vi "CF _new.vi"() -> ()   [LabVIEW 2013]
uses:
  PEM/Labview Driver, PEM100, Rev 1.2/PEM100_Visa_rev1.2.llb/HindsPEM100_Setup.ctl
  PEM/Labview Driver, PEM100, Rev 1.2/PEM100_Visa_rev1.2.llb/Com Address.ctl
  <vilib>/DAQmx/read.llb/DAQmx Read (Analog 1D DBL NChan 1Samp).vi
  <vilib>/DAQmx/write.llb/DAQmx Write (Analog 1D DBL NChan 1Samp).vi
  <vilib>/DAQmx/write.llb/DAQmx Write (Analog 2D DBL NChan NSamp).vi
  <vilib>/DAQmx/read.llb/DAQmx Read (Analog 2D DBL NChan NSamp).vi
  <vilib>/Analysis/baseanly.llb/Mean (DBL).vi
  <vilib>/DAQmx/write.llb/DAQmx Write (Analog DBL 1Chan 1Samp).vi
  <vilib>/DAQmx/read.llb/DAQmx Read (Analog 1D DBL 1Chan NSamp).vi
  <vilib>/Utility/file.llb/Read From Spreadsheet File (DBL).vi
  <vilib>/DAQmx/create/channels.llb/DAQmx Create Channel (AI-Voltage-Basic).vi
  <vilib>/DAQmx/create/channels.llb/DAQmx Create Channel (AO-Voltage-Basic).vi
  <vilib>/DAQmx/configure/timing.llb/DAQmx Timing (Sample Clock).vi
  <vilib>/DAQmx/miscellaneous.llb/DAQmx Fill In Error Info.vi
  <vilib>/DAQmx/configure/trigger.llb/DAQmx Start Trigger (Digital Edge).vi
  <vilib>/Utility/file.llb/Write To Spreadsheet File (DBL).vi
  <vilib>/measure/NI_MABase.lvlib
  <resource>/objmgr/daqmx.rc
  <vilib>/Analysis/NI_AALBase.lvlib
panel:
  in  "Static Channels":cluster{dbl, string, "Output Channels":tag}[](array[cluster])=[{1.0, "", "Output Channels"="Dev1/ao2"}, {1.0, "", "Output Channels"="Dev1/ao3"}, {1.0, "", "Output Channels"="Dev2/ao2"}, {1.0, "", "Output Channels"="Dev2/ao3"}, {0.0, "", "Output Channels"=""}, {1.0, "", "Output Channels"=""}]
  out "IR Power":dbl[][](array[numeric])=[[0.3898, 5.617e-05, 1000.0], [2.02, 0.0002739, 1010.0], [2.025, 0.0002537, 1020.0], [1.748, 0.0002412, 1030.0], [1.884, 0.0003115, 1040.0], [1.752, 0.000412, 1050.0], [2.034, 0.0004784, 1060.0], [2.031, 0.0003652, 1070.0], [2.155, 0.000355, 1080.0], [1.988, 0.0003222, 1090.0], [1.864, 0.0003151, 1100.0], [1.733, 0.000293, 1110.0], [1.546, 0.0002614, 1120.0], [1.43, 0.0002417, 1130.0], [1.423, 0.0002405, 1140.0], [1.513, 0.0002557, 1150.0], [1.694, 0.0002862, 1160.0], [1.907, 0.0003223, 1170.0], [2.124, 0.0003589, 1180.0], [2.278, 0.000385, 1190.0], [2.277, 0.0003847, 1200.0], [2.144, 0.0003621, 1210.0], [1.986, 0.0003355, 1220.0], [1.898, 0.0003205, 1230.0], [1.925, 0.0003252, 1240.0], [2.034, 0.0003435, 1250.0], [2.127, 0.0003592, 1260.0], [2.211, 0.0003733, 1270.0], [2.244, 0.0003788, 1280.0], [2.232, 0.0003768, 1290.0], [2.217, 0.0003743, 1300.0], [2.274, 0.0003838, 1310.0], [2.371, 0.0004002, 1320.0], [2.499, 0.0004217, 1330.0], [2.694, 0.0004546, 1340.0], [2.607, 0.0004399, 1350.0], [2.198, 0.0003709, 1360.0], [1.699, 0.0002866, 1370.0], [1.275, 0.0002151, 1380.0], [1.552, 0.0002617, 1390.0], [1.766, 0.0002977, 1400.0], [2.054, 0.0003464, 1410.0], [2.374, 0.0004003, 1420.0], [2.643, 0.0004456, 1430.0], [2.718, 0.0004583, 1440.0], [2.547, 0.0004293, 1450.0], [2.195, 0.00037, 1460.0], [1.875, 0.000316, 1470.0], [1.72, 0.0002899, 1480.0], [1.676, 0.0002824, 1490.0], [1.736, 0.0002925, 1500.0], [1.805, 0.0003041, 1510.0], [1.929, 0.0003249, 1520.0], [2.082, 0.0003507, 1530.0], [2.283, 0.0003845, 1540.0], [2.517, 0.0004239, 1550.0], [2.698, 0.0004544, 1560.0], [2.772, 0.0004668, 1570.0], [2.674, 0.0004501, 1580.0], [2.529, 0.0004257, 1590.0], [2.338, 0.0003936, 1600.0], [2.127, 0.000358, 1610.0], [1.947, 0.0003277, 1620.0], [1.752, 0.0002948, 1630.0], [1.552, 0.0002612, 1640.0], [1.388, 0.0002335, 1650.0], [1.207, 0.0002031, 1660.0], [1.019, 0.0001714, 1670.0], [0.9422, 0.0001585, 1680.0], [0.8635, 0.0001452, 1690.0], [0.8028, 0.000135, 1700.0], [0.7895, 0.0001328, 1710.0], [0.7496, 0.000126, 1720.0], [0.7109, 0.0001195, 1730.0], [0.6709, 0.0001128, 1740.0], [0.6361, 0.0001069, 1750.0], [0.586, 9.849e-05, 1760.0], [0.5324, 8.947e-05, 1770.0], [0.472, 7.932e-05, 1780.0], [0.4092, 6.875e-05, 1790.0], [0.3409, 5.728e-05, 1800.0]]
  out "Vis Power":dbl[][](array[numeric])=[[1.246, 2.318e-05, 400.0], [1.183, 0.0001042, 405.0], [0.7058, 0.0001228, 410.0], [0.957, 3.031e-05, 415.0], [0.9707, 5.607e-05, 420.0], [0.9509, 9.291e-05, 425.0], [0.9652, 0.0001411, 430.0], [0.9779, 0.000182, 435.0], [1.003, 0.0001974, 440.0], [1.041, 0.0002096, 445.0], [1.028, 0.0002025, 450.0], [1.052, 0.0001774, 455.0], [1.04, 0.0001549, 460.0], [1.031, 0.0001442, 465.0], [1.076, 0.0001512, 470.0], [1.072, 0.0001558, 475.0], [1.077, 0.0001726, 480.0], [1.077, 0.000155, 485.0], [1.051, 0.0001677, 490.0], [1.085, 0.0001761, 495.0], [1.075, 0.0002017, 500.0], [1.039, 0.0002081, 505.0], [1.025, 0.0002273, 510.0], [1.01, 0.0002913, 515.0], [1.017, 0.0002703, 520.0], [1.009, 0.0002942, 525.0], [0.9843, 0.0002796, 530.0], [1.004, 0.0002957, 535.0], [0.9771, 0.0003261, 540.0], [0.9818, 0.0003368, 545.0], [0.9802, 0.0003446, 550.0], [0.9463, 0.0003474, 555.0], [0.9541, 0.0003665, 560.0], [0.9389, 0.0003327, 565.0], [0.9278, 0.0003475, 570.0], [0.9343, 0.0003765, 575.0], [0.9392, 0.000404, 580.0], [0.9248, 0.0004213, 585.0], [0.9276, 0.0004463, 590.0], [0.9301, 0.0004129, 595.0], [0.938, 0.0003926, 600.0], [0.9261, 0.0004247, 605.0], [0.9214, 0.0004545, 610.0], [0.9264, 0.0004519, 615.0], [0.9205, 0.0004481, 620.0], [0.9071, 0.0004037, 625.0], [0.9085, 0.0004188, 630.0], [0.9135, 0.0004314, 635.0], [0.919, 0.0004155, 640.0], [0.9358, 0.0004483, 645.0], [0.9164, 0.0004434, 650.0], [0.9342, 0.0004245, 655.0], [0.9412, 0.0004252, 660.0], [0.9544, 0.0004259, 665.0], [0.9549, 0.0004423, 670.0], [0.9525, 0.0004703, 675.0], [0.9531, 0.0005061, 680.0], [0.9534, 0.0005373, 685.0], [0.9538, 0.0005706, 690.0], [0.9623, 0.0005955, 695.0], [0.9587, 0.0006049, 700.0], [0.9643, 0.0005917, 705.0], [0.9702, 0.0005094, 710.0], [0.9857, 0.0004327, 715.0], [0.9781, 0.0004413, 720.0], [0.9567, 0.0004771, 725.0], [0.9459, 0.0004635, 730.0], [0.9418, 0.0004453, 735.0], [0.9456, 0.0004497, 740.0], [0.9608, 0.0004574, 745.0], [0.953, 0.0004442, 750.0], [0.9723, 0.000451, 755.0], [0.9896, 0.0004518, 760.0], [0.996, 0.0004485, 765.0], [1.001, 0.0004247, 770.0], [1.007, 0.0003865, 775.0], [1.016, 0.0003508, 780.0], [1.035, 0.0003404, 785.0], [1.031, 0.0003623, 790.0], [1.027, 0.0003991, 795.0], [1.018, 0.0004293, 800.0], [1.02, 0.0004557, 805.0], [1.028, 0.0004573, 810.0], [1.023, 0.0004482, 815.0], [1.018, 0.0004471, 820.0], [1.006, 0.0004426, 825.0], [1.005, 0.0004233, 830.0], [1.01, 0.0003991, 835.0], [1.009, 0.000391, 840.0], [1.001, 0.0004016, 845.0], [0.9936, 0.0004036, 850.0], [0.9817, 0.0003871, 855.0], [0.98, 0.0003447, 860.0], [0.989, 0.0003386, 865.0], [0.9676, 0.0003372, 870.0], [0.9529, 0.0003146, 875.0], [0.96, 0.0003173, 880.0], [0.9574, 0.0002994, 885.0], [0.9534, 0.000297, 890.0], [0.9416, 0.0002885, 895.0], [0.9526, 0.0002831, 900.0], [0.9407, 0.0002601, 905.0], [0.9437, 0.000248, 910.0], [0.9327, 0.0002356, 915.0], [0.9274, 0.0002234, 920.0], [0.93, 0.0002134, 925.0], [0.9262, 0.0002018, 930.0], [0.9292, 0.0001934, 935.0], [0.937, 0.0001986, 940.0], [0.9274, 0.0002188, 945.0], [0.9187, 0.0002472, 950.0], [0.919, 0.0002798, 955.0], [0.9199, 0.0002845, 960.0], [0.9228, 0.0002559, 965.0], [0.9247, 0.0002169, 970.0], [0.9264, 0.0001847, 975.0], [0.9249, 0.0001615, 980.0], [0.9245, 0.0001469, 985.0], [0.9239, 0.0001402, 990.0], [0.9154, 0.0001357, 995.0], [0.9124, 0.0001315, 1000.0]]
  in  "Normalizing power IR":path=path "T:/Physics/Minot Group/Lee/SPCM/Power waves/2015-02-05/PowIRnewconfig"
  in  "Normalizing power visible":path=path "T:/Physics/Minot Group/Lee/SPCM/Power waves/2015-02-05/Powvis"
  out "Record Start":timestamp=timestamp(3554067343.4700146 s since 1904-01-01)
  in  "Sm Voltage offset x":dbl=0.0056
  in  "Sm voltage offset y":dbl=0.0064
  out "VNTy":dbl=-0.002731286355015208
  out "VNTx":dbl=0.0019385044089532365
  in  "Use PEM?":bool
  out "PEM delay":dbl=2.0442256927490234
  in  "PEM100Setup":T1={"Address:"=0, "Retardation:"=0.25, "RTD Units"=0, "Wavelength:"=1010.0, "Wave Units"=0} {"Address:" items=["Com 1", "Com 2", "Com 3", "Com 4", "Com 5", "Com 6", "Com 7", "Com 8", "Com 9", "Com 10"]; "Wave Units" items=["nm", "um", "cm-1"]; "RTD Units" items=["waves", "Radians", "Degrees"]; "Wavelength:" min=0.0 max=19999.9 step=0.1 format="%.1f"; "Retardation:" min=0.0 max=10.0 step=0.001 format="%.3f"}
  in  "Scan base":path=path "T:/Physics/Minot Group/Lee/SPCM"
  in  "Prepend date folder?":bool=TRUE
  in  "Subfolder(no outside slashes)":string
  in  "Volts/pixel y":dbl=-0.041
  in  "Volts/pixel  x":dbl=0.041
  out "String":string="IR Grating"
  in  "IR Grating Correction":dbl[][](array[numeric])=[[1000.0, 0.0, 0.0], [1100.0, 0.0, -0.06], [1200.0, -0.01, 0.06], [1300.0, 0.06, 0.02], [1400.0, -0.05, 0.05], [1500.0, 0.0, 0.0], [1600.0, 0.0, 0.0], [1700.0, 0.0, 0.0], [1800.0, 0.0, 0.0]]
  in  "Reset Positioned wavelength?":bool
  out "Done?":string="  ok\r\n"
  out "Busy?":bool
  out "Reply":string=" 619.990 nm  ok\r\n" caption="Mono Response"
  in  "Speed (nm/min)":dbl=100.0 min=1.0 max=500.0 step=0.1 format="%.1f"
  in  "Wavelength:":dbl=620.0 caption="nm" min=0.0 max=2000.0 step=0.1 format="%.1f"
  in  "Positioned Wavelength":dbl=1600.0
  in  "Sm Correction?":bool=TRUE
  out "Delta Pix y":dbl=-0.006
  out "delta pix x":dbl
  in  "Power Meter Initalized?":bool
  out "Multiplication Factor":dbl=1e-09
  in  "Preamp Sensitivity":T3(ring)=enum."1nA/V"
  in  "Configuration":T4(ring)=enum."Preamp"
  in  "Multiply Data?":bool=TRUE
  out "Waveform Chart  Y":dbl[](graph)=[-0.006278594561464471, -0.0062748012532580204, -0.006271007945051572, -0.006267214636845122, -0.0062634213286386735, -0.006259628020432223, -0.006255834712225775, -0.006252041404019325, -0.006248248095812876, -0.006244454787606426, -0.006240661479399978, -0.006236868171193528, -0.006233074862987079, -0.006229281554780629, -0.006225488246574181, -0.006221694938367731, -0.006217901630161282, -0.006214108321954833, -0.006210315013748384, -0.006206521705541934, -0.006202728397335485, -0.006198935089129036, -0.0061951417809225865, -0.006191348472716137, -0.006187555164509688, -0.006183761856303239, -0.006179968548096789, -0.00617617523989034, -0.006172381931683891, -0.006168588623477442, -0.006164795315270992, -0.006161002007064543, -0.006157208698858094, -0.0061534153906516445, -0.006149622082445195, -0.006145828774238746, -0.006142035466032297, -0.006138242157825847, -0.006134448849619398, -0.006130655541412949, -0.0061268622332064995, -0.00612306892500005, -0.006119275616793601, -0.006115482308587152, -0.006111689000380702, -0.006107895692174253, -0.006104102383967804, -0.006100309075761355, -0.006096515767554905, -0.006092722459348457, -0.006088929151142007, -0.0060851358429355575, -0.006081342534729108, -0.006077549226522659, -0.00607375591831621, -0.00606996261010976, -0.006066169301903311, -0.006062375993696862, -0.0060585826854904126, -0.006054789377283963, -0.006050996069077514, -0.006047202760871065, -0.0060434094526646154, -0.006039616144458167, -0.006035822836251717, -0.0060320295280452685, -0.006028236219838819, -0.00602444291163237, -0.006020649603425921, -0.006016856295219471, -0.006013062987013022, -0.006009269678806573, -0.0060054763706001235, -0.006001683062393674, -0.005997889754187225, -0.005994096445980776, -0.005990303137774326, -0.005986509829567877, -0.005982716521361427, -0.005978923213154979, -0.005975129904948529, -0.00597133659674208, -0.005967543288535631, -0.0059637499803291815, -0.005959956672122732, -0.005956163363916283, -0.005952370055709834, -0.005948576747503384, -0.005944783439296935, -0.005940990131090486, -0.005937196822884037, -0.005933403514677587, -0.005929610206471138, -0.005925816898264689, -0.0059220235900582395, -0.00591823028185179, -0.005914436973645341, -0.005910643665438892, -0.005906850357232442, -0.005903057049025993, -0.005899263740819544, -0.0058954704326130945, -0.005891677124406645, -0.005887883816200196, -0.005884090507993747, -0.005880297199787297, -0.005876503891580848, -0.005872710583374399, -0.00586891727516795, -0.0058651239669615, -0.005861330658755051, -0.005857537350548602, -0.005853744042342153, -0.005849950734135703, -0.005846157425929255, -0.005842364117722805, -0.005838570809516356, -0.005834777501309906, -0.005830984193103458, -0.0058271908848970076, -0.005823397576690559, -0.005819604268484109, -0.005815810960277661, -0.0058120176520712104, -0.005808224343864761, -0.005804431035658312, -0.005800637727451863, -0.005796844419245413, -0.005793051111038965, -0.005789257802832515, -0.005785464494626066, -0.005781671186419617, -0.005777877878213168, -0.0057740845700067185, -0.005770291261800269, -0.00576649795359382, -0.005762704645387371, -0.0057589113371809214, -0.005755118028974472, -0.005751324720768023, -0.005747531412561574, -0.005743738104355124, -0.005739944796148675, -0.005736151487942226, -0.0057323581797357765, -0.005728564871529327, -0.005724771563322878, -0.005720978255116429, -0.005717184946909979, -0.00571339163870353, -0.005709598330497081, -0.005705805022290632, -0.005702011714084182, -0.005698218405877733, -0.005694425097671284, -0.0056906317894648345, -0.005686838481258385, -0.005683045173051936, -0.005679251864845487, -0.005675458556639037, -0.005671665248432588, -0.005667871940226139, -0.0056640786320196895, -0.00566028532381324, -0.005656492015606791, -0.005652698707400342, -0.005648905399193892, -0.005645112090987443, -0.005641318782780994, -0.005637525474574545, -0.005633732166368095, -0.005629938858161646, -0.005626145549955197, -0.0056223522417487475, -0.005618558933542298, -0.005614765625335849, -0.0056109723171294, -0.005607179008922951, -0.005603385700716501, -0.005599592392510053, -0.0055957990843036026, -0.005592005776097154, -0.005588212467890704, -0.005584419159684256, -0.0055806258514778054, -0.005576832543271357, -0.005573039235064907, -0.0055692459268584585, -0.005565452618652008, -0.00556165931044556, -0.00555786600223911, -0.005554072694032661, -0.005550279385826211, -0.005546486077619763, -0.0055426927694133135, -0.005538899461206864, -0.005535106153000415, -0.005531312844793966, -0.0055275195365875164, -0.005523726228381067, -0.005519932920174618, -0.005516139611968169, -0.005512346303761719, -0.00550855299555527, -0.005504759687348821, -0.0055009663791423715, -0.005497173070935922, -0.005493379762729473, -0.005489586454523024, -0.005485793146316574, -0.005481999838110125, -0.005478206529903676, -0.005474413221697227, -0.005470619913490777, -0.005466826605284328, -0.005463033297077879, -0.0054592399888714295, -0.00545544668066498, -0.005451653372458531, -0.005447860064252082, -0.005444066756045632, -0.005440273447839183, -0.005436480139632734, -0.0054326868314262845, -0.005428893523219835, -0.005425100215013386, -0.005421306906806937, -0.005417513598600487, -0.005413720290394039, -0.005409926982187589, -0.00540613367398114, -0.00540234036577469, -0.005398547057568242, -0.005394753749361792, -0.0053909604411553425, -0.005387167132948893, -0.005383373824742445, -0.005379580516535995, -0.005375787208329545, -0.005371993900123096, -0.005368200591916648, -0.0053644072837101976, -0.005360613975503749, -0.005356820667297299, -0.005353027359090851, -0.005349234050884401, -0.005345440742677952, -0.005341647434471502, -0.005337854126265053, -0.005334060818058604, -0.005330267509852155, -0.005326474201645705, -0.0053226808934392555, -0.005318887585232807, -0.005315094277026358, -0.0053113009688199085, -0.005307507660613458, -0.00530371435240701, -0.005299921044200561, -0.0052961277359941114, -0.005292334427787662, -0.005288541119581213, -0.005284747811374764, -0.005280954503168314, -0.005277161194961865, -0.005273367886755416, -0.0052695745785489665, -0.005265781270342517, -0.005261987962136068, -0.005258194653929619, -0.005254401345723169, -0.00525060803751672, -0.005246814729310271, -0.005243021421103822, -0.005239228112897372, -0.005235434804690923, -0.005231641496484474, -0.0052278481882780245, -0.005224054880071575, -0.005220261571865126, -0.005216468263658677, -0.005212674955452227, -0.005208881647245778, -0.005205088339039329, -0.0052012950308328795, -0.00519750172262643, -0.005193708414419981, -0.005189915106213532, -0.005186121798007082, -0.005182328489800633, -0.005178535181594185, -0.005174741873387735, -0.005170948565181285, -0.005167155256974836, -0.005163361948768388, -0.005159568640561938, -0.005155775332355488, -0.005151982024149039, -0.00514818871594259, -0.005144395407736141, -0.005140602099529691, -0.005136808791323242, -0.0051330154831167926, -0.005129222174910344, -0.005125428866703894, -0.005121635558497445, -0.0051178422502909954, -0.005114048942084547, -0.005110255633878098, -0.0051064623256716485, -0.005102669017465198, -0.00509887570925875, -0.005095082401052301, -0.005091289092845851, -0.005087495784639401, -0.005083702476432953, -0.0050799091682265035, -0.005076115860020054, -0.005072322551813604, -0.005068529243607156, -0.0050647359354007064, -0.005060942627194257, -0.005057149318987808, -0.005053356010781359, -0.005049562702574909, -0.00504576939436846, -0.005041976086162011, -0.0050381827779555615, -0.005034389469749112, -0.005030596161542663, -0.005026802853336214, -0.005023009545129764, -0.005019216236923315, -0.005015422928716866, -0.005011629620510417, -0.005007836312303967, -0.005004043004097518, -0.005000249695891069, -0.0049964563876846195, -0.00499266307947817, -0.004988869771271721, -0.004985076463065272, -0.004981283154858822, -0.004977489846652373, -0.004973696538445925, -0.0049699032302394745, -0.004966109922033025, -0.004962316613826576, -0.004958523305620127, -0.004954729997413677, -0.004950936689207228, -0.004947143381000779, -0.00494335007279433, -0.00493955676458788, -0.004935763456381431, -0.004931970148174982, -0.0049281768399685325, -0.004924383531762084, -0.004920590223555635, -0.004916796915349185, -0.004913003607142735, -0.004909210298936287, -0.004905416990729838, -0.0049016236825233876, -0.004897830374316938, -0.00489403706611049, -0.004890243757904041, -0.0048864504496975904, -0.004882657141491141, -0.004878863833284693, -0.0048750705250782435, -0.004871277216871794, -0.004867483908665345, -0.004863690600458895, -0.004859897292252446, -0.004856103984045997, -0.004852310675839548, -0.004848517367633098, -0.004844724059426649, -0.0048409307512202, -0.004837137443013751, -0.004833344134807301, -0.004829550826600852, -0.004825757518394403, -0.004821964210187954, -0.004818170901981504, -0.004814377593775055, -0.004810584285568606, -0.0048067909773621565, -0.004802997669155707, -0.004799204360949258, -0.004795411052742809, -0.004791617744536359, -0.00478782443632991, -0.004784031128123461, -0.004780237819917012, -0.004776444511710562, -0.004772651203504113, -0.004768857895297664, -0.0047650645870912145, -0.004761271278884765, -0.004757477970678316, -0.004753684662471867, -0.004749891354265417, -0.004746098046058968, -0.004742304737852519, -0.0047385114296460695, -0.004734718121439621, -0.004730924813233171, -0.004727131505026722, -0.004723338196820272, -0.004719544888613824, -0.004715751580407374, -0.004711958272200925, -0.004708164963994475, -0.004704371655788027, -0.004700578347581577, -0.0046967850393751275, -0.004692991731168678, -0.00468919842296223, -0.0046854051147557805, -0.004681611806549331, -0.004677818498342881, -0.004674025190136432, -0.004670231881929983, -0.004666438573723534, -0.004662645265517084, -0.004658851957310635, -0.004655058649104186, -0.004651265340897737, -0.004647472032691287, -0.004643678724484838, -0.004639885416278389, -0.00463609210807194, -0.004632298799865491, -0.0046285054916590405, -0.004624712183452592, -0.004620918875246143, -0.0046171255670396935, -0.004613332258833244, -0.004609538950626795, -0.004605745642420346, -0.0046019523342138964, -0.004598159026007447, -0.004594365717800998, -0.004590572409594549, -0.004586779101388099, -0.00458298579318165, -0.004579192484975201, -0.0045753991767687515, -0.004571605868562302, -0.004567812560355853, -0.004564019252149404, -0.004560225943942954, -0.004556432635736505, -0.004552639327530056, -0.004548846019323607, -0.004545052711117157, -0.004541259402910708, -0.004537466094704259, -0.0045336727864978095, -0.00452987947829136, -0.004526086170084911, -0.004522292861878462, -0.004518499553672012, -0.004514706245465564, -0.004510912937259114, -0.0045071196290526645, -0.004503326320846215, -0.004499533012639766, -0.004495739704433317, -0.004491946396226867, -0.004488153088020418, -0.004484359779813969, -0.0044805664716075205, -0.00447677316340107, -0.004472979855194621, -0.004469186546988172, -0.004465393238781723, -0.004461599930575273, -0.004457806622368824, -0.004454013314162375, -0.004450220005955926, -0.004446426697749477, -0.004442633389543027, -0.0044388400813365776, -0.004435046773130129, -0.00443125346492368, -0.004427460156717231, -0.0044236668485107804, -0.004419873540304332, -0.004416080232097883, -0.0044122869238914335, -0.004408493615684983, -0.004404700307478534, -0.004400906999272086, -0.004397113691065636, -0.004393320382859187, -0.004389527074652737, -0.0043857337664462885, -0.004381940458239839, -0.00437814715003339, -0.004374353841826941, -0.0043705605336204914, -0.004366767225414042, -0.004362973917207593, -0.004359180609001144, -0.004355387300794694, -0.004351593992588245, -0.004347800684381796, -0.0043440073761753465, -0.004340214067968897, -0.004336420759762448, -0.004332627451555999, -0.004328834143349549, -0.004325040835143101, -0.004321247526936651, -0.004317454218730202, -0.004313660910523752, -0.004309867602317303, -0.004306074294110854, -0.0043022809859044045, -0.004298487677697955, -0.004294694369491506, -0.0042909010612850575, -0.004287107753078607, -0.004283314444872158, -0.004279521136665709, -0.00427572782845926, -0.004271934520252811, -0.004268141212046361, -0.004264347903839912, -0.004260554595633463, -0.004256761287427014, -0.004252967979220564, -0.004249174671014115, -0.004245381362807666, -0.004241588054601217, -0.004237794746394768, -0.0042340014381883175, -0.004230208129981869, -0.00422641482177542, -0.0042226215135689705, -0.004218828205362521, -0.004215034897156071, -0.004211241588949623, -0.004207448280743173, -0.004203654972536724, -0.004199861664330274, -0.004196068356123826, -0.004192275047917376, -0.004188481739710927, -0.004184688431504478, -0.0041808951232980285, -0.004177101815091579, -0.00417330850688513, -0.004169515198678681, -0.004165721890472231, -0.004161928582265782, -0.004158135274059333, -0.0041543419658528835, -0.004150548657646434, -0.004146755349439985, -0.004142962041233536, -0.0041391687330270864, -0.004135375424820637, -0.004131582116614188, -0.004127788808407739, -0.004123995500201289, -0.00412020219199484, -0.004116408883788391, -0.0041126155755819415, -0.004108822267375492, -0.004105028959169043, -0.004101235650962594, -0.004097442342756144, -0.004093649034549695, -0.004089855726343246, -0.0040860624181367974, -0.004082269109930347, -0.004078475801723898, -0.004074682493517449, -0.004070889185311, -0.00406709587710455, -0.004063302568898101, -0.004059509260691652, -0.004055715952485203, -0.004051922644278754, -0.004048129336072304, -0.0040443360278658545, -0.004040542719659406, -0.004036749411452957, -0.0040329561032465076, -0.004029162795040057, -0.004025369486833608, -0.00402157617862716, -0.0040177828704207105, -0.00401398956221426, -0.004010196254007811, -0.004006402945801363, -0.004002609637594913, -0.003998816329388464, -0.003995023021182014, -0.0039912297129755655, -0.003987436404769116, -0.003983643096562667, -0.003979849788356218, -0.003976056480149768, -0.003972263171943319, -0.00396846986373687, -0.003964676555530421, -0.003960883247323971, -0.003957089939117522, -0.003953296630911073, -0.0039495033227046235, -0.003945710014498174, -0.003941916706291725, -0.003938123398085276, -0.003934330089878826, -0.003930536781672377, -0.003926743473465928, -0.0039229501652594785, -0.003919156857053029, -0.00391536354884658, -0.003911570240640131, -0.0039077769324336814, -0.003903983624227232, -0.003900190316020783, -0.003896397007814334, -0.0038926036996078843, -0.003888810391401435, -0.0038850170831949858, -0.003881223774988537, -0.0038774304667820872, -0.003873637158575638, -0.0038698438503691887, -0.00386605054216274, -0.0038622572339562906, -0.003858463925749841, -0.0038546706175433916, -0.0038508773093369427, -0.0038470840011304934, -0.003843290692924044, -0.0038394973847175945, -0.003835704076511145, -0.0038319107683046963, -0.003828117460098247, -0.0038243241518917974, -0.003820530843685348, -0.0038167375354788992, -0.00381294422727245, -0.0038091509190660007, -0.003805357610859551, -0.0038015643026531026, -0.003797770994446653, -0.0037939776862402036, -0.0037901843780337543, -0.0037863910698273055, -0.003782597761620856, -0.0037788044534144065, -0.003775011145207957, -0.0037712178370015084, -0.003767424528795059, -0.0037636312205886094, -0.00375983791238216, -0.0037560446041757112, -0.003752251295969262, -0.0037484579877628127, -0.003744664679556363, -0.0037408713713499137, -0.003737078063143465, -0.0037332847549370156, -0.0037294914467305663, -0.0037256981385241166, -0.0037219048303176678, -0.0037181115221112185, -0.003714318213904769, -0.0037105249056983195, -0.0037067315974918707, -0.0037029382892854214, -0.003699144981078972, -0.003695351672872523, -0.0036915583646660735, -0.0036877650564596243, -0.003683971748253175, -0.0036801784400467257, -0.003676385131840277, -0.003672591823633827, -0.003668798515427378, -0.0036650052072209286, -0.0036612118990144798, -0.0036574185908080305, -0.0036536252826015808, -0.0036498319743951315, -0.0036460386661886822, -0.0036422453579822334, -0.0036384520497757837, -0.0036346587415693344, -0.003630865433362885, -0.0036270721251564363, -0.003623278816949987, -0.0036194855087435373, -0.003615692200537088, -0.003611898892330639, -0.00360810558412419, -0.0036043122759177406, -0.003600518967711291, -0.0035967256595048425, -0.003592932351298393, -0.0035891390430919435, -0.003585345734885494, -0.0035815524266790454, -0.0035777591184725957, -0.0035739658102661464, -0.003570172502059697, -0.0035663791938532483, -0.003562585885646799, -0.0035587925774403493, -0.0035549992692339, -0.0035512059610274503, -0.003547412652821002, -0.0035436193446145526, -0.003539826036408103, -0.0035360327282016536, -0.003532239419995205, -0.0035284461117887555, -0.003524652803582306, -0.0035208594953758565, -0.0035170661871694077, -0.0035132728789629584, -0.003509479570756509, -0.0035056862625500594, -0.0035018929543436106, -0.0034980996461371613, -0.003494306337930712, -0.0034905130297242623, -0.0034867197215178135, -0.003482926413311364, -0.003479133105104915, -0.0034753397968984657, -0.003471546488692017, -0.003467753180485567, -0.003463959872279118, -0.0034601665640726685, -0.0034563732558662193, -0.00345257994765977, -0.0034487866394533207, -0.0034449933312468714, -0.003441200023040422, -0.0034374067148339733, -0.0034336134066275236, -0.0034298200984210743, -0.003426026790214625, -0.003422233482008176, -0.0034184401738017265, -0.0034146468655952772, -0.003410853557388828, -0.003407060249182379, -0.00340326694097593, -0.00339947363276948, -0.003395680324563031, -0.0033918870163565824, -0.0033880937081501327, -0.003384300399943683, -0.0033805070917372337, -0.0033767137835307845, -0.0033729204753243356, -0.0033691271671178863, -0.0033653338589114366, -0.0033615405507049874, -0.003357747242498539, -0.0033539539342920892, -0.00335016062608564, -0.0033463673178791902, -0.003342574009672742, -0.0033387807014662926, -0.003334987393259843, -0.003331194085053393, -0.0033274007768469447, -0.0033236074686404955, -0.0033198141604340457, -0.0033160208522275965, -0.0033122275440211476, -0.0033084342358146984, -0.003304640927608249, -0.0033008476194017994, -0.0032970543111953505, -0.0032932610029889012, -0.003289467694782452, -0.0032856743865760023, -0.003281881078369553, -0.003278087770163104, -0.003274294461956655, -0.0032705011537502056, -0.003266707845543756, -0.003262914537337307, -0.0032591212291308578, -0.0032553279209244085, -0.003251534612717959, -0.00324774130451151, -0.0032439479963050607, -0.0032401546880986114, -0.003236361379892162, -0.003232568071685713, -0.0032287747634792635, -0.0032249814552728143, -0.003221188147066365, -0.003217394838859916, -0.0032136015306534664, -0.003209808222447017, -0.003206014914240568, -0.003202221606034119, -0.0031984282978276693, -0.00319463498962122, -0.0031908416814147708, -0.0031870483732083215, -0.0031832550650018727, -0.003179461756795423, -0.0031756684485889737, -0.0031718751403825244, -0.0031680818321760756, -0.0031642885239696263, -0.0031604952157631766, -0.0031567019075567273, -0.0031529085993502784, -0.003149115291143829, -0.0031453219829373795, -0.00314152867473093, -0.0031377353665244818, -0.003133942058318032, -0.003130148750111583, -0.003126355441905133, -0.0031225621336986847, -0.0031187688254922354, -0.0031149755172857857, -0.003111182209079336, -0.0031073889008728876, -0.0031035955926664383, -0.0030998022844599886, -0.0030960089762535393, -0.0030922156680470896, -0.003088422359840641, -0.003084629051634192, -0.003080835743427742, -0.003077042435221293, -0.003073249127014844, -0.003069455818808395, -0.0030656625106019455, -0.003061869202395496, -0.003058075894189047, -0.0030542825859825977, -0.0030504892777761484, -0.0030466959695696987, -0.00304290266136325, -0.0030391093531568006, -0.0030353160449503513, -0.003031522736743902, -0.0030277294285374528, -0.0030239361203310035, -0.003020142812124554, -0.003016349503918105, -0.0030125561957116557, -0.0030087628875052064, -0.003004969579298757, -0.003001176271092308, -0.0029973829628858585, -0.0029935896546794093, -0.00298979634647296, -0.0029860030382665107, -0.0029822097300600614, -0.002978416421853612, -0.002974623113647163, -0.0029708298054407136, -0.0029670364972342643, -0.0029632431890278155, -0.0029594498808213658, -0.0029556565726149165, -0.0029518632644084672, -0.0029480699562020184, -0.002944276647995569, -0.0029404833397891194, -0.00293669003158267, -0.0029328967233762217, -0.002929103415169772, -0.0029253101069633223, -0.002921516798756873, -0.0029177234905504246, -0.002913930182343975, -0.0029101368741375256, -0.002906343565931076, -0.0029025502577246266, -0.0028987569495181782, -0.0028949636413117285, -0.0028911703331052792, -0.0028873770248988295, -0.002883583716692381, -0.002879790408485932, -0.002875997100279482, -0.0028722037920730324, -0.002868410483866584, -0.0028646171756601347, -0.002860823867453685, -0.0028570305592472357, -0.002853237251040787, -0.0028494439428343376, -0.0028456506346278884, -0.0028418573264214386, -0.00283806401821499, -0.0028342707100085405, -0.0028304774018020912, -0.002826684093595642, -0.0028228907853891927, -0.0028190974771827434, -0.002815304168976294, -0.002811510860769845, -0.002807717552563395, -0.0028039242443569463, -0.002800130936150497, -0.0027963376279440478, -0.0027925443197375985, -0.002788751011531149, -0.0027849577033247, -0.0027811643951182506, -0.002777371086911802, -0.002773577778705352, -0.002769784470498903, -0.0027659911622924535, -0.0027621978540860043, -0.002758404545879555, -0.0027546112376731053, -0.0027508179294666573, -0.002747024621260208, -0.0027432313130537583, -0.0027394380048473086, -0.0027356446966408593, -0.00273185138843441, -0.0027280580802279608, -0.0027242647720215115, -0.002720471463815062, -0.002716678155608614, -0.0027128848474021645, -0.002709091539195715, -0.0027052982309892656, -0.002701504922782816, -0.0026977116145763666, -0.0026939183063699173, -0.002690124998163468, -0.0026863316899570196, -0.0026825383817505703, -0.002678745073544121, -0.0026749517653376713, -0.002671158457131222, -0.0026673651489247724, -0.002663571840718323, -0.002659778532511874, -0.0026559852243054254, -0.002652191916098976, -0.002648398607892527, -0.0026446052996860776, -0.002640811991479628, -0.0026370186832731786, -0.002633225375066729, -0.0026294320668602796, -0.0026256387586538303, -0.002621845450447382, -0.0026180521422409326, -0.0026142588340344834, -0.002610465525828034, -0.002606672217621585, -0.002602878909415135, -0.0025990856012086854, -0.002595292293002236, -0.002591498984795788, -0.0025877056765893384, -0.002583912368382889, -0.00258011906017644, -0.0025763257519699906, -0.0025725324437635413, -0.0025687391355570916, -0.0025649458273506423, -0.0025611525191441943, -0.0025573592109377446, -0.002553565902731295, -0.0025497725945248456, -0.0025459792863183964, -0.002542185978111947, -0.002538392669905498, -0.002534599361699048, -0.002530806053492599, -0.002527012745286151, -0.002523219437079701, -0.002519426128873252, -0.002515632820666802, -0.002511839512460353, -0.0025080462042539036, -0.0025042528960474543, -0.002500459587841005, -0.0024966662796345566, -0.0024928729714281074, -0.0024890796632216577]
  out "Final Y":dbl=-0.0024890796632216577
  out "initial y":dbl=-0.006278594561464471
  out "Waveform Chart X":dbl[](graph)=[-0.005478594561464469, -0.005471177462494051, -0.005463760363523634, -0.005456343264553216, -0.005448926165582799, -0.00544150906661238, -0.005434091967641963, -0.0054266748686715455, -0.005419257769701128, -0.00541184067073071, -0.005404423571760292, -0.005397006472789874, -0.0053895893738194565, -0.005382172274849039, -0.005374755175878621, -0.005367338076908203, -0.005359920977937786, -0.005352503878967368, -0.005345086779996951, -0.005337669681026533, -0.005330252582056116, -0.005322835483085698, -0.00531541838411528, -0.005308001285144862, -0.0053005841861744445, -0.005293167087204027, -0.005285749988233609, -0.005278332889263191, -0.005270915790292773, -0.005263498691322355, -0.005256081592351938, -0.00524866449338152, -0.005241247394411102, -0.005233830295440685, -0.005226413196470267, -0.00521899609749985, -0.005211578998529432, -0.005204161899559015, -0.005196744800588597, -0.005189327701618179, -0.005181910602647761, -0.005174493503677343, -0.005167076404706926, -0.005159659305736508, -0.00515224220676609, -0.005144825107795672, -0.005137408008825254, -0.005129990909854837, -0.005122573810884419, -0.005115156711914002, -0.005107739612943584, -0.005100322513973166, -0.005092905415002748, -0.0050854883160323305, -0.0050780712170619136, -0.005070654118091496, -0.005063237019121078, -0.00505581992015066, -0.005048402821180242, -0.0050409857222098245, -0.005033568623239407, -0.005026151524268989, -0.005018734425298571, -0.005011317326328153, -0.005003900227357736, -0.004996483128387318, -0.004989066029416901, -0.004981648930446483, -0.004974231831476066, -0.004966814732505647, -0.00495939763353523, -0.0049519805345648125, -0.004944563435594395, -0.004937146336623977, -0.004929729237653559, -0.004922312138683141, -0.004914895039712723, -0.004907477940742306, -0.004900060841771888, -0.00489264374280147, -0.004885226643831052, -0.004877809544860635, -0.0048703924458902165, -0.0048629753469198, -0.004855558247949382, -0.004848141148978965, -0.004840724050008546, -0.004833306951038129, -0.004825889852067711, -0.004818472753097294, -0.004811055654126876, -0.004803638555156458, -0.00479622145618604, -0.004788804357215622, -0.0047813872582452045, -0.004773970159274788, -0.004766553060304369, -0.004759135961333952, -0.004751718862363534, -0.0047443017633931155, -0.0047368846644226985, -0.004729467565452281, -0.004722050466481864, -0.004714633367511445, -0.004707216268541028, -0.00469979916957061, -0.0046923820706001925, -0.004684964971629775, -0.004677547872659357, -0.004670130773688939, -0.004662713674718521, -0.0046552965757481034, -0.004647879476777686, -0.004640462377807268, -0.004633045278836851, -0.004625628179866433, -0.004618211080896016, -0.0046107939819255974, -0.0046033768829551805, -0.004595959783984763, -0.004588542685014345, -0.004581125586043927, -0.004573708487073509, -0.004566291388103091, -0.004558874289132674, -0.004551457190162256, -0.004544040091191838, -0.00453662299222142, -0.004529205893251002, -0.0045217887942805846, -0.004514371695310167, -0.00450695459633975, -0.004499537497369332, -0.004492120398398915, -0.004484703299428496, -0.004477286200458079, -0.004469869101487662, -0.004462452002517244, -0.004455034903546826, -0.004447617804576408, -0.00444020070560599, -0.0044327836066355725, -0.004425366507665155, -0.004417949408694737, -0.004410532309724319, -0.004403115210753902, -0.0043956981117834835, -0.0043882810128130665, -0.004380863913842649, -0.004373446814872231, -0.004366029715901813, -0.004358612616931395, -0.004351195517960978, -0.0043437784189905605, -0.004336361320020143, -0.004328944221049725, -0.004321527122079307, -0.004314110023108889, -0.0043066929241384715, -0.004299275825168054, -0.004291858726197636, -0.004284441627227218, -0.004277024528256801, -0.004269607429286382, -0.0042621903303159655, -0.004254773231345548, -0.004247356132375131, -0.004239939033404712, -0.004232521934434295, -0.004225104835463877, -0.0042176877364934594, -0.004210270637523042, -0.004202853538552624, -0.004195436439582206, -0.004188019340611788, -0.00418060224164137, -0.004173185142670953, -0.004165768043700535, -0.004158350944730117, -0.0041509338457597, -0.004143516746789281, -0.004136099647818864, -0.0041286825488484466, -0.00412126544987803, -0.004113848350907611, -0.004106431251937194, -0.004099014152966776, -0.004091597053996358, -0.0040841799550259406, -0.004076762856055523, -0.004069345757085105, -0.004061928658114687, -0.004054511559144269, -0.004047094460173852, -0.004039677361203434, -0.004032260262233017, -0.004024843163262599, -0.004017426064292182, -0.004010008965321763, -0.0040025918663513455, -0.0039951747673809285, -0.00398775766841051, -0.003980340569440093, -0.003972923470469675, -0.003965506371499257, -0.0039580892725288395, -0.003950672173558422, -0.003943255074588004, -0.003935837975617586, -0.003928420876647168, -0.00392100377767675, -0.003913586678706333, -0.0039061695797359157, -0.003898752480765498, -0.0038913353817950796, -0.003883918282824663, -0.003876501183854245, -0.003869084084883827, -0.0038616669859134088, -0.0038542498869429923, -0.003846832787972574, -0.003839415689002156, -0.003831998590031738, -0.00382458149106132, -0.003817164392090903, -0.0038097472931204854, -0.003802330194150067, -0.0037949130951796493, -0.0037874959962092324, -0.0037800788972388146, -0.0037726617982683968, -0.0037652446992979785, -0.0037578276003275616, -0.0037504105013571438, -0.003742993402386726, -0.0037355763034163077, -0.003728159204445891, -0.003720742105475473, -0.003713325006505055, -0.0037059079075346373, -0.0036984908085642204, -0.003691073709593802, -0.0036836566106233843, -0.003676239511652966, -0.003668822412682549, -0.0036614053137121313, -0.0036539882147417135, -0.0036465711157712957, -0.0036391540168008774, -0.003631736917830461, -0.0036243198188600427, -0.0036169027198896244, -0.0036094856209192066, -0.0036020685219487897, -0.003594651422978372, -0.003587234324007954, -0.0035798172250375362, -0.0035724001260671193, -0.003564983027096701, -0.0035575659281262832, -0.003550148829155865, -0.003542731730185448, -0.0035353146312150302, -0.0035278975322446124, -0.0035204804332741946, -0.0035130633343037777, -0.00350564623533336, -0.0034982291363629416, -0.0034908120373925234, -0.003483394938422107, -0.0034759778394516886, -0.003468560740481271, -0.003461143641510853, -0.0034537265425404347, -0.0034463094435700182, -0.0034388923445996, -0.0034314752456291817, -0.003424058146658764, -0.003416641047688347, -0.003409223948717929, -0.0034018068497475113, -0.0033943897507770935, -0.0033869726518066766, -0.0033795555528362588, -0.0033721384538658405, -0.0033647213548954223, -0.0033573042559250058, -0.0033498871569545875, -0.0033424700579841697, -0.003335052959013752, -0.003327635860043335, -0.003320218761072917, -0.003312801662102499, -0.0033053845631320806, -0.003297967464161664, -0.003290550365191246, -0.003283133266220828, -0.0032757161672504103, -0.0032682990682799925, -0.0032608819693095755, -0.0032534648703391577, -0.0032460477713687395, -0.003238630672398321, -0.0032312135734279047, -0.0032237964744574864, -0.0032163793754870686, -0.003208962276516651, -0.003201545177546234, -0.003194128078575816, -0.003186710979605398, -0.0031792938806349796, -0.003171876781664563, -0.003164459682694145, -0.003157042583723727, -0.003149625484753309, -0.0031422083857828922, -0.0031347912868124744, -0.003127374187842056, -0.0031199570888716384, -0.0031125399899012214, -0.003105122890930803, -0.0030977057919603854, -0.0030902886929899676, -0.0030828715940195497, -0.003075454495049133, -0.003068037396078715, -0.0030606202971082967, -0.0030532031981378785, -0.003045786099167462, -0.0030383690001970437, -0.003030951901226626, -0.003023534802256208, -0.003016117703285791, -0.0030087006043153734, -0.003001283505344955, -0.0029938664063745373, -0.0029864493074041203, -0.002979032208433702, -0.0029716151094632843, -0.0029641980104928665, -0.0029567809115224495, -0.0029493638125520317, -0.002941946713581614, -0.0029345296146111957, -0.002927112515640779, -0.002919695416670361, -0.0029122783176999427, -0.002904861218729525, -0.002897444119759107, -0.00289002702078869, -0.0028826099218182723, -0.002875192822847854, -0.0028677757238774358, -0.0028603586249070193, -0.002852941525936601, -0.002845524426966183, -0.0028381073279957654, -0.0028306902290253485, -0.0028232731300549306, -0.002815856031084513, -0.0028084389321140946, -0.0028010218331436776, -0.00279360473417326, -0.0027861876352028416, -0.0027787705362324238, -0.002771353437262007, -0.002763936338291589, -0.002756519239321171, -0.002749102140350753, -0.0027416850413803364, -0.002734267942409918, -0.0027268508434395, -0.002719433744469082, -0.0027120166454986643, -0.0027045995465282474, -0.0026971824475578296, -0.0026897653485874113, -0.0026823482496169935, -0.0026749311506465766, -0.0026675140516761587, -0.0026600969527057405, -0.0026526798537353227, -0.0026452627547649057, -0.002637845655794488, -0.00263042855682407, -0.002623011457853652, -0.002615594358883235, -0.002608177259912817, -0.002600760160942399, -0.002593343061971981, -0.002585925963001564, -0.0025785088640311463, -0.0025710917650607285, -0.0025636746660903102, -0.0025562575671198937, -0.0025488404681494755, -0.0025414233691790577, -0.0025340062702086394, -0.0025265891712382216, -0.0025191720722678047, -0.002511754973297387, -0.002504337874326969, -0.002496920775356551, -0.002489503676386134, -0.002482086577415716, -0.002474669478445298, -0.00246725237947488, -0.002459835280504463, -0.0024524181815340452, -0.0024450010825636274, -0.002437583983593209, -0.0024301668846227927, -0.0024227497856523744, -0.0024153326866819566, -0.0024079155877115383, -0.0024004984887411214, -0.0023930813897707036, -0.0023856642908002858, -0.0023782471918298675, -0.002370830092859451, -0.0023634129938890328, -0.002355995894918615, -0.0023485787959481967, -0.002341161696977779, -0.002333744598007362, -0.002326327499036944, -0.0023189104000665263, -0.002311493301096108, -0.0023040762021256916, -0.0022966591031552733, -0.0022892420041848555, -0.0022818249052144373, -0.0022744078062440203, -0.0022669907072736025, -0.0022595736083031847, -0.0022521565093327665, -0.00224473941036235, -0.0022373223113919317, -0.002229905212421514, -0.0022224881134510956, -0.002215071014480679, -0.002207653915510261, -0.002200236816539843, -0.0021928197175694253, -0.0021854026185990083, -0.00217798551962859, -0.0021705684206581722, -0.0021631513216877544, -0.002155734222717336, -0.0021483171237469192, -0.0021409000247765014, -0.0021334829258060836, -0.0021260658268356654, -0.002118648727865249, -0.0021112316288948306, -0.002103814529924413, -0.0020963974309539946, -0.002088980331983578, -0.00208156323301316, -0.002074146134042742, -0.002066729035072324, -0.0020593119361019072, -0.002051894837131489, -0.002044477738161071, -0.002037060639190653, -0.0020296435402202364, -0.002022226441249818, -0.0020148093422794004, -0.0020073922433089825, -0.0019999751443385643, -0.0019925580453681478, -0.0019851409463977295, -0.0019777238474273117, -0.0019703067484568935, -0.001962889649486477, -0.0019554725505160587, -0.001948055451545641, -0.0019406383525752229, -0.001933221253604806, -0.0019258041546343881, -0.00191838705566397, -0.001910969956693552, -0.0019035528577231353, -0.0018961357587527173, -0.0018887186597822993, -0.0018813015608118812, -0.0018738844618414645, -0.0018664673628710465, -0.0018590502639006285, -0.0018516331649302104, -0.0018442160659597937, -0.0018367989669893757, -0.0018293818680189576, -0.0018219647690485398, -0.0018145476700781218, -0.0018071305711077049, -0.001799713472137287, -0.001792296373166869, -0.001784879274196451, -0.0017774621752260343, -0.0017700450762556164, -0.0017626279772851984, -0.0017552108783147804, -0.0017477937793443637, -0.0017403766803739456, -0.0017329595814035276, -0.0017255424824331098, -0.0017181253834626928, -0.0017107082844922748, -0.001703291185521857, -0.001695874086551439, -0.001688456987581022, -0.0016810398886106042, -0.0016736227896401862, -0.0016662056906697682, -0.0016587885916993514, -0.0016513714927289334, -0.0016439543937585154, -0.0016365372947880973, -0.0016291201958176793, -0.0016217030968472626, -0.0016142859978768445, -0.0016068688989064265, -0.0015994517999360085, -0.0015920347009655918, -0.0015846176019951737, -0.001577200503024756, -0.0015697834040543379, -0.001562366305083921, -0.001554949206113503, -0.001547532107143085, -0.001540115008172667, -0.0015326979092022501, -0.001525280810231832, -0.0015178637112614143, -0.0015104466122909963, -0.0015030295133205795, -0.0014956124143501615, -0.0014881953153797435, -0.0014807782164093254, -0.0014733611174389087, -0.0014659440184684907, -0.0014585269194980727, -0.0014511098205276546, -0.0014436927215572366, -0.0014362756225868199, -0.0014288585236164018, -0.001421441424645984, -0.001414024325675566, -0.001406607226705149, -0.001399190127734731, -0.0013917730287643132, -0.0013843559297938952, -0.0013769388308234785, -0.0013695217318530604, -0.0013621046328826424, -0.0013546875339122244, -0.0013472704349418076, -0.0013398533359713896, -0.0013324362370009716, -0.0013250191380305535, -0.0013176020390601368, -0.0013101849400897188, -0.0013027678411193008, -0.001295350742148883, -0.001287933643178466, -0.001280516544208048, -0.00127309944523763, -0.0012656823462672121, -0.001258265247296794, -0.0012508481483263774, -0.0012434310493559591, -0.0012360139503855413, -0.0012285968514151233, -0.0012211797524447066, -0.0012137626534742885, -0.0012063455545038705, -0.0011989284555334525, -0.0011915113565630357, -0.0011840942575926177, -0.0011766771586221997, -0.0011692600596517819, -0.001161842960681365, -0.001154425861710947, -0.0011470087627405289, -0.001139591663770111, -0.001132174564799694, -0.0011247574658292763, -0.001117340366858858, -0.0011099232678884402, -0.0011025061689180233, -0.0010950890699476055, -0.0010876719709771872, -0.0010802548720067694, -0.0010728377730363514, -0.0010654206740659347, -0.0010580035750955166, -0.0010505864761250986, -0.0010431693771546808, -0.0010357522781842638, -0.0010283351792138458, -0.0010209180802434278, -0.00101350098127301, -0.001006083882302593, -0.000998666783332175, -0.000991249684361757, -0.0009838325853913392, -0.0009764154864209222, -0.0009689983874505043, -0.0009615812884800863, -0.0009541641895096683, -0.0009467470905392515, -0.0009393299915688335, -0.0009319128925984156, -0.0009244957936279975, -0.0009170786946575807, -0.0009096615956871628, -0.0009022444967167447, -0.0008948273977463267, -0.0008874102987759088, -0.000879993199805492, -0.0008725761008350739, -0.000865159001864656, -0.000857741902894238, -0.0008503248039238211, -0.0008429077049534032, -0.0008354906059829852, -0.0008280735070125672, -0.0008206564080421504, -0.0008132393090717324, -0.0008058222101013144, -0.0007984051111308964, -0.0007909880121604795, -0.0007835709131900617, -0.0007761538142196437, -0.0007687367152492256, -0.0007613196162788089, -0.0007539025173083909, -0.0007464854183379728, -0.0007390683193675548, -0.0007316512203971381, -0.0007242341214267201, -0.000716817022456302, -0.000709399923485884, -0.0007019828245154662, -0.0006945657255450492, -0.0006871486265746312, -0.0006797315276042134, -0.0006723144286337954, -0.0006648973296633784, -0.0006574802306929606, -0.0006500631317225426, -0.0006426460327521246, -0.0006352289337817078, -0.0006278118348112898, -0.0006203947358408718, -0.0006129776368704537, -0.000605560537900037, -0.000598143438929619, -0.000590726339959201, -0.0005833092409887829, -0.0005758921420183662, -0.0005684750430479482, -0.0005610579440775301, -0.0005536408451071123, -0.0005462237461366954, -0.0005388066471662773, -0.0005313895481958595, -0.0005239724492254415, -0.0005165553502550235, -0.0005091382512846065, -0.0005017211523141887, -0.0004943040533437707, -0.00048688695437335266, -0.00047946985540293593, -0.0004720527564325179, -0.00046463565746209987, -0.00045721855849168184, -0.0004498014595212651, -0.0004423843605508471, -0.00043496726158042905, -0.000427550162610011, -0.0004201330636395943, -0.00041271596466917627, -0.00040529886569875824, -0.0003978817667283404, -0.0003904646677579235, -0.00038304756878750545, -0.00037563046981708764, -0.0003682133708466696, -0.00036079627187625266, -0.00035337917290583485, -0.0003459620739354168, -0.0003385449749649988, -0.00033112787599458076, -0.00032371077702416404, -0.000316293678053746, -0.000308876579083328, -0.00030145948011290995, -0.0002940423811424932, -0.0002866252821720752, -0.00027920818320165716, -0.00027179108423123935, -0.0002643739852608224, -0.0002569568862904044, -0.00024953978731998656, -0.00024212268834956853, -0.00023470558937915159, -0.00022728849040873356, -0.00021987139143831574, -0.00021245429246789771, -0.00020503719349748077, -0.00019762009452706296, -0.00019020299555664493, -0.0001827858965862269, -0.00017536879761581017, -0.00016795169864539214, -0.0001605345996749741, -0.00015311750070455608, -0.00014570040173413805, -0.00013828330276372132, -0.0001308662037933033, -0.00012344910482288527, -0.00011603200585246745, -0.00010861490688205051, -0.00010119780791163248, -9.378070894121467e-05, -8.636360997079664e-05, -7.894651100037969e-05, -7.152941202996188e-05, -6.411231305954385e-05, -5.669521408912582e-05, -4.927811511870909e-05, -4.186101614829106e-05, -3.444391717787303e-05, -2.7026818207455004e-05, -1.9609719237038276e-05, -1.2192620266620246e-05, -4.775521296202217e-06, 2.6415776742158125e-06, 1.005867664463254e-05, 1.747577561505057e-05, 2.48928745854686e-05, 3.230997355588641e-05, 3.972707252630444e-05, 4.7144171496721387e-05, 5.4561270467139416e-05, 6.197836943755723e-05, 6.939546840797526e-05, 7.68125673783922e-05, 8.422966634881002e-05, 9.164676531922804e-05, 9.906386428964607e-05, 0.0001064809632600628, 0.00011389806223048083, 0.00012131516120089886, 0.0001287322601713169, 0.00013614935914173362, 0.00014356645811215165, 0.00015098355708256968, 0.0001584006560529877, 0.00016581775502340444, 0.00017323485399382246, 0.0001806519529642405, 0.0001880690519346583, 0.00019548615090507655, 0.00020290324987549306, 0.0002103203488459113, 0.00021773744781632912, 0.00022515454678674737, 0.00023257164575716388, 0.00023998874472758213, 0.00024740584369799994, 0.00025482294266841775, 0.0002622400416388347, 0.00026965714060925294, 0.00027707423957967076, 0.00028449133855008857, 0.0002919084375205055, 0.0002993255364909233, 0.00030674263546134157, 0.0003141597344317594, 0.00032157683340217633, 0.00032899393237259414, 0.0003364110313430124, 0.0003438281303134302, 0.00035124522928384715, 0.00035866232825426496, 0.0003660794272246832, 0.000373496526195101, 0.00038091362516551883, 0.0003883307241359358, 0.000395747823106354, 0.00040316492207677183, 0.00041058202104718965, 0.0004179991200176066, 0.0004254162189880244, 0.00043283331795844265, 0.00044025041692886046, 0.0004476675158992774, 0.0004550846148696952, 0.00046250171384011347, 0.0004699188128105313, 0.0004773359117809482, 0.00048475301075136604, 0.0004921701097217843, 0.0004995872086922021, 0.000507004307662619, 0.0005144214066330369, 0.0005218385056034551, 0.0005292556045738729, 0.0005366727035442899, 0.0005440898025147077, 0.0005515069014851259, 0.0005589240004555437, 0.0005663410994259615, 0.0005737581983963785, 0.0005811752973667963, 0.0005885923963372145, 0.0005960094953076324, 0.0006034265942780493, 0.0006108436932484671, 0.0006182607922188854, 0.0006256778911893032, 0.0006330949901597201, 0.0006405120891301379, 0.0006479291881005562, 0.000655346287070974, 0.0006627633860413909, 0.0006701804850118087, 0.000677597583982227, 0.0006850146829526448, 0.0006924317819230618, 0.0006998488808934796, 0.0007072659798638974, 0.0007146830788343156, 0.0007221001778047326, 0.0007295172767751504, 0.0007369343757455682, 0.0007443514747159864, 0.0007517685736864043, 0.0007591856726568212, 0.000766602771627239, 0.0007740198705976573, 0.0007814369695680751, 0.000788854068538492, 0.0007962711675089098, 0.0008036882664793281, 0.0008111053654497459, 0.0008185224644201628, 0.0008259395633905806, 0.0008333566623609989, 0.0008407737613314167, 0.0008481908603018336, 0.0008556079592722515, 0.0008630250582426693, 0.0008704421572130875, 0.0008778592561835045, 0.0008852763551539223, 0.0008926934541243401, 0.0009001105530947583, 0.0009075276520651748, 0.0009149447510355931, 0.0009223618500060109, 0.0009297789489764292, 0.000937196047946847, 0.0009446131469172639, 0.0009520302458876817, 0.0009594473448581, 0.0009668644438285178, 0.0009742815427989347, 0.0009816986417693525, 0.0009891157407397703, 0.0009965328397101886, 0.0010039499386806055, 0.0010113670376510234, 0.0010187841366214412, 0.0010262012355918594, 0.0010336183345622764, 0.0010410354335326942, 0.001048452532503112, 0.0010558696314735302, 0.0010632867304439467, 0.001070703829414365, 0.0010781209283847828, 0.001085538027355201, 0.0010929551263256176, 0.0011003722252960358, 0.0011077893242664536, 0.0011152064232368719, 0.0011226235222072897, 0.0011300406211777066, 0.0011374577201481244, 0.0011448748191185422, 0.0011522919180889605, 0.0011597090170593774, 0.0011671261160297952, 0.001174543215000213, 0.0011819603139706313, 0.0011893774129410478, 0.001196794511911466, 0.0012042116108818839, 0.0012116287098523021, 0.0012190458088227186, 0.0012264629077931369, 0.0012338800067635547, 0.001241297105733973, 0.0012487142047043895, 0.0012561313036748077, 0.0012635484026452255, 0.0012709655016156433, 0.0012783826005860603, 0.0012857996995564785, 0.0012932167985268963, 0.0013006338974973141, 0.0013080509964677324, 0.0013154680954381493, 0.0013228851944085671, 0.001330302293378985, 0.0013377193923494032, 0.0013451364913198197, 0.001352553590290238, 0.0013599706892606558, 0.0013673877882310727, 0.0013748048872014905, 0.0013822219861719088, 0.0013896390851423266, 0.0013970561841127448, 0.0014044732830831626, 0.0014118903820535805, 0.001419307481023996, 0.0014267245799944143, 0.0014341416789648322, 0.0014415587779352504, 0.0014489758769056682, 0.001456392975876086, 0.0014638100748465043, 0.001471227173816922, 0.0014786442727873403, 0.001486061371757756, 0.0014934784707281738, 0.0015008955696985916, 0.0015083126686690099, 0.0015157297676394277, 0.001523146866609846, 0.0015305639655802637, 0.0015379810645506815, 0.0015453981635210972, 0.0015528152624915154, 0.0015602323614619332, 0.0015676494604323515, 0.0015750665594027693, 0.0015824836583731871, 0.0015899007573436054, 0.0015973178563140232, 0.0016047349552844388, 0.001612152054254857, 0.0016195691532252749, 0.0016269862521956927, 0.001634403351166111, 0.0016418204501365287, 0.001649237549106947, 0.0016566546480773648, 0.0016640717470477826, 0.0016714888460181983, 0.0016789059449886165, 0.0016863230439590343, 0.0016937401429294526, 0.0017011572418998704, 0.0017085743408702882, 0.0017159914398407064, 0.0017234085388111242, 0.00173082563778154, 0.0017382427367519581, 0.001745659835722376, 0.0017530769346927938, 0.001760494033663212, 0.0017679111326336298, 0.001775328231604048, 0.0017827453305744659, 0.0017901624295448815, 0.0017975795285152993, 0.0018049966274857176, 0.0018124137264561354, 0.0018198308254265536, 0.0018272479243969715, 0.0018346650233673893, 0.0018420821223378075, 0.0018494992213082253, 0.001856916320278641, 0.0018643334192490592, 0.001871750518219477, 0.0018791676171898953, 0.001886584716160313, 0.001894001815130731, 0.0019014189141011491, 0.001908836013071567, 0.0019162531120419826, 0.0019236702110124008, 0.0019310873099828187]
  out "Final x":dbl=0.0019310873099828187
  out "initial x":dbl=-0.005478594561464469
  out "y after move":dbl=-0.00627859456146447
  out "x after move":dbl=-0.005156111996998277
  out "number of samples written per channel":u32=1000
  in  "Scan mirrors out":tag="Dev1/ao1:0"
  in  "Scan Mirrors in":tag="Dev1/ai1:2"
  in  "Vis Grating Correction":dbl[][](array[numeric])=[[450.0, 0.0, 0.0], [500.0, 0.04, 0.02], [550.0, 0.01, 0.01], [600.0, -0.08, 0.01], [650.0, -0.18, 0.0], [700.0, -0.16, -0.01], [750.0, -0.12, -0.02], [800.0, -0.1, -0.04], [850.0, -0.04, -0.05], [900.0, 0.0, -0.06], [950.0, 0.0, -0.08], [1000.0, -0.1, -0.1]]
  in  "Lockin resource":refnum<visa-resource-name>="COM14"
  in  "Preamp resource":refnum<visa-resource-name>="COM14"
  in  "Preamp Bias on?":bool
  in  "Preamp Bias (mv)":i32 min=-5000 max=5000 step=25
  in  "Auto Update":bool=TRUE
  in  "Output 1":dbl=0.2501508035632204 step=0.03
  in  "Output 2":dbl=-0.11010797694125393 step=0.05
  in  "Exit":bool
  in  "Tab Control":enum32{"Imaging", "Spectral"}(tab)
  in  "Recenter?":bool
  out "Channel2":dbl[][](graph)
  in  "Update":bool
  out "Output rate":dbl=18751.171948246767
  out "Input rate":dbl=18751.171948246767
  out "Channel 2":path=path "T:/Physics/Minot Group/Lee/SPCM/2016-08-14/PC_2um_p1p1_250"
  out "Channel 1":path=path "T:/Physics/Minot Group/Lee/SPCM/2016-08-14/PC_2um_p1p1_250"
  out "Linescan 2":dbl[](graph)=[2.8616281360451744e-09, 2.7477769195591166e-09, 2.6855296645642135e-09, 2.619734646603969e-09, 2.5323304931478706e-09, 2.357199703623348e-09, 2.196260038501338e-09, 2.019194204613491e-09, 1.9134062623296084e-09, 1.8082633856201464e-09, 1.7898795101187754e-09, 1.7627874839798104e-09, 1.7892344618647176e-09, 1.8201967787599828e-09, 1.896312480611225e-09, 1.8643825876599605e-09, 1.8672853051365925e-09, 1.8692204501281485e-09, 1.8876043278332885e-09, 1.909858496275512e-09, 1.9040530609561846e-09, 1.9108260688337913e-09, 1.924049560608745e-09, 1.9079233511632906e-09, 1.9053431576893193e-09, 1.921146842878851e-09, 1.910503544647538e-09, 1.9630749891398836e-09, 1.9385631494544865e-09, 1.898247625688817e-09, 1.9443685850845926e-09, 1.9475938271240413e-09, 1.9427559640709576e-09, 1.950496544973439e-09, 1.9566245049210017e-09, 1.946948778714852e-09, 1.9740408124619302e-09, 2.0188716803723505e-09, 2.050156532538334e-09, 2.0478988627417946e-09, 2.0953099302003363e-09, 2.165942751804073e-09, 2.230770143323461e-09, 2.2988227858719187e-09, 2.3988053558323108e-09, 2.5274926252884233e-09, 2.7568076100245433e-09, 2.9387115522026845e-09, 3.2183406165686085e-09, 3.518933986445069e-09, 3.7092238874585966e-09, 3.820172615293967e-09, 3.936604306832179e-09, 4.081095760727e-09, 4.135602595359075e-09, 4.193657220605958e-09, 4.110123068156147e-09, 4.183336397696654e-09, 4.206235723904329e-09, 4.1849490262578446e-09, 4.1530189820107816e-09, 4.00885002716471e-09, 4.069484838362026e-09, 4.012075282843867e-09, 4.026588933726788e-09, 3.920800557255436e-09, 3.9124148944676966e-09, 3.934669153789264e-09, 3.9872408147937086e-09, 3.914672572893318e-09, 3.899191349657951e-09, 3.959181093025679e-09, 3.996916581380962e-09, 3.974339793044946e-09, 4.0030445670086595e-09, 4.103995080851408e-09, 4.1194763121240714e-09, 4.1188312608086776e-09, 4.1717254722568696e-09, 4.189786911982269e-09, 4.1514063535839775e-09, 4.1620497013260256e-09, 4.2088159297604835e-09, 4.254937112399558e-09, 4.196882477822367e-09, 4.282029278254082e-09, 4.234295463531106e-09, 4.27719139135123e-09, 4.227199896992681e-09, 4.250099225844832e-09, 4.239778401401863e-09, 4.268805720867143e-09, 4.34492181368369e-09, 4.310734075161775e-09, 4.2975105167624075e-09, 4.313636807555965e-09, 4.293317681269935e-09, 4.230747680245282e-09, 4.200752786518081e-09, 4.26074257634713e-09, 4.173338100769103e-09, 4.13237733865816e-09, 4.133344915665602e-09, 4.106575286020537e-09, 3.962406348300544e-09, 3.933701577271317e-09, 3.8475872764947645e-09, 3.848554852806141e-09, 3.844362022140127e-09, 3.815657259508047e-09, 3.8982237732255174e-09, 3.889515585438152e-09, 3.9472476487356926e-09, 4.005624771511919e-09, 4.0469080458631575e-09, 4.0288466128011295e-09, 4.1104455938064494e-09, 4.0749677738801564e-09, 4.060131595597144e-09, 4.032394394229869e-09, 4.030136715135146e-09, 3.913059945445151e-09, 3.8911282127919935e-09, 3.874679414084965e-09, 3.7901777527914185e-09, 3.840814242379548e-09, 3.814044632453724e-09, 3.896288620367623e-09, 3.901449028009337e-09, 3.940474612946106e-09, 3.988530916991677e-09, 3.968856858928706e-09, 3.999174260285375e-09, 4.006269822640368e-09, 4.04303773870843e-09, 4.088513850196991e-09, 4.121733991736428e-09, 4.1439882629078e-09, 4.106897811667886e-09, 4.161404649939319e-09, 4.084321017000921e-09, 4.0230411523504384e-09, 4.05722886512944e-09, 4.0311042918884394e-09, 3.978532625067268e-09, 3.9865957636963e-09, 3.981435354954829e-09, 3.860810819616334e-09, 3.836298886365324e-09, 3.746636827241499e-09, 3.5566694346580964e-09, 3.423144017193125e-09, 3.2296289905827152e-09, 3.1283561592212396e-09, 3.1847980211208594e-09, 3.209309917555692e-09, 3.368959801364383e-09, 3.5860192299966996e-09, 3.5969850881112955e-09, 3.727285306244354e-09, 3.858875666937502e-09, 3.948215225286442e-09, 3.937571883357148e-09, 3.997561632495193e-09, 4.115283478593245e-09, 4.0082049760320424e-09, 4.0230411523504384e-09, 4.0633568516976585e-09, 4.023363677928784e-09, 4.009172552731438e-09, 3.969179384462861e-09, 3.9436998680696785e-09, 3.969824435531956e-09, 3.926928541711178e-09, 3.8850002288816776e-09, 3.755345011984573e-09, 3.6856795391418374e-09, 3.597630138597383e-09, 3.457009155448353e-09, 3.275427539422822e-09, 3.148675228722906e-09, 2.8854949665501148e-09, 2.7339083595093895e-09, 2.5355557384113996e-09, 2.4010630269699973e-09, 2.269150542648132e-09, 2.197872660177296e-09, 2.1088559501457708e-09, 1.995972459674721e-09, 2.0043580896925906e-09, 2.0150013894916052e-09, 1.9988751777452025e-09, 1.9659777070596796e-09, 1.968235376562004e-09, 1.9727507155906965e-09, 1.9866192570939622e-09, 1.9604947954445013e-09, 1.931145092892418e-09, 1.9463037303063125e-09, 1.945658681898423e-09]
  out "Linescan":dbl[](graph)=[-1.2746313372481338e-13, -6.900456871093786e-12, -2.062604204549463e-12, -5.6103628281490765e-12, -4.642792295240776e-12, -7.222980381663458e-12, -4.4998664569612673e-13, -5.287839317246314e-12, -5.932886338985189e-12, -3.675221761732199e-12, -1.0448215483701392e-11, -8.19055091297311e-12, -1.7400806929125069e-12, -7.868027402603103e-12, -5.6103628281490765e-12, -5.932886338985189e-12, -4.320268784137969e-12, -3.675221761732199e-12, -3.675221761732199e-12, -4.965315806276885e-12, -3.997745272968448e-12, -5.6103628281490765e-12, -6.577933360457528e-12, -3.0301747390594496e-12, -1.2746313372481338e-13, -7.725101576005368e-13, 1.9506037831341893e-13, -3.997745272968448e-12, -2.062604204549463e-12, 1.4851544271358544e-12, -1.4175571812087111e-12, -1.7400806929125069e-12, -4.4998664569612673e-13, -1.2746313372481338e-13, -1.7400806929125069e-12, -3.3526982504292048e-12, -1.7400806929125069e-12, 2.4527249644561058e-12, -4.4998664569612673e-13, -1.2746313372481338e-13, -1.4175571812087111e-12, -2.3851277161195948e-12, 4.710389553884026e-12, -3.675221761732199e-12, -3.3526982504292048e-12, 2.1302014519489974e-12, 3.4202955023797672e-12, 5.6779600932173074e-12, 4.710389553884026e-12, 6.968054146602611e-12, 6.000483606462789e-12, 1.1483383341933487e-11, 9.548242256603055e-12, 1.6966283096908445e-11, 1.4386094974485694e-11, 1.5998712550492164e-11, 1.3418524429693514e-11, 1.2128430370916706e-11, 9.870765770656217e-12, 1.0838336313220224e-11, 7.290577660117066e-12, 8.58067171484787e-12, 9.870765770656217e-12, 6.6455306331554235e-12, 8.25814820106419e-12, 6.000483606462789e-12, 1.1160859827543118e-11, 1.8076779395089188e-12, 3.4202955023797672e-12, 3.4202955023797672e-12, 3.742819015155153e-12, 6.323007119775488e-12, 1.4851544271358544e-12, 4.387866040907266e-12, 3.0977719896714747e-12, 4.387866040907266e-12, 5.355436580039031e-12, 5.6779600932173074e-12, 5.6779600932173074e-12, 4.065342527997647e-12, -1.2746313372481338e-13, 5.032913066927943e-12, 6.000483606462789e-12, 3.742819015155153e-12, 4.065342527997647e-12, 5.355436580039031e-12, 4.387866040907266e-12, -1.4175571812087111e-12, -1.4175571812087111e-12, -1.4175571812087111e-12, -4.4998664569612673e-13, -1.2746313372481338e-13, -2.7076512276229186e-12, -1.4175571812087111e-12, 2.1302014519489974e-12, -7.725101576005368e-13, 1.8076779395089188e-12, -7.725101576005368e-13, -3.997745272968448e-12, 1.162630914829788e-12, -3.0301747390594496e-12, 1.9506037831341893e-13, -1.0950336694380597e-12, -2.3851277161195948e-12, -1.7400806929125069e-12, -1.7400806929125069e-12, -2.3851277161195948e-12, 5.17583890418586e-13, -1.0950336694380597e-12, -2.062604204549463e-12, 2.1302014519489974e-12, 1.4851544271358544e-12, -1.7400806929125069e-12, 1.162630914829788e-12, 2.7752484770302593e-12, -1.4175571812087111e-12, 1.162630914829788e-12, 3.4202955023797672e-12, 1.162630914829788e-12, 4.065342527997647e-12, -7.725101576005368e-13, -2.3851277161195948e-12, -3.3526982504292048e-12, -7.725101576005368e-13, -2.3851277161195948e-12, 4.710389553884026e-12, 1.9506037831341893e-13, 2.7752484770302593e-12, -1.0950336694380597e-12, -1.4175571812087111e-12, -1.4175571812087111e-12, -2.062604204549463e-12, 1.162630914829788e-12, 1.9506037831341893e-13, 1.9506037831341893e-13, 3.0977719896714747e-12, 3.0977719896714747e-12, 2.4527249644561058e-12, 1.9506037831341893e-13, -1.2746313372481338e-13, -3.0301747390594496e-12, -1.2746313372481338e-13, -1.4175571812087111e-12, 2.1302014519489974e-12, -4.965315806276885e-12, 1.8076779395089188e-12, -2.062604204549463e-12, -1.2746313372481338e-13, -4.4998664569612673e-13, 2.4527249644561058e-12, -1.4175571812087111e-12, 1.162630914829788e-12, 5.17583890418586e-13, -4.320268784137969e-12, 2.4527249644561058e-12, -6.577933360457528e-12, 1.9506037831341893e-13, -3.0301747390594496e-12, -2.3851277161195948e-12, -3.3526982504292048e-12, -4.642792295240776e-12, -7.725101576005368e-13, -1.0950336694380597e-12, -1.7400806929125069e-12, -2.062604204549463e-12, -2.062604204549463e-12, -5.287839317246314e-12, -5.932886338985189e-12, -8.83559793351357e-12, -9.158121443684053e-12, -4.320268784137969e-12, -1.1415786013017008e-11, -9.158121443684053e-12, -7.222980381663458e-12, -7.868027402603103e-12, -8.513074423276593e-12, -1.0770738993539655e-11, -9.480644953788062e-12, -1.3028403560549283e-11, -9.803168463825611e-12, -1.1738309522656131e-11, -9.158121443684053e-12, -8.83559793351357e-12, -9.480644953788062e-12, -9.803168463825611e-12, -7.868027402603103e-12, -5.932886338985189e-12, -4.642792295240776e-12, 1.9506037831341893e-13, -1.0125691973796717e-11, -2.7076512276229186e-12, -2.062604204549463e-12, -1.0950336694380597e-12, -2.3851277161195948e-12, -3.3526982504292048e-12, -9.480644953788062e-12, -4.4998664569612673e-13, 1.9506037831341893e-13, 4.710389553884026e-12, -1.2746313372481338e-13]
  in  "Go to Cursor":bool caption="Scan"
  in  "Scanner delay (ms)":dbl=0.16
  in  "X Scan size(um)":dbl=2.0
  in  "Scan Rate (Hz)":dbl=15.0
  in  "Y offset (um)":dbl
  in  "Scan Angle (°)":dbl
  in  "Scan Points":u32=200
  in  "Scan Lines":u32=200
  in  "Conv. (mV/um)":dbl=41.0
  in  "Reset":bool
  in  "Y Scan size(um)":dbl=2.0
  in  "Lines read":u32=1
  in  "Save Image":bool
  in  "X offset (um)":dbl
  in  "stepsize":dbl=0.001
  in  "Increment":bool
  in  "Concat":bool=TRUE
  in  "StopPoint":dbl
  in  "Start Scan":bool=TRUE caption="Scan"
  in  "Starting Point":tag="Dev1/ai2:1"
  in  "Scan Channels":cluster{dbl, string, "Output Channels":tag}[](array[cluster])=[{1.0, "", "Output Channels"="Dev1/ao1"}, {1.0, "", "Output Channels"="Dev1/ao0"}, {1.0, "", "Output Channels"="Dev2/ao2"}, {1.0, "", "Output Channels"="Dev2/ao3"}, {0.0, "", "Output Channels"=""}, {1.0, "", "Output Channels"=""}]
  in  "Inputs":cluster{dbl, string, "Input Channels":tag}[](array[cluster])=[{1.0, "", "Input Channels"="Dev1/ai16"}, {1.0, "", "Input Channels"="Dev1/ai17"}, {1.0, "", "Input Channels"=""}, {1.0, "", "Input Channels"=""}, {0.0, "", "Input Channels"=""}, {1.0, "", "Input Channels"=""}]
  in  "Input Minimum Value":dbl=-10.0 format="%0.2f"
  in  "Input Maximum Value":dbl=10.0 format="%0.2f"
  in  "Output Maximum Value":dbl=4.0 format="%0.2f"
  in  "Output Minimum Value":dbl=-4.0 format="%0.2f"
  in  "output scale":i32=1
  in  "out/in":dbl=1.0
  in  "Switch to Spectral":bool
  out "Reflection Image":dbl[][](graph)
  in  "Channel 2 Filename":string="PC_2um_p1p1"
  in  "Channel 1 filename":string="PC_2um_p1p1"
  in  "Save Channel 1?":bool=TRUE
  in  "Save Channel 2?":bool=TRUE
  in  "Averaging amount Ch1 (4 min)":i32=8
  in  "Average Ch1?":bool
  in  "Increment type":enum16{"Wavelength", "Output1"}(ring)=enum."Output1"
  in  "eV":bool=TRUE
  out "Power meter initalized?":bool
  in  "Switch to Imaging":bool
  in  "Input Channel":tag="Dev1/ai16"
  out "Readout":dbl=-6.932709220073548e-12 format="%^#_9e"
  in  "On":bool=TRUE
  in  "Current":bool=TRUE
  in  "Power":bool
  out "ScanGraph":cluster{dbl[], dbl[]}(graph)
  out "Waveform Chart":dbl(graph)=-6.932709220073548e-12
  out "Zero Value":dbl format="%#.3p"
  in  "Zero?":bool
  in  "Power Meter":refnum<visa-resource-name>="USB0::0x1313::0x8072::P2000362::INSTR"
  in  "Range":i16=1 min=1 max=6 step=1
  out "Rng":string
  out "AUTO?":bool
  in  "Double Mono":refnum<visa-resource-name>="COM16"
  out "Sensor Name":string="S122C"
  out "Sensor SN":string="10101425"
  out "IDN String":string="Thorlabs,PM100USB,P2000362,1.3.0\n"
  out "PM Error log":string
  in  "Step Size (nm)":dbl=10.0 min=0.1 max=100.0 step=0.1 format="%.1f"
  in  "Step Time (sec)":dbl=0.5 min=0.001 max=300.0 step=0.001 format="%.3f"
  in  "Start":dbl=1000.0 min=0.0 max=2000.0 step=0.1 format="%.1f"
  in  "End":dbl=1800.0 min=0.0 max=2000.0 step=0.1 format="%.1f"
  in  "Save":bool
  in  "Scan":bool
  in  "STOP":bool
  in  "Ask?":u16(ring) items=["?nm", "?nm/min", "?grating", "?turret", "?gratings"]
  in  "Send ?":bool
  in  "CMD":u16(ring)=1 items=["nm", "goto", "nm/min", "VIS grating", "IR grating"]
  in  "Send CMD":bool
  in  "PM Settings":T5={"Spot Size (mm)"=4.0, "BWIn"=0, "Averaging Rate"=300, "Auto Range"=TRUE} {"Spot Size (mm)" min=1.0 max=9.0 step=0.5; "BWIn" items=["HIGH", "LOW"]; "Averaging Rate" min=33 max=5000 step=1}
  out "path":path=path "T:/Physics/Minot Group/Lee/SPCM/2016-08-14/testx"
  in  "Filename":string="testx"
  in  "Reset Params":bool
  in  "Record":bool
  in  "Normalize?":bool=TRUE
  in  "Calculate current offset":bool
  in  "Current offset":dbl
  in  "Use Current offset":bool=TRUE
  out "Data stream":string="Wavelength (nm)"
  out "Measuring?":bool
  out "Saved?":bool
  # "Square wave peak to peak value = lockin output x 2.222...\nNot included in multiplication factor"
  # "Conversion"
  # "Output channel 1"
  # "Output channel 2"
  # "y is inverted"
  # "Scan channel 1"
  # "Scan channel 2"
  # "Input channel 1"
  # "Input channel 2"
  # "nm"
  # "Range Settings"
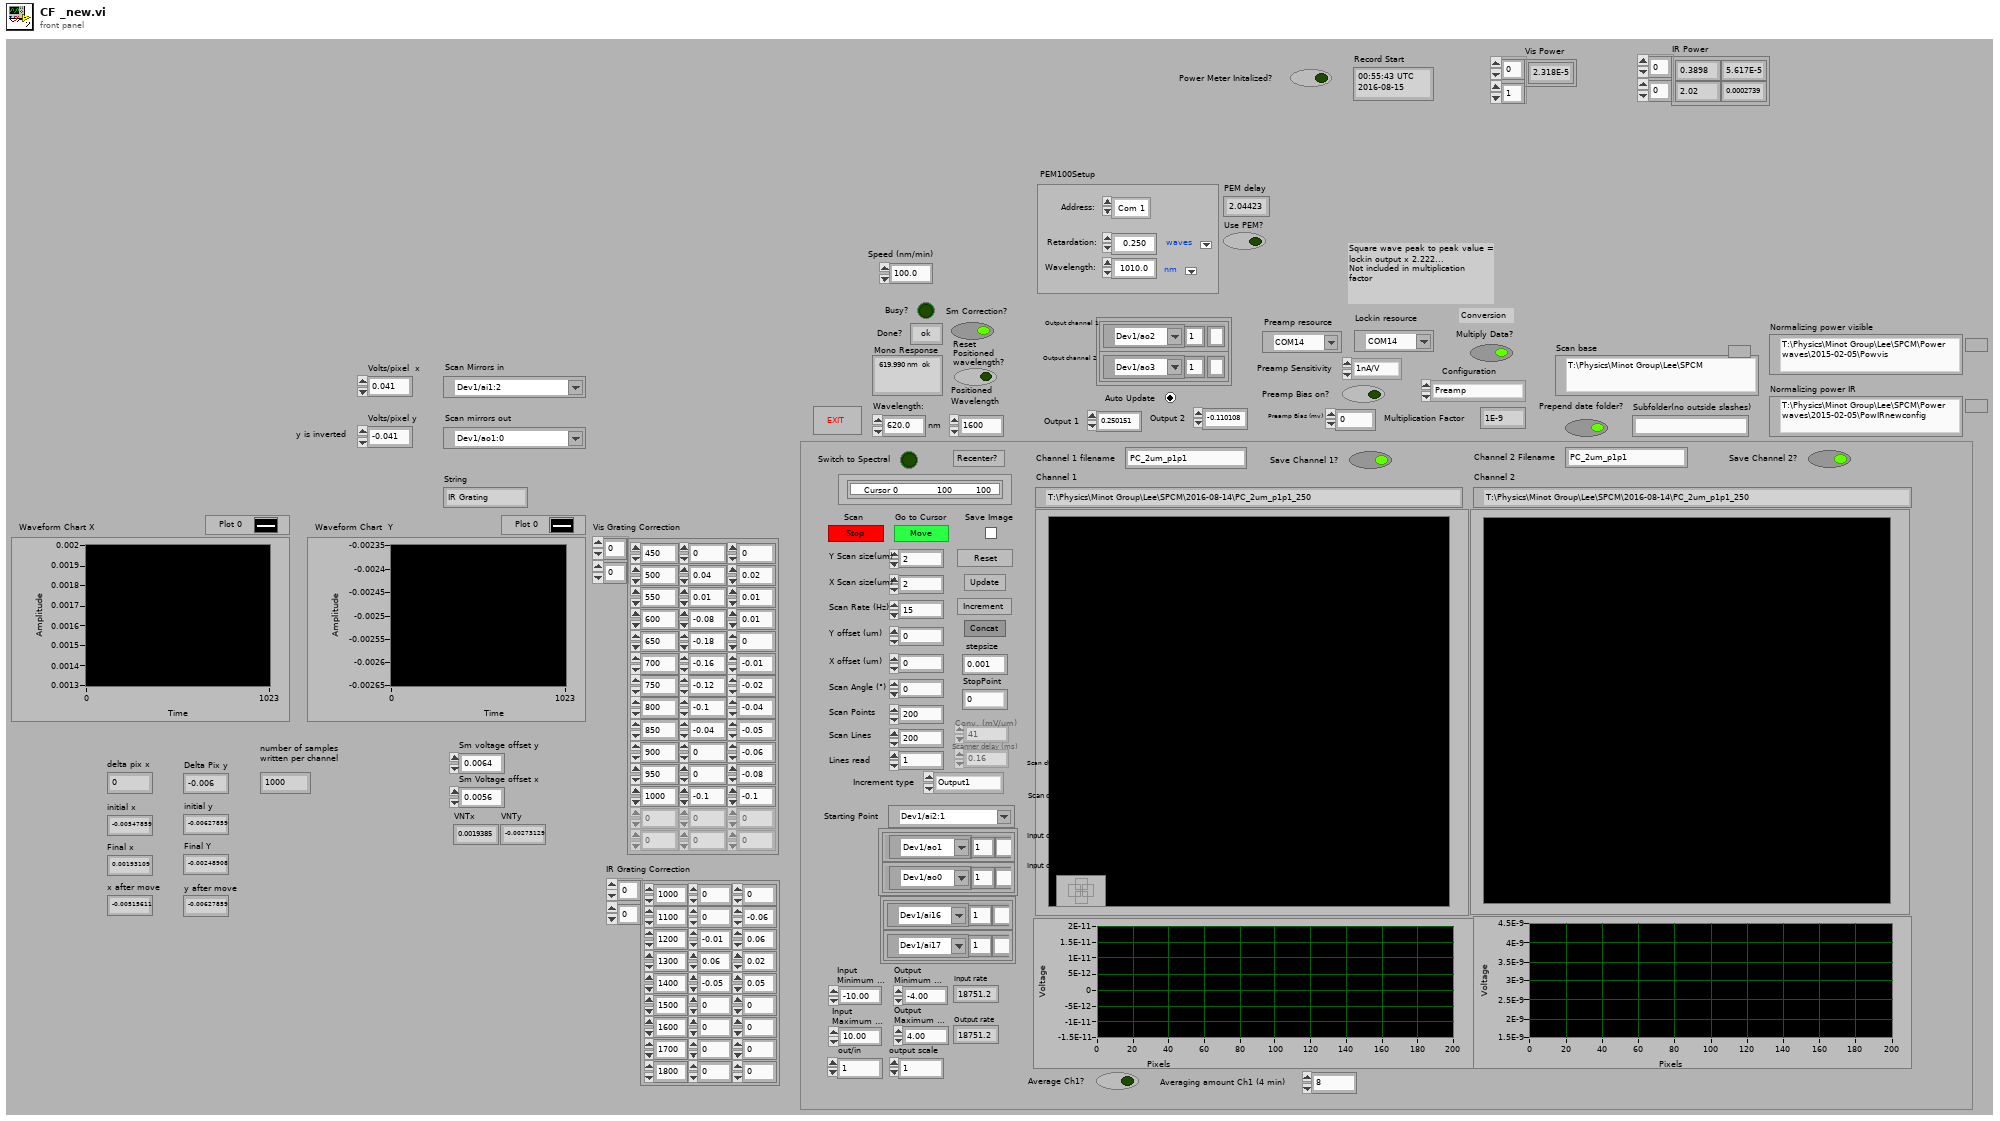
[diagram p1: front panel]
types:
  T1 = typedef "HindsPEM100_Setup.ctl" = cluster{"Address:":T2, "Retardation:":dbl, "RTD Units":u16, "Wavelength:":dbl, "Wave Units":u16}
  T2 = typedef "Com Address.ctl" = u16
  T3 = enum16{"1pA/V", "2pA/V", "5pA/V", "10pA/V", "20pA/V", "50pA/V", "100pA/V", "200pA/V", "500pA/V", "1nA/V", "2nA/V", "5nA/V", "10nA/V", "20nA/V", "50nA/V", "100nA/V", "200nA/V", "500nA/V", "1uA/V", "2uA/V", "5uA/V", "10uA/V", "20uA/V", "50uA/V", "100uA/V", "200uA/V", "500uA/V", "1mA/V"}
  T4 = enum16{"Preamp to Lockin", "Preamp", "Lockin current", "Lockin Voltage", ""}
  T5 = cluster{"Spot Size (mm)":dbl, "BWIn":u16, "Averaging Rate":i32, "Auto Range":bool}
  T6 = enum16{"Sine Wave", "Triangle Wave", "Square Wave", "Sawtooth Wave"}
  T7 = cluster{"Scanner delay (ms)":dbl, "Y Scan size(um) ":dbl, "X Scan size(um)":dbl, "Scan Rate (Hz)":dbl, "Y offset (um)":dbl, "X offset (um)":dbl, "Scan Angle (°)":dbl, "Conv. (mV/um)":dbl, "Lines read":u32, "Scan Lines":u32, "Scan Points":u32}
  T8 = typedef "LVPointDoubleTypeDef.ctl" = cluster{"Cursor X":dbl, "Cursor Y":dbl}
  T9 = enum16{"open", "open or create", "create or replace", "create", "open (read only)"}
  T10 = cluster{"Address:":T2, "Retardation:":dbl, "RTD Units":u16, "Wavelength:":dbl, "Wave Units":u16}
  T11 = cluster{"X offset (um)":dbl, "Y offset (um)":dbl}
  T12 = cluster{"Address:":T2, "Retardation:":dbl, "RTD Units":u16, dbl, "Wave Units":u16}
  T13 = cluster{"Multiply Data?":bool, "Configuration":enum16{"Preamp to Lockin", "Preamp", "Lockin current", "Lockin Voltage", ""}, "Preamp Sensitivity":enum16{"1pA/V", "2pA/V", "5pA/V", "10pA/V", "20pA/V", "50pA/V", "100pA/V", "200pA/V", "500pA/V", "1nA/V", "2nA/V", "5nA/V", "10nA/V", "20nA/V", "50nA/V", "100nA/V", "200nA/V", "500nA/V", "1uA/V", "2uA/V", "5uA/V", "10uA/V", "20uA/V", "50uA/V", "100uA/V", "200uA/V", "500uA/V", "1mA/V"}, "Step Time (sec)":dbl, "Output 1":dbl, "Output 2":dbl, "Preamp Bias (mv)":i32, "Preamp Bias on?":bool, "Wavelength:":dbl, "Use Current offset":bool, "Current offset":dbl, "YScale.NameLbl.Text":string, "XScale.NameLbl.Text":string, "Normalizing power visible":path, "Normalizing power IR":path}
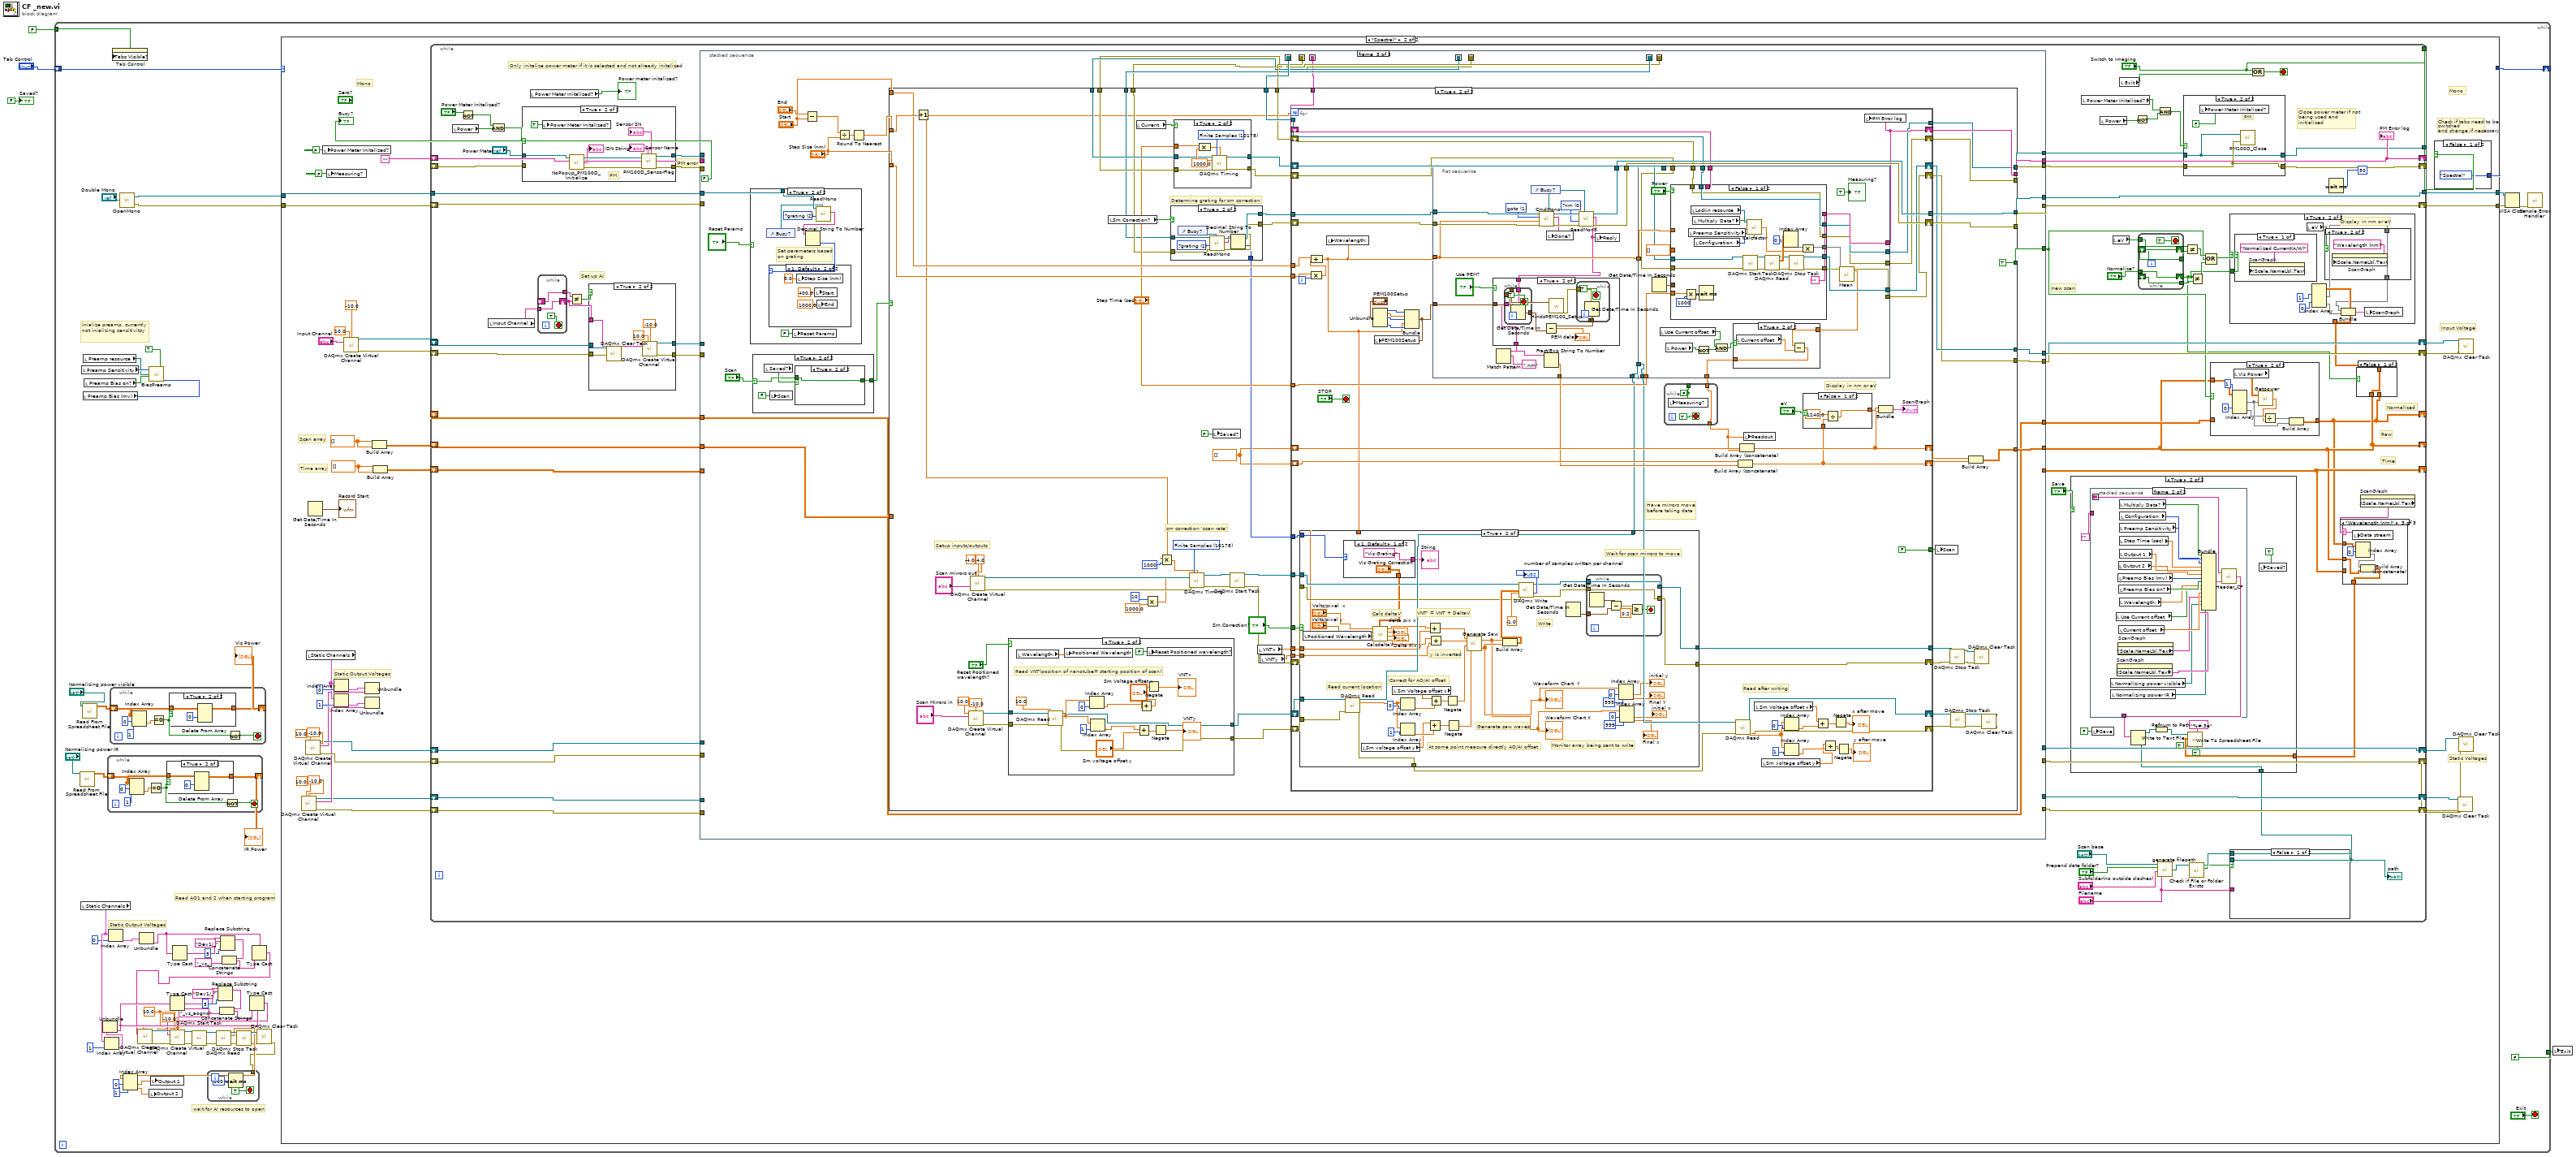
[diagram p0: block diagram]
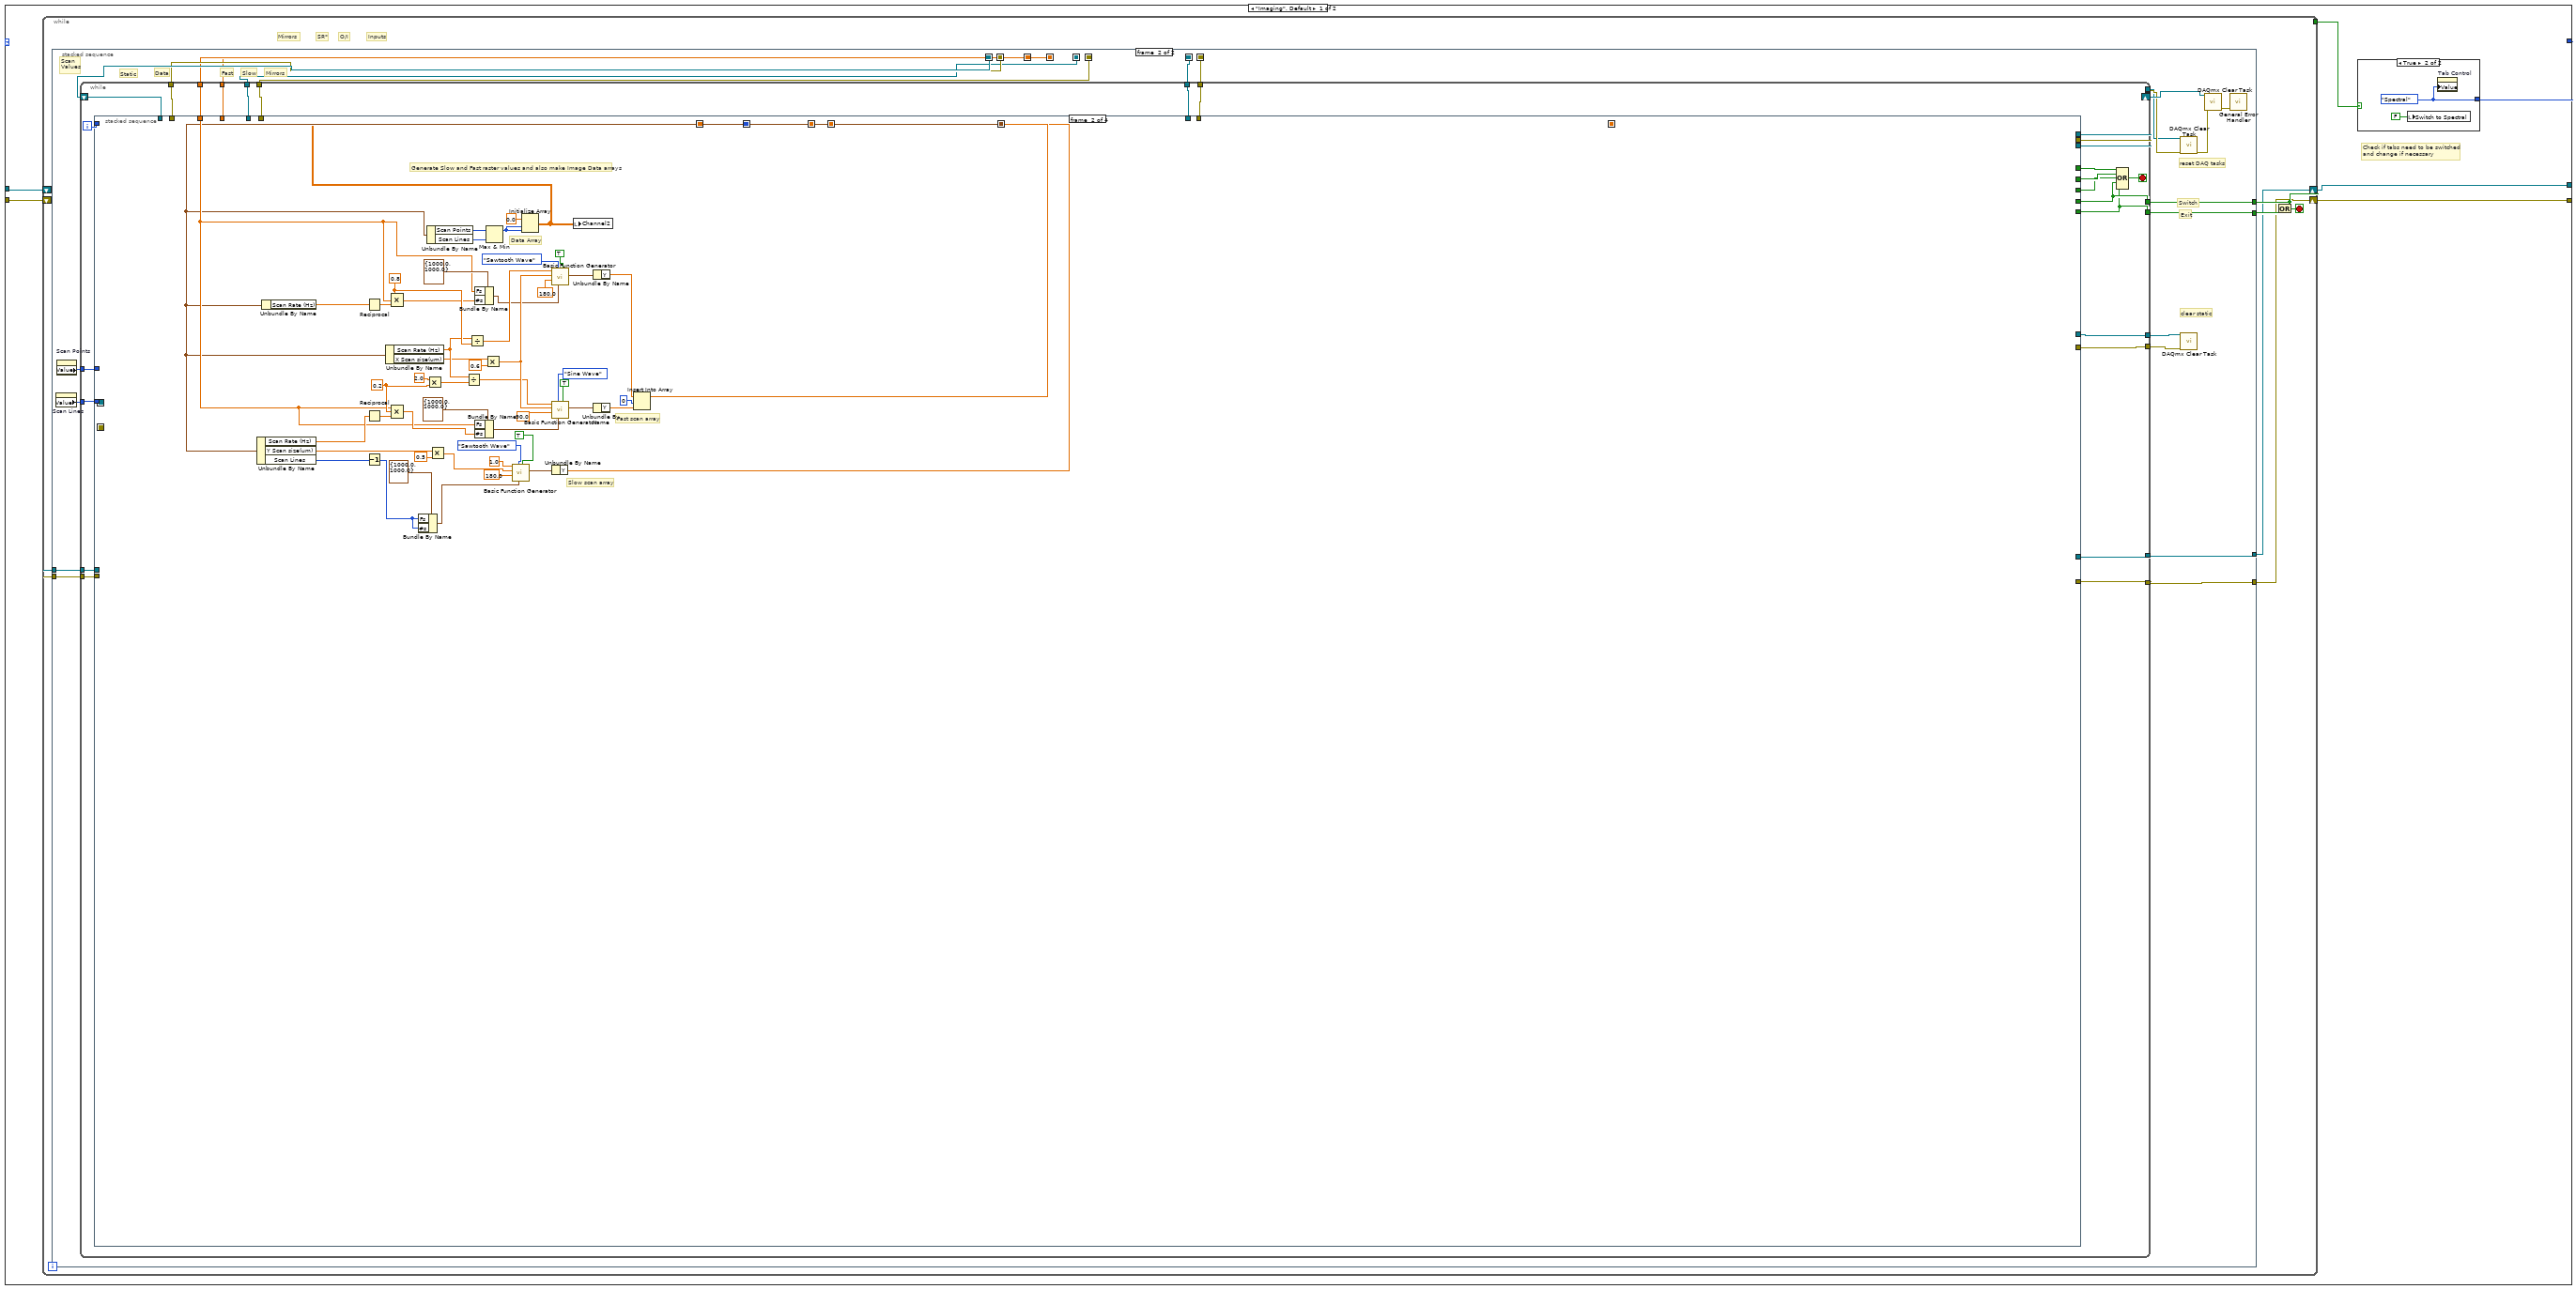
[diagram p4: hidden frame]
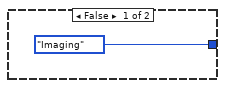
[diagram p5: hidden frame]
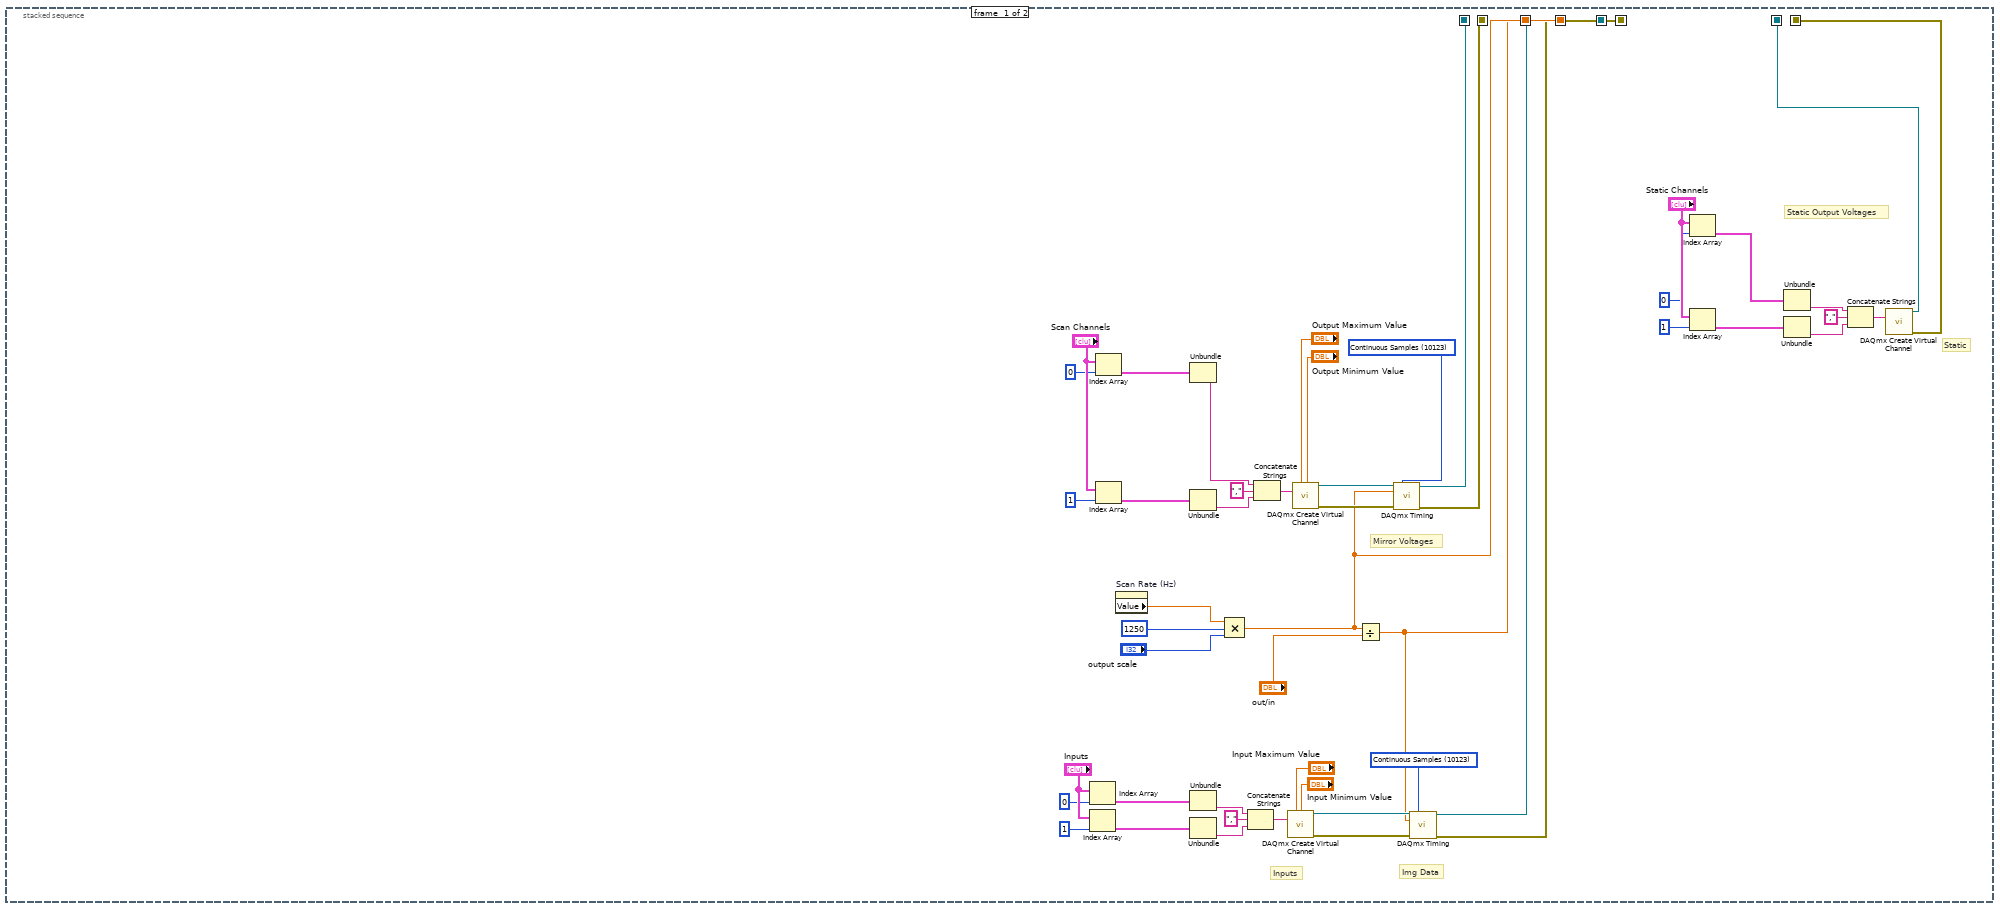
[diagram p6: hidden frame]
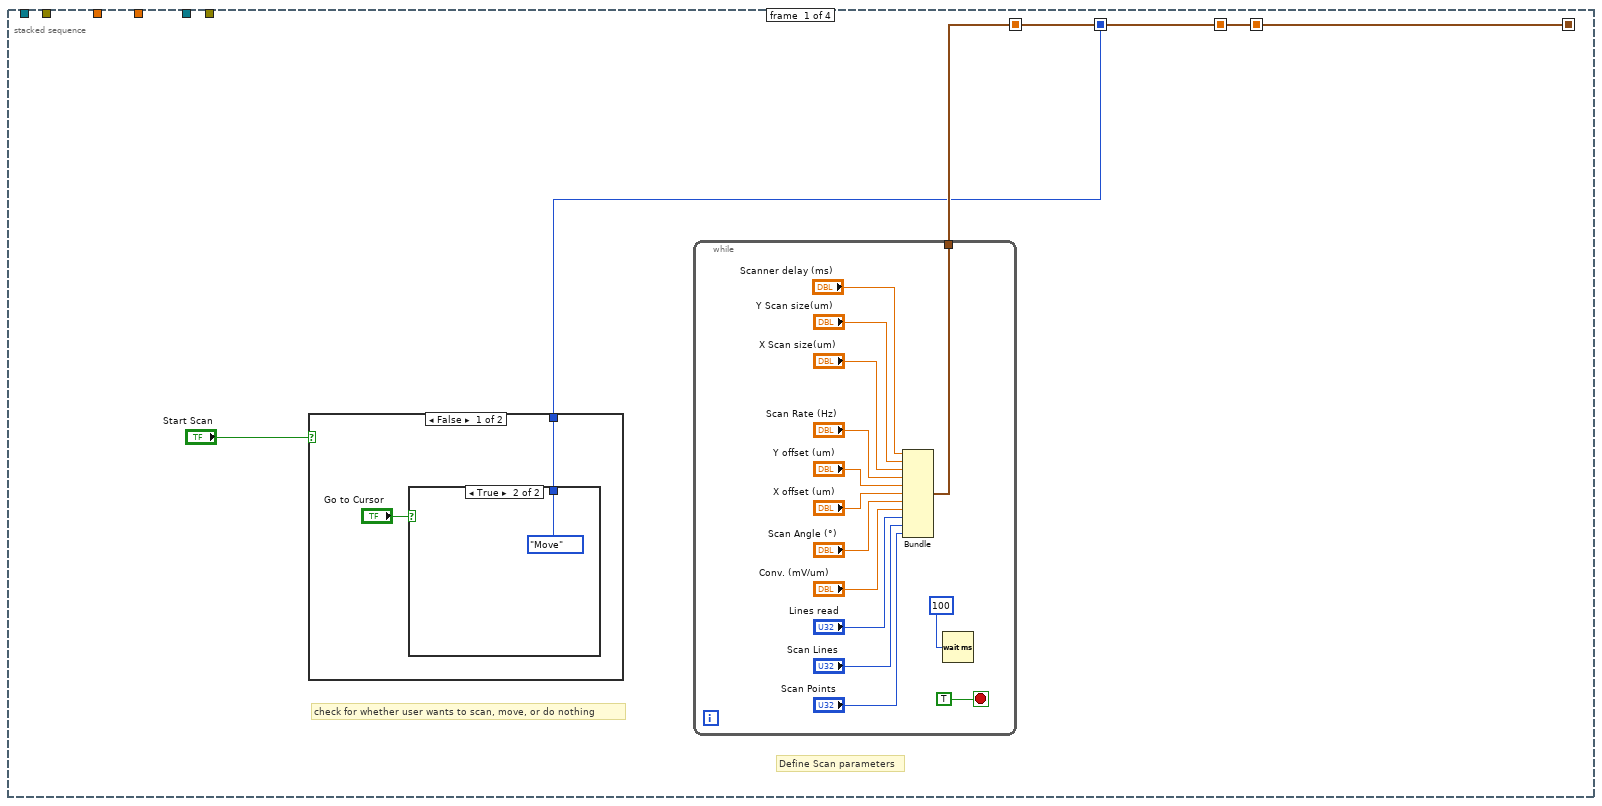
[diagram p7: hidden frame]
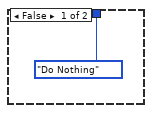
[diagram p8: hidden frame]
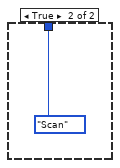
[diagram p9: hidden frame]
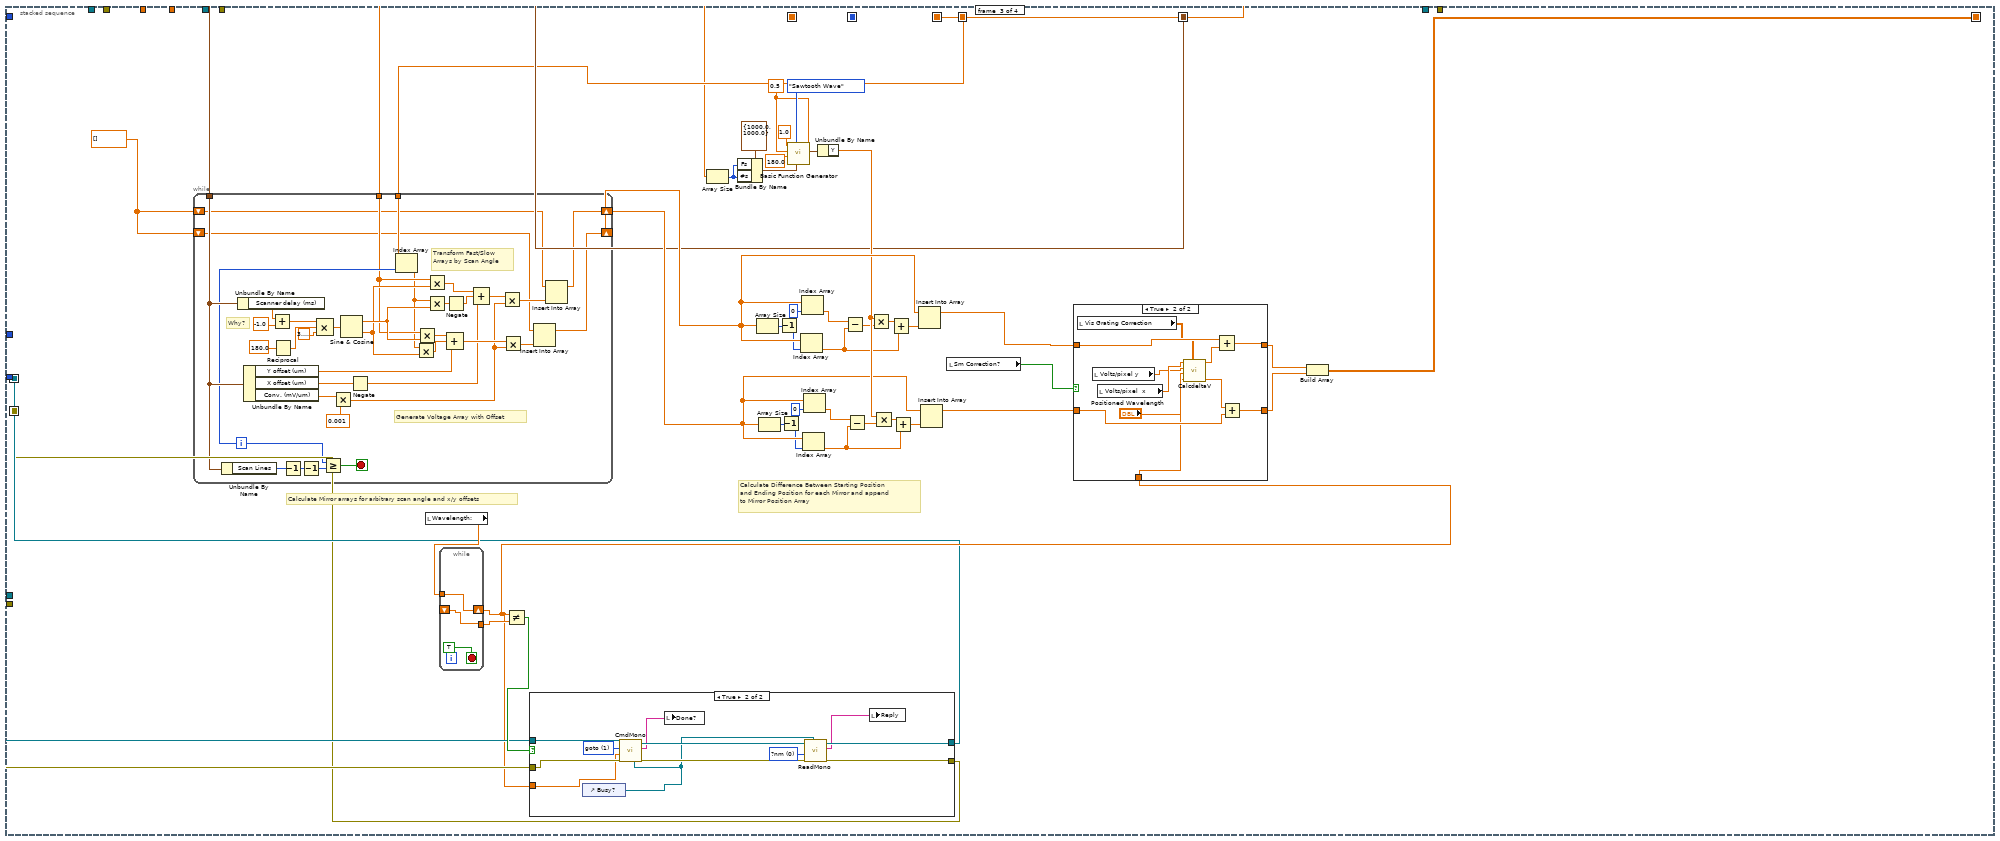
[diagram p10: hidden frame]
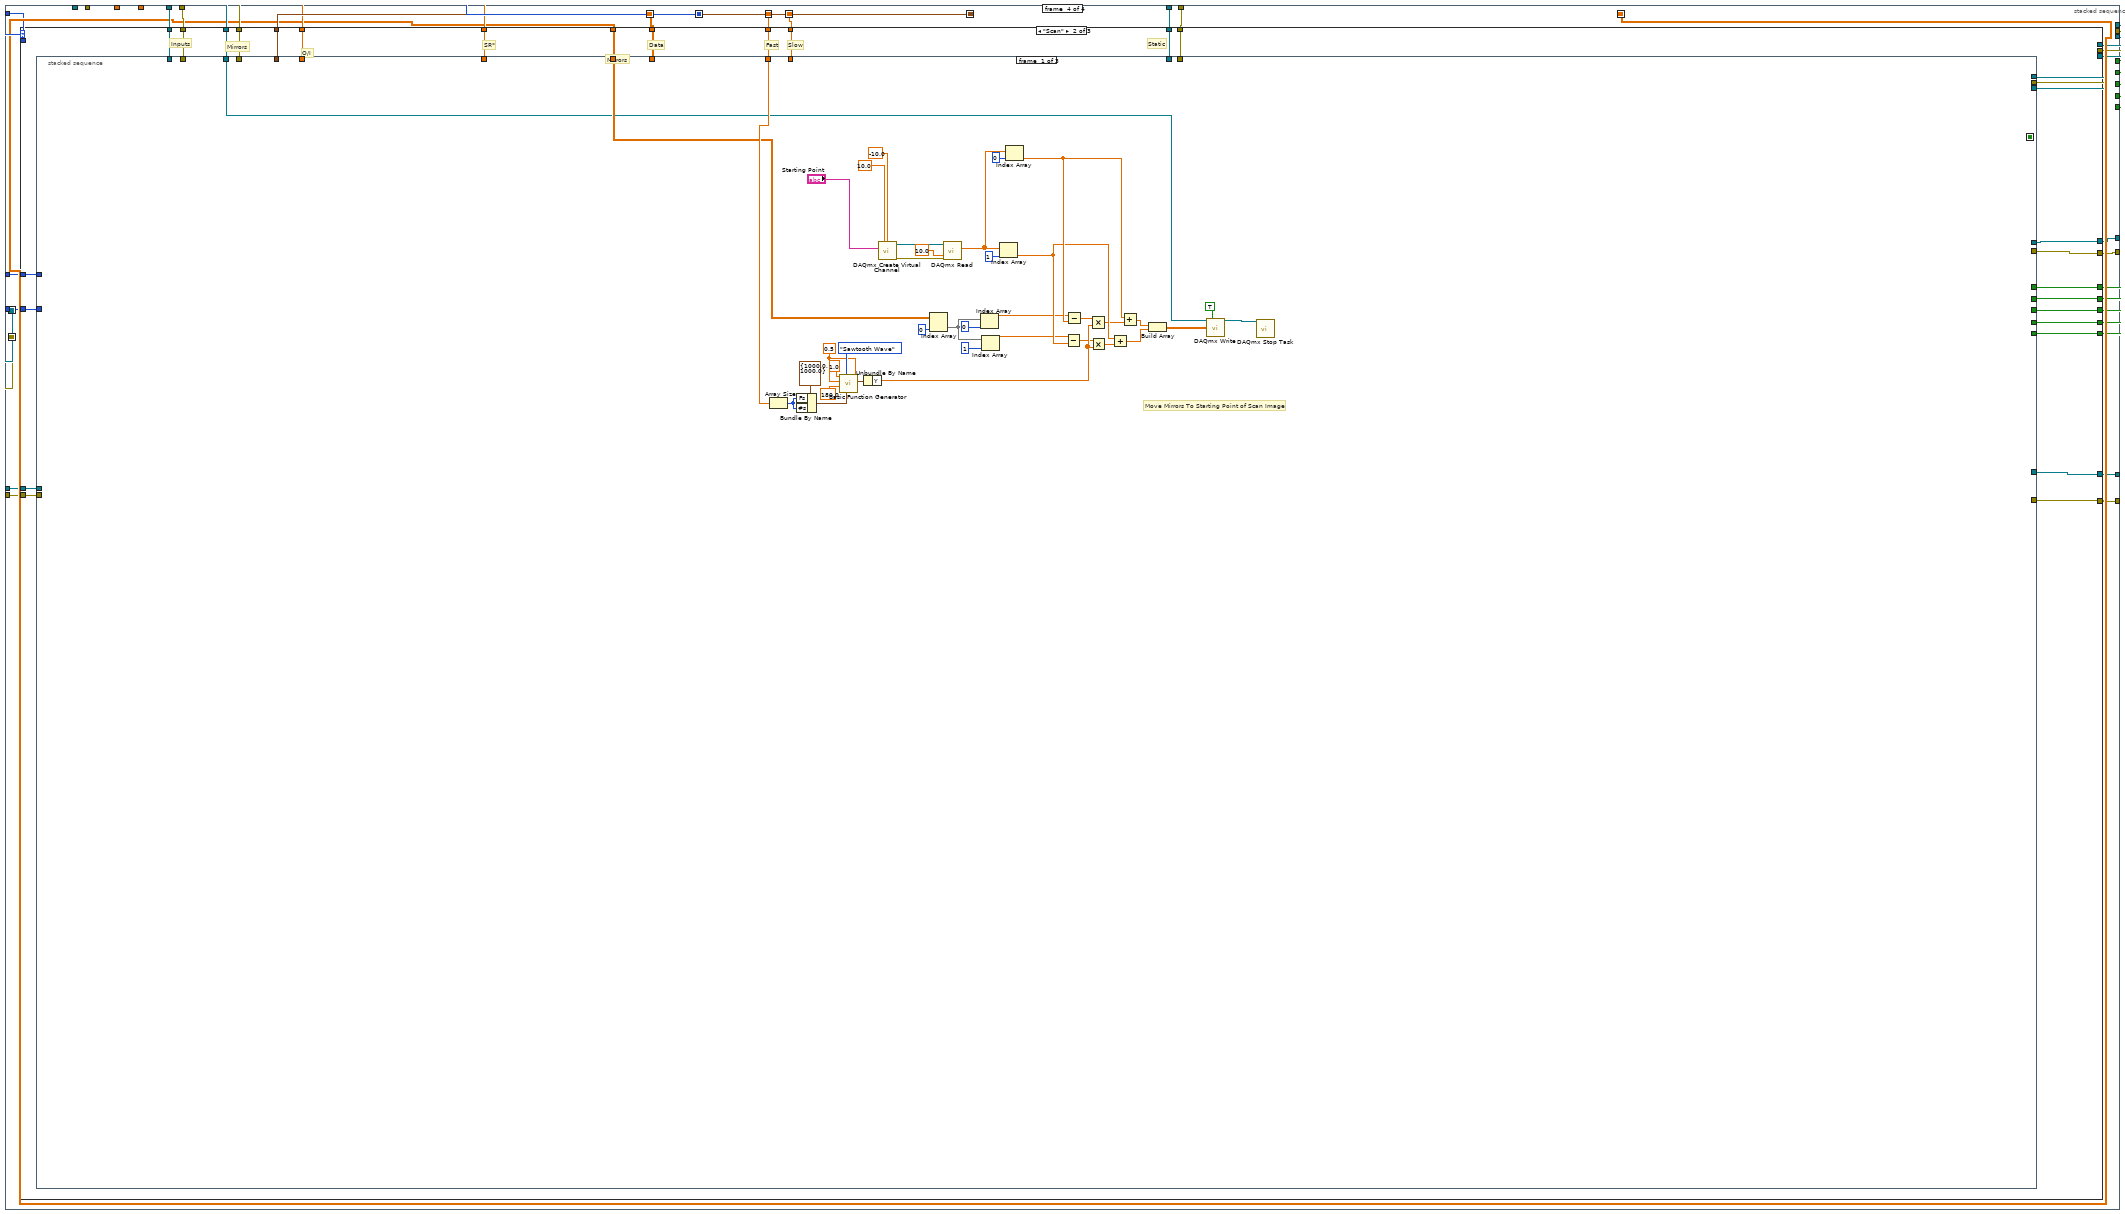
[diagram p13: hidden frame]
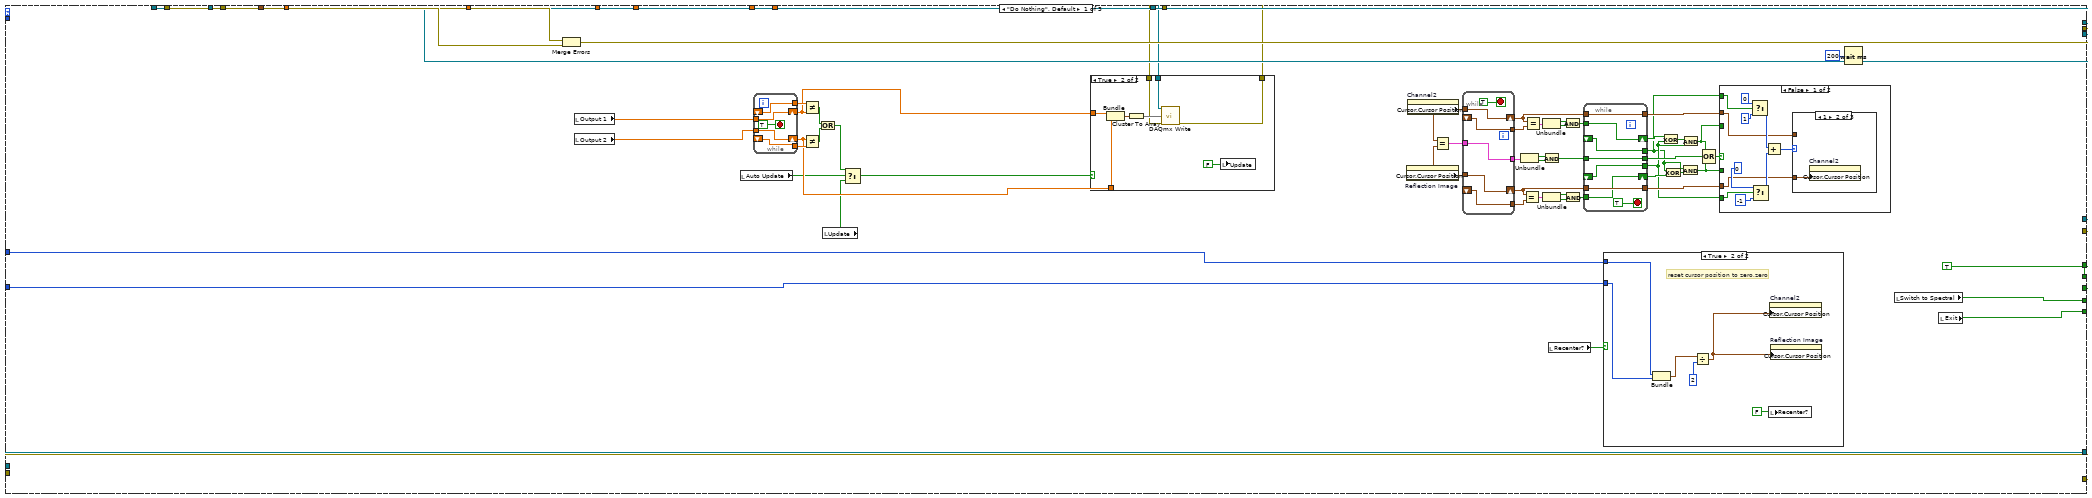
[diagram p14: hidden frame]
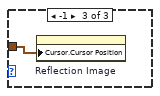
[diagram p18: hidden frame]
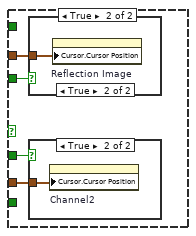
[diagram p19: hidden frame]
diagram:
  n1 = while {
    tunnel: [FALSE ("Exit")] -> w4
    shift-right: [w62] -> _
    shift-left: "Tab Control" -> [w63]
    tunnel: FALSE ("Tabs Visible?") -> [w61]
    stop <- "Exit" stop-if-true
    w5 = -10.0 ("minimum value")
    w6 = 10.0 ("maximum value")
    # "Read AO1 and 2 when starting program"
    # "wait for AI resources to open"
    # "Static Output Voltages"
    # "Inialize preamp, currently not inializing sensitivitsy"
    n2 = call-poly <vilib>:"Read From Spreadsheet File.vi"("file path (dialog if empty)"="Normalizing power IR") -> ("all rows"=w48:dbl[][])  [unwired: 6 in, 4 out]
    n3 = local read "Static Channels"() -> (w43:cluster{dbl, string, "Output Channels":tag}[])
    n4 = local read "Preamp Sensitivity"() -> (w58:T3)
    n5 = call-poly <vilib>:"Read From Spreadsheet File.vi"("file path (dialog if empty)"="Normalizing power visible") -> ("all rows"=w49:dbl[][])  [unwired: 6 in, 4 out]
    n6 = local read "Preamp Bias (mv)"() -> (w60:i32)
    n7 = local read "Preamp resource"() -> (w57:refnum<visa-resource-name>)
    n8 = local read "Preamp Bias on?"() -> (w59:bool)
    n9 = Index Array(array=w43, index=1) -> (element=w41:cluster{dbl, string, "Output Channels":tag})
    n10 = Unbundle(w41) -> ("Output Channels"=w29:tag)  [unwired: 2 out]
    n11 = while {
      shift-right: [w71] -> w44
      shift-left: w48 -> [w73]
      stop <- w69 stop-if-true
      n12 = Index Array(array=w73, index (row)=0 ("disabled index (row)"), index (col)=1 ("disabled index (col)")) -> (element=w74:dbl)
      n13 = Equal To 0?(x=w74) -> (x = 0?=w70:bool)
      n14 = case shown="True" w70 {
        tunnel: w73 -> [w75 w78]
        tunnel: [w75 w77] -> w71
        frame False {
        }
        frame True {
          n15 = Delete From Array(array=w78, index (row)=0) -> (array with subset deleted=w77:dbl[][])  [unwired: 2 in, 1 out]
        }
      }
      n16 = Not(x=w70) -> (.not. x?=w69:bool)
    }
    "IR Power" <- w44
    n17 = Index Array(array=w43, index=0) -> (element=w42:cluster{dbl, string, "Output Channels":tag})
    n18 = while {
      shift-right: [w82] -> w45
      shift-left: w49 -> [w84]
      stop <- w80 stop-if-true
      n19 = Index Array(array=w84, index (row)=0 ("disabled index (row)"), index (col)=1 ("disabled index (col)")) -> (element=w85:dbl)
      n20 = Equal To 0?(x=w85) -> (x = 0?=w81:bool)
      n21 = case shown="True" w81 {
        tunnel: w84 -> [w86 w89]
        tunnel: [w86 w88] -> w82
        frame False {
        }
        frame True {
          n22 = Delete From Array(array=w89, index (row)=0) -> (array with subset deleted=w88:dbl[][])  [unwired: 2 in, 1 out]
        }
      }
      n23 = Not(x=w81) -> (.not. x?=w80:bool)
    }
    "Vis Power" <- w45
    n24 = property on="Tab Control" class="TabCtl (strict)"("Tabs Visible?"=w61) -> ()  [unwired: 2 in, 2 out]
    n25 = call "OpenMono.vi"("Mono Port"="Double Mono") -> ("VISA resource name out"=w54:refnum<visa-resource-name>, "error out"=w53:errorcluster)
    n26 = Unbundle(w42) -> ("Output Channels"=w22:tag)  [unwired: 2 out]
    n27 = call "BiasPreamp.vi"("VISA resource name"=w57, "CHANGE SENS?"=TRUE, "Sensitivity"=w58, "Bias on"=w59, "Bias Voltage (mv)"=w60) -> ()
    n28 = Type Cast(x=w29) -> (*(type *) &x=w33:string)  [unwired: 1 in]
    n29 = Type Cast(x=w22) -> (*(type *) &x=w28:string)  [unwired: 1 in]
    n30 = Replace Substring(2:5 ("length (len. of substring)"), 4:"Dev1/_" ("substring (\"\")"), 5:w33) -> (1:w36:string)  [unwired: 1 in, 1 out]
    n31 = Concatenate Strings(w36, "_vs_aognd" ("string")) -> (w38:string)
    n32 = Replace Substring(2:5 ("length (len. of substring)"), 4:"Dev1/_" ("substring (\"\")"), 5:w28) -> (1:w25:string)  [unwired: 1 in, 1 out]
    n33 = Concatenate Strings(w25, "_vs_aognd" ("string")) -> (w23:string)
    n34 = Type Cast(type=w29, x=w38) -> (*(type *) &x=w19:tag)
    n35 = Type Cast(type=w22, x=w23) -> (*(type *) &x=w21:tag)
    n36 = call-poly <vilib>:"DAQmx Create Virtual Channel.vi"("maximum value"=w6, "minimum value"=w5, "physical channels"=w21) -> ("task out"=w20:refnum<k21>, "error out"=w7:errorcluster)  [unwired: 11 in]
    n37 = call-poly <vilib>:"DAQmx Create Virtual Channel.vi"("task in"=w20, "maximum value"=w6, "minimum value"=w5, "physical channels"=w19, "error in"=w7) -> ("task out"=w18:refnum<k21>, "error out"=w8:errorcluster)  [unwired: 9 in]
    n38 = call <vilib>:"DAQmx Start Task.vi"("task/channels in"=w18, "error in"=w8) -> ("task out"=w30:refnum<k21>, "error out"=w9:errorcluster)  [unwired: 12 in]
    n39 = call-poly <vilib>:"DAQmx Read.vi"("task/channels in"=w30, "error in"=w9) -> ("task out"=w31:refnum<k21>, "data"=w15:dbl[], "error out"=w10:errorcluster)  [unwired: 11 in]
    n40 = Index Array(array=w15, index #1=0 ("index"), index #2=1 ("index")) -> (element #1=w14:dbl, element #2=w13:dbl)
    n41 = local write "Output 2"(w13) -> ()
    n42 = local write "Output 1"(w14) -> ()
    n43 = call <vilib>:"DAQmx Stop Task.vi"("task/channels in"=w31, "error in"=w10) -> ("task out"=w32:refnum<k21>, "error out"=w11:errorcluster)  [unwired: 12 in]
    n44 = call <vilib>:"DAQmx Clear Task.vi"("task in"=w32, "error in"=w11) -> ("error out"=w12:errorcluster)  [unwired: 13 in]
    n45 = while {
      tunnel: w12 -> [_]
      stop <- TRUE stop-if-true
      n46 = Wait (ms)(milliseconds to wait=u32 100) -> ()  [unwired: 1 out]
    }
    n47 = case shown="\"Spectral\"" w63 {
      tunnel: [w95 w1403] -> w62
      tunnel: w54 -> [w93 w1394]
      tunnel: w53 -> [w92 w1395]
      tunnel: [w91 w1393] -> w50
      tunnel: [w90 w1392] -> w51
      frame "Imaging", Default {
        # "Check if tabs need to be switched\nand change if necessary"
        n48 = while {
          tunnel: [w103] -> w94
          shift-right: [w102] -> w91
          shift-left: w93 -> [w100]
          shift-right: [w101] -> w90
          shift-left: w92 -> [w99]
          stop <- w105 stop-if-true
          # "Inputs"
          # "O/I"
          # "SR*"
          # "Mirrors"
          n49 = stacked-sequence {
            seq-local: [w114 _] -> [_ w176]
            seq-local: [w115 _] -> [_ w175]
            seq-local: [w111 _] -> [_ w177]
            seq-local: [w110 _] -> [_ w174]
            seq-local: [w109 _] -> [_ w173]
            seq-local: [w108 _] -> [_ w172]
            seq-local: [w106 _] -> [_ w171]
            seq-local: [w107 _] -> [_ w170]
            tunnel: [_ w160] -> w103
            tunnel: [_ w159] -> w104
            tunnel: w99 -> [_ w157]
            tunnel: w100 -> [_ w158]
            tunnel: [_ w156] -> w102
            tunnel: [_ w155] -> w101
            frame #0 {
              w112 = 10123 items=["Finite Samples"=10178, "Continuous Samples"=10123, "Hardware Timed Single Point"=12522] ("sample mode")
              w113 = 10123 items=["Finite Samples"=10178, "Continuous Samples"=10123, "Hardware Timed Single Point"=12522] ("sample mode")
              # "Mirror Voltages"
              # "Img Data"
              # "Static Output Voltages"
              # "Inputs"
              # "Static"
              n50 = Index Array(array="Inputs", index=0) -> (element=w126:cluster{dbl, string, "Input Channels":tag})
              n51 = Index Array(array="Inputs", index=1) -> (element=w127:cluster{dbl, string, "Input Channels":tag})
              n52 = Index Array(array="Scan Channels", index=0) -> (element=w136:cluster{dbl, string, "Output Channels":tag})
              n53 = Index Array(array="Scan Channels", index=1) -> (element=w137:cluster{dbl, string, "Output Channels":tag})
              n54 = property on="Scan Rate (Hz)" class="DigNum (strict)"() -> ("Value"=w121:dbl)  [unwired: 2 in, 2 out]
              n55 = Unbundle(w136) -> ("Output Channels"=w142:tag)  [unwired: 2 out]
              n56 = Unbundle(w137) -> ("Output Channels"=w141:tag)  [unwired: 2 out]
              n57 = Unbundle(w126) -> ("Input Channels"=w130:tag)  [unwired: 2 out]
              n58 = Unbundle(w127) -> ("Input Channels"=w129:tag)  [unwired: 2 out]
              n59 = Compound Arithmetic op=MULTIPLY(w121, 1250, "output scale") -> (w109:dbl)
              n60 = Concatenate Strings(w130, ",", w129) -> (w131:string)
              n61 = Concatenate Strings(w142, ",", w141) -> (w143:string)
              n62 = call-poly <vilib>:"DAQmx Create Virtual Channel.vi"("maximum value"="Input Maximum Value", "minimum value"="Input Minimum Value", "physical channels"=w131) -> ("task out"=w117:refnum<k21>, "error out"=w116:errorcluster)  [unwired: 11 in]
              n63 = call-poly <vilib>:"DAQmx Create Virtual Channel.vi"("maximum value"="Output Maximum Value", "minimum value"="Output Minimum Value", "physical channels"=w143) -> ("task out"=w119:refnum<k21>, "error out"=w118:errorcluster)  [unwired: 11 in]
              n64 = Divide(x=w109, y="out/in") -> (x/y=w108:dbl)
              n65 = call-poly <vilib>:"DAQmx Timing.vi"("task/channels in"=w119, "sample mode"=w113, "rate"=w109, "error in"=w118) -> ("task out"=w111:refnum<k21>, "error out"=w110:errorcluster)  [unwired: 10 in]
              n66 = call-poly <vilib>:"DAQmx Timing.vi"("task/channels in"=w117, "sample mode"=w112, "rate"=w108, "error in"=w116) -> ("task out"=w106:refnum<k21>, "error out"=w107:errorcluster)  [unwired: 10 in]
              n67 = Index Array(array="Static Channels", index=0) -> (element=w144:cluster{dbl, string, "Output Channels":tag})
              n68 = Index Array(array="Static Channels", index=1) -> (element=w145:cluster{dbl, string, "Output Channels":tag})
              n69 = Unbundle(w144) -> ("Output Channels"=w150:tag)  [unwired: 2 out]
              n70 = Unbundle(w145) -> ("Output Channels"=w149:tag)  [unwired: 2 out]
              n71 = Concatenate Strings(w150, ",", w149) -> (w151:string)
              n72 = call-poly <vilib>:"DAQmx Create Virtual Channel.vi"("physical channels"=w151) -> ("task out"=w114:refnum<k21>, "error out"=w115:errorcluster)  [unwired: 13 in]
            }
            frame #1 {
              # "clear static"
              # "Static"
              # "Mirrors"
              # "Slow"
              # "Fast"
              # "Data"
              # "Scan\nValues"
              # "Exit"
              # "Switch"
              # "reset DAQ tasks"
              n73 = property on="Scan Lines" class="DigNum (strict)"() -> ("Value"=w169:u32)  [unwired: 2 in, 2 out]
              n74 = property on="Scan Points" class="DigNum (strict)"() -> ("Value"=w168:u32)  [unwired: 2 in, 2 out]
              n75 = while {
                shift-right: [w187] -> w163
                shift-left: w177 -> [w200]
                tunnel: w176 -> [w203]
                tunnel: w175 -> [w202]
                tunnel: w174 -> [w201]
                tunnel: w173 -> [w199]
                tunnel: w172 -> [w198]
                tunnel: w171 -> [w197]
                tunnel: w170 -> [w196]
                tunnel: w169 -> [w195]
                tunnel: w168 -> [w194]
                tunnel: [w189] -> w165
                tunnel: [w188] -> w164
                tunnel: [w186] -> w162
                tunnel: [w185] -> w161
                tunnel: [w184] -> w160
                tunnel: [w183] -> w159
                tunnel: w158 -> [w181]
                tunnel: w157 -> [w180]
                tunnel: [w179] -> w156
                tunnel: [w178] -> w155
                i -> [w182]
                stop <- w193 stop-if-true
                n76 = stacked-sequence {
                  seq-local: [w206 _ _ _] -> [_ w229 w294 w414]
                  seq-local: [_ w228 _ _] -> [_ _ _ w410]
                  seq-local: [_ w227 _ _] -> [_ _ w292 w409]
                  seq-local: [_ w226 _ _] -> [_ _ w293 w408]
                  seq-local: [_ _ w291 _] -> [_ _ _ w407]
                  seq-local: [w204 _ _ _] -> [_ _ _ w420]
                  seq-local: [_ _ w279 _] -> [_ _ _ w392]
                  seq-local: [_ _ w278 _] -> [_ _ _ w391]
                  tunnel: w203 -> [_ _ _ w419]
                  tunnel: w202 -> [_ _ _ w418]
                  tunnel: w201 -> [_ _ _ w416]
                  tunnel: w200 -> [_ _ _ w417]
                  tunnel: w199 -> [_ w230 _ w415]
                  tunnel: w198 -> [_ _ _ w413]
                  tunnel: w197 -> [_ _ _ w412]
                  tunnel: w196 -> [_ _ _ w411]
                  tunnel: w195 -> [_ _ _ w406]
                  tunnel: w194 -> [_ _ _ w405]
                  tunnel: [_ _ _ w404] -> w192
                  tunnel: [_ _ _ w403] -> w191
                  tunnel: [_ _ _ w402] -> w190
                  tunnel: [_ _ _ w401] -> w189
                  tunnel: [_ _ _ w400] -> w188
                  tunnel: [_ _ _ w399] -> w187
                  tunnel: [_ _ _ w398] -> w186
                  tunnel: [_ _ _ w397] -> w185
                  tunnel: [_ _ _ w396] -> w184
                  tunnel: [_ _ _ w395] -> w183
                  tunnel: w182 -> [_ _ _ w394]
                  tunnel: w181 -> [_ _ w282 _]
                  tunnel: w180 -> [_ _ w281 _]
                  tunnel: [_ _ _ w393] -> w179
                  tunnel: [_ _ _ w390] -> w178
                  frame #0 {
                    # "check for whether user wants to scan, move, or do nothing"
                    # "Define Scan parameters"
                    n77 = case shown="False" "Start Scan" {
                      tunnel: [w207 enum16{"Do Nothing", "Scan", "Move"}."Scan" ("Enum")] -> w204
                      frame False {
                        n78 = case shown="True" "Go to Cursor" {
                          tunnel: [enum16{"Do Nothing", "Scan", "Move"}."Do Nothing" ("Enum") enum16{"Do Nothing", "Scan", "Move"}."Move" ("Enum")] -> w207
                          frame False {
                          }
                          frame True {
                          }
                        }
                      }
                      frame True {
                      }
                    }
                    n79 = while {
                      tunnel: [w212] -> w206
                      stop <- TRUE stop-if-true
                      n80 = Bundle("Scanner delay (ms)"="Scanner delay (ms)", "Y Scan size(um)"="Y Scan size(um)", "X Scan size(um)"="X Scan size(um)", "Scan Rate (Hz)"="Scan Rate (Hz)", "Y offset (um)"="Y offset (um)", "X offset (um)"="X offset (um)", "Scan Angle (°)"="Scan Angle (°)", "Conv. (mV/um)"="Conv. (mV/um)", "Lines read"="Lines read", "Scan Lines"="Scan Lines", "Scan Points"="Scan Points") -> (w212:T7)  [unwired: 1 in]
                      n81 = Wait (ms)(milliseconds to wait=u32 100) -> ()  [unwired: 1 out]
                    }
                  }
                  frame #1 {
                    w232 = 0.2 ("value")
                    w277 = 0.8 ("y")
                    # "Generate Slow and Fast raster values and also make Image Data arrays"
                    # "Slow scan array"
                    # "Fast scan array"
                    # "Data Array"
                    n82 = Unbundle By Name(w229) -> ("Scan Rate (Hz)"=w253:dbl, "Y Scan size(um)"=w244:dbl, "Scan Lines"=w245:u32)
                    n83 = Unbundle By Name(w229) -> ("Scan Rate (Hz)"=w265:dbl)
                    n84 = Reciprocal(x=w265) -> (1/x=w266:dbl)
                    n85 = Reciprocal(x=w253) -> (1/x=w254:dbl)
                    n86 = Decrement(x=w245) -> (x-1=w237:u32)
                    n87 = Unbundle By Name(w229) -> ("Scan Rate (Hz)"=w276:dbl, "X Scan size(um)"=w260:dbl)
                    n88 = Compound Arithmetic op=MULTIPLY(w277, w230, w266) -> (w267:dbl)
                    n89 = Compound Arithmetic op=MULTIPLY(w230, w232, w254) -> (w255:dbl)
                    n90 = Bundle By Name(cluster=cluster{"Fs":dbl, "#s":dbl} {"Fs"=1000.0, "#s"=1000.0} ("sampling info"), "Fs"=w237, "#s"=w237) -> (w246:cluster{"Fs":dbl, "#s":dbl})
                    n91 = Multiply(x=2.0, y=w232) -> (x*y=w231:dbl)
                    n92 = Unbundle By Name(w229) -> ("Scan Points"=w236:u32, "Scan Lines"=w235:u32)
                    n93 = Multiply(x=w244, y=0.5) -> (x*y=w243:dbl)
                    n94 = Divide(x=w276, y=w231) -> (x/y=w258:dbl)
                    n95 = Divide(x=w276, y=w277) -> (x/y=w270:dbl)
                    n96 = Bundle By Name(cluster=cluster{"Fs":dbl, "#s":dbl} {"Fs"=1000.0, "#s"=1000.0} ("sampling info"), "Fs"=w230, "#s"=w267) -> (w268:cluster{"Fs":dbl, "#s":dbl})
                    n97 = Bundle By Name(cluster=cluster{"Fs":dbl, "#s":dbl} {"Fs"=1000.0, "#s"=1000.0} ("sampling info"), "Fs"=w230, "#s"=w255) -> (w256:cluster{"Fs":dbl, "#s":dbl})
                    n98 = Multiply(x=w260, y=0.6) -> (x*y=w275:dbl)
                    n99 = Max & Min(x=w236, y=w235) -> (max(x,y)=w234:u32)  [unwired: 1 out]
                    n100 = call <vilib>:"Basic Function Generator.vi"("reset signal"=TRUE, "sampling info"=w246, "signal type"=T6."Sawtooth Wave", "phase"=180.0, "amplitude"=w243, "frequency"=1.0) -> ("signal out"=w239:waveform(dbl))  [unwired: 3 in, 2 out]
                    n101 = Initialize Array(0.0 ("element"), w234, w234) -> (w228:dbl[][])
                    n102 = call <vilib>:"Basic Function Generator.vi"("reset signal"=TRUE, "sampling info"=w268, "signal type"=T6."Sawtooth Wave", "phase"=180.0, "amplitude"=w275, "frequency"=w270) -> ("signal out"=w264:waveform(dbl))  [unwired: 3 in, 2 out]
                    n103 = call <vilib>:"Basic Function Generator.vi"("reset signal"=TRUE, "sampling info"=w256, "signal type"=T6."Sine Wave", "phase"=90.0, "amplitude"=w275, "frequency"=w258) -> ("signal out"=w252:waveform(dbl))  [unwired: 3 in, 2 out]
                    n104 = Unbundle By Name(w239) -> ("Y"=w226:dbl[])
                    n105 = local write "Channel2"(w228) -> ()
                    n106 = Unbundle By Name(w264) -> ("Y"=w241:dbl[])
                    n107 = Unbundle By Name(w252) -> ("Y"=w251:dbl[])
                    n108 = Insert Into Array(array=w241, index=0, new element=w251) -> (w227:dbl[])
                  }
                  frame #2 {
                    w303 = 0.5 ("offset")
                    w295 = dbl[] []
                    # "Calculate Mirror arrays for arbitrary scan angle and x/y offsets"
                    # "Calculate Difference Between Starting Position\nand Ending Position for each Mirror and append\nto Mirror Position Array"
                    n109 = while {
                      tunnel: w294 -> [w385]
                      shift-right: [w353] -> w320
                      shift-left: w295 -> [w356]
                      shift-right: [w354] -> w322
                      shift-left: w295 -> [w355]
                      tunnel: w292 -> [w358]
                      tunnel: w293 -> [w359]
                      i -> [w360]
                      stop <- w388 stop-if-true
                      # "Transform Fast/Slow \nArrays by Scan Angle"
                      # "Why?"
                      # "Generate Voltage Array with Offset"
                      n110 = Unbundle By Name(w385) -> ("Scan Lines"=w386:u32)
                      n111 = Unbundle By Name(w385) -> ("Scanner delay (ms)"=w378:dbl)
                      n112 = Unbundle By Name(w385) -> ("Y offset (um)"=w365:dbl, "X offset (um)"=w375:dbl, "Conv. (mV/um)"=w376:dbl)
                      n113 = Add(x=w378, y=-1.0) -> (x+y=w382:dbl)
                      n114 = Reciprocal(x=180.0 ("value")) -> (1/x=w380:dbl)
                      n115 = Decrement(x=w386) -> (x-1=w389:u32)
                      n116 = Decrement(x=w389) -> (x-1=w387:u32)
                      n117 = Compound Arithmetic op=MULTIPLY(w382, w380, 3.141592653589793) -> (w379:dbl)
                      n118 = Greater Or Equal?(x=w360, y=w387) -> (x >= y?=w388:bool)
                      n119 = Multiply(x=w376, y=0.001) -> (x*y=w361:dbl)
                      n120 = Sine & Cosine(0:w379) -> (1:w364:dbl, 2:w363:dbl)
                      n121 = Negate(x=w375) -> (-x=w362:dbl)
                      n122 = Index Array(array=w359, index=w360) -> (element=w357:dbl)
                      n123 = Multiply(x=w357, y=w363) -> (x*y=w369:dbl)
                      n124 = Multiply(x=w358, y=w364) -> (x*y=w370:dbl[])
                      n125 = Multiply(x=w358, y=w363) -> (x*y=w368:dbl[])
                      n126 = Multiply(x=w357, y=w364) -> (x*y=w366:dbl)
                      n127 = Negate(x=w366) -> (-x=w367:dbl)
                      n128 = Compound Arithmetic op=unknown(w370, w369, w365) -> (w372:dbl[])
                      n129 = Compound Arithmetic op=unknown(w368, w367, w362) -> (w371:dbl[])
                      n130 = Multiply(x=w371, y=w361) -> (x*y=w373:dbl[])
                      n131 = Multiply(x=w372, y=w361) -> (x*y=w374:dbl[])
                      n132 = Insert Into Array(array=w356, new element=w374) -> (w353:dbl[])  [unwired: 1 in]
                      n133 = Insert Into Array(array=w355, new element=w373) -> (w354:dbl[])  [unwired: 1 in]
                    }
                    n134 = local read "Wavelength:"() -> (w285:dbl)
                    n135 = while {
                      tunnel: w285 -> [w339]
                      shift-right: [w339] -> w280
                      shift-left: _ -> [w338]
                      tunnel: [w338] -> w284
                      stop <- TRUE stop-if-true
                    }
                    n136 = Not Equal?(x=w280, y=w284) -> (x != y?=w283:bool)
                    n137 = case shown="True" w283 {
                      tunnel: w282 -> [w324 w333]
                      tunnel: w281 -> [w323 w336]
                      tunnel: [w323 w334] -> w278
                      tunnel: [w324 w331] -> w279
                      tunnel: w280 -> [_ w328]
                      frame False {
                      }
                      frame True {
                        w327 = u16 0 items=["?nm", "?nm/min", "?grating", "?turret", "?gratings"] ("Cmd")
                        w330 = u16 1 items=["nm", "goto", "nm/min", "VIS grating", "IR grating"] ("Cmd")
                        n138 = control-ref of="Busy?"() -> (w325:refnum<vi>)
                        n139 = call "CmdMono.vi"("Busy"=w325, "error in (no error)"=w336, "Wavelength (nm)"=w328, "Cmd"=w330, "Mono Port"=w333) -> ("error out"=w335:errorcluster, "Response"=w329:string, "Mono Port Out"=w332:refnum<visa-resource-name>)  [unwired: 3 in, 1 out]
                        n140 = local write "Done?"(w329) -> ()
                        n141 = call "ReadMono.vi"("Busy"=w325, "error in (no error)"=w335, "Cmd"=w327, "Mono Port"=w332) -> ("error out"=w334:errorcluster, "Response"=w326:string, "Mono Port Out"=w331:refnum<visa-resource-name>)  [unwired: 2 in, 1 out]
                        n142 = local write "Reply"(w326) -> ()
                      }
                    }
                    n143 = Array Size(array=w292) -> (size(s)=w302:i32)
                    n144 = Bundle By Name(cluster=cluster{"Fs":dbl, "#s":dbl} {"Fs"=1000.0, "#s"=1000.0} ("sampling info"), "Fs"=w302, "#s"=w302) -> (w307:cluster{"Fs":dbl, "#s":dbl})
                    n145 = Array Size(array=w322) -> (size(s)=w296:i32)
                    n146 = Array Size(array=w320) -> (size(s)=w319:i32)
                    n147 = Decrement(x=w296) -> (x-1=w300:i32)
                    n148 = Decrement(x=w319) -> (x-1=w315:i32)
                    n149 = call <vilib>:"Basic Function Generator.vi"("offset"=w303, "sampling info"=w307, "signal type"=T6."Sawtooth Wave", "phase"=180.0, "amplitude"=w303, "frequency"=1.0) -> ("signal out"=w305:waveform(dbl))  [unwired: 3 in, 2 out]
                    n150 = Index Array(array=w322, index=w300) -> (element=w310:dbl)
                    n151 = Index Array(array=w322, index=0) -> (element=w301:dbl)
                    n152 = Index Array(array=w320, index=w315) -> (element=w313:dbl)
                    n153 = Index Array(array=w320, index=0) -> (element=w314:dbl)
                    n154 = Unbundle By Name(w305) -> ("Y"=w321:dbl[])
                    n155 = Subtract(x=w301, y=w310) -> (x-y=w311:dbl)
                    n156 = Subtract(x=w314, y=w313) -> (x-y=w312:dbl)
                    n157 = Multiply(x=w321, y=w311) -> (x*y=w299:dbl[])
                    n158 = Multiply(x=w321, y=w312) -> (x*y=w316:dbl[])
                    n159 = Add(x=w299, y=w310) -> (x+y=w298:dbl[])
                    n160 = Add(x=w316, y=w313) -> (x+y=w317:dbl[])
                    n161 = Insert Into Array(array=w322, new element=w298) -> (w290:dbl[])  [unwired: 1 in]
                    n162 = Insert Into Array(array=w320, new element=w317) -> (w289:dbl[])  [unwired: 1 in]
                    n163 = local read "Sm Correction?"() -> (w288:bool)
                    n164 = case shown="True" w288 {
                      tunnel: w290 -> [w341 w349]
                      tunnel: w289 -> [w340 w352]
                      tunnel: [w341 w348] -> w286
                      tunnel: [w340 w347] -> w287
                      tunnel: w280 -> [_ w346]
                      frame False {
                      }
                      frame True {
                        n165 = local read "Vis Grating Correction"() -> (w342:dbl[][])
                        n166 = local read "Volts/pixel y"() -> (w343:dbl)
                        n167 = local read "Volts/pixel  x"() -> (w344:dbl)
                        n168 = call "CalcdeltaV.vi"("Correction"=w342, "nm0"="Positioned Wavelength", "nm in"=w346, "Volts/pixel y"=w343, "Volts/pixel  x"=w344) -> ("DeltaVy"=w351:dbl, "DeltaVx"=w350:dbl)  [unwired: 2 out]
                        n169 = Add(x=w349, y=w350) -> (x+y=w348:dbl[])
                        n170 = Add(x=w351, y=w352) -> (x+y=w347:dbl[])
                      }
                    }
                    n171 = Build Array(w286, w287) -> (w291:dbl[][])
                  }
                  frame #3 {
                    n172 = case shown="\"Scan\"" w420 {
                      tunnel: w419 -> [w433 w557 w1260]
                      tunnel: w418 -> [w432 w556 w1261]
                      tunnel: w417 -> [w476 w558 w1255]
                      tunnel: w416 -> [w480 w555 w1258]
                      tunnel: w415 -> [_ w553 _]
                      tunnel: w414 -> [_ w554 w1267]
                      tunnel: w413 -> [_ w552 _]
                      tunnel: w412 -> [w477 w551 w1257]
                      tunnel: w411 -> [w479 w550 w1259]
                      tunnel: w410 -> [_ w549 _]
                      tunnel: w409 -> [_ w560 w1253]
                      tunnel: w408 -> [_ w548 _]
                      tunnel: w407 -> [_ w559 w1252]
                      tunnel: w406 -> [w438 w562 w1266]
                      tunnel: w405 -> [w439 w561 w1265]
                      tunnel: [w473 w547 w1262] -> w404
                      tunnel: [w473 w546 w1262] -> w403
                      tunnel: [w473 w545 w1262] -> w402
                      tunnel: [w433 w544 w1260] -> w401
                      tunnel: [w431 w543 w1261] -> w400
                      tunnel: [w476 w542 w1254] -> w399
                      tunnel: [w478 w541 w1256] -> w398
                      tunnel: [w477 w540 w1257] -> w397
                      tunnel: [w474 w539 w1264] -> w396
                      tunnel: [w475 w538 w1263] -> w395
                      tunnel: w394 -> [_ _ w1270]
                      tunnel: w392 -> [w422 w537 w1251]
                      tunnel: w391 -> [w421 w536 _]
                      tunnel: [w422 w535 w1251] -> w393
                      tunnel: [w421 w534 _] -> w390
                      frame "Do Nothing", Default {
                        w473 = TRUE ("status")
                        n173 = Merge Errors(w479, w480) -> (w478:errorcluster)
                        n174 = local read "Output 1"() -> (w430:dbl)
                        n175 = local read "Output 2"() -> (w429:dbl)
                        n176 = local read "Auto Update"() -> (w426:bool)
                        n177 = while {
                          tunnel: w430 -> [w494]
                          tunnel: w429 -> [w492]
                          shift-right: [w494] -> w428
                          shift-left: _ -> [w493]
                          tunnel: [w493] -> w436
                          shift-right: [w492] -> w427
                          shift-left: _ -> [w491]
                          tunnel: [w491] -> w434
                          stop <- TRUE stop-if-true
                        }
                        n178 = Not Equal?(x=w436, y=w428) -> (x != y?=w437:bool)
                        n179 = Not Equal?(x=w427, y=w434) -> (x != y?=w435:bool)
                        n180 = Or(x=w437, y=w435) -> (x .or. y?=w424:bool)
                        n181 = local read "Update"() -> (w425:bool)
                        n182 = Select(t=w424, s=w426, f=w425) -> (s? t:f=w423:bool)
                        n183 = case shown="True" w423 {
                          tunnel: w428 -> [_ w488]
                          tunnel: w432 -> [w481 w486]
                          tunnel: w433 -> [_ w485]
                          tunnel: [w481 w484] -> w431
                          tunnel: w427 -> [_ w483]
                          frame False {
                          }
                          frame True {
                            n184 = Bundle("Output 1"=w488, "Output 2"=w483) -> (w489:cluster{"Output 1":dbl, "Output 2":dbl})  [unwired: 1 in]
                            n185 = Cluster To Array(cluster=w489) -> (array=w487:dbl[])
                            n186 = call-poly <vilib>:"DAQmx Write.vi"("task/channels in"=w485, "data"=w487, "error in"=w486) -> ("error out"=w484:errorcluster)  [unwired: 10 in, 2 out]
                            n187 = local write "Update"(FALSE ("Increment")) -> ()
                          }
                        }
                        n188 = property on="Reflection Image" class="IntGraph (strict)"() -> ("Cursor.Cursor Position"=w452:T8)  [unwired: 2 in, 2 out]
                        n189 = property on="Channel2" class="IntGraph (strict)"() -> ("Cursor.Cursor Position"=w451:T8)  [unwired: 2 in, 2 out]
                        n190 = Equal?(x=w451, y=w452) -> (x = y?=w448:cluster{"Cursor X":bool, "Cursor Y":bool})
                        n191 = while {
                          tunnel: w452 -> [w531]
                          tunnel: w451 -> [w533]
                          shift-right: [w533] -> w463
                          shift-left: _ -> [w532]
                          tunnel: [w532] -> w470
                          shift-right: [w531] -> w461
                          shift-left: _ -> [w530]
                          tunnel: [w530] -> w471
                          tunnel: [w528] -> w447
                          tunnel: w448 -> [w528]
                          stop <- TRUE stop-if-true
                        }
                        n192 = Unbundle(w447) -> ("Cursor X"=w446:bool, "Cursor Y"=w445:bool)
                        n193 = Equal?(x=w461, y=w471) -> (x = y?=w464:cluster{"Cursor X":bool, "Cursor Y":bool})
                        n194 = Equal?(x=w463, y=w470) -> (x = y?=w469:cluster{"Cursor X":bool, "Cursor Y":bool})
                        n195 = Unbundle(w469) -> ("Cursor X"=w468:bool, "Cursor Y"=w467:bool)
                        n196 = And(x=w446, y=w445) -> (x .and. y?=w443:bool)
                        n197 = Unbundle(w464) -> ("Cursor X"=w465:bool, "Cursor Y"=w466:bool)
                        n198 = local read "Recenter?"() -> (w440:bool)
                        n199 = And(x=w468, y=w467) -> (x .and. y?=w458:bool)
                        n200 = And(x=w465, y=w466) -> (x .and. y?=w459:bool)
                        n201 = while {
                          tunnel: w463 -> [w527]
                          tunnel: [w527] -> w462
                          tunnel: w461 -> [w526]
                          tunnel: [w526] -> w460
                          tunnel: w459 -> [w524]
                          shift-right: [w524] -> w457
                          shift-left: _ -> [w521]
                          tunnel: w458 -> [w523]
                          shift-right: [w523] -> w455
                          shift-left: _ -> [w522]
                          tunnel: [w522] -> w441
                          tunnel: [w521] -> w442
                          tunnel: [w520] -> w444
                          tunnel: w443 -> [w520]
                          stop <- TRUE stop-if-true
                        }
                        n202 = case shown="True" w440 {
                          tunnel: w439 -> [_ w496]
                          tunnel: w438 -> [_ w497]
                          frame False {
                          }
                          frame True {
                            # "reset cursor position to zero,zero"
                            n203 = Bundle("Value"=w496, "Value"=w497) -> (w500:cluster{"Value":u32, "Value":u32})  [unwired: 1 in]
                            n204 = Divide(x=w500, y=2) -> (x/y=w498:cluster{"Value":dbl, "Value":dbl})
                            n205 = local write "Recenter?"(FALSE ("Recenter?")) -> ()
                            n206 = property on="Channel2" class="IntGraph (strict)"("Cursor.Cursor Position"=w498) -> ()  [unwired: 2 in, 2 out]
                            n207 = property on="Reflection Image" class="IntGraph (strict)"("Cursor.Cursor Position"=w498) -> ()  [unwired: 2 in, 2 out]
                          }
                        }
                        n208 = Exclusive Or(1:w442, 2:w455) -> (0:w454:bool)
                        n209 = Exclusive Or(1:w457, 2:w441) -> (0:w456:bool)
                        n210 = And(x=w441, y=w456) -> (x .and. y?=w449:bool)
                        n211 = And(x=w454, y=w442) -> (x .and. y?=w450:bool)
                        n212 = Compound Arithmetic op=OR(w450, w444, w449) -> (w453:bool)
                        n213 = case shown="False" w453 {
                          tunnel: w462 -> [w501 w517]
                          tunnel: w460 -> [w502 w516]
                          tunnel: w449 -> [_ w515]
                          tunnel: w450 -> [_ w514]
                          tunnel: w442 -> [w509 _]
                          tunnel: w441 -> [w511 _]
                          frame False {
                            n214 = Select(t=0, s=w511, f=1) -> (s? t:f=w504:i32)
                            n215 = Select(t=0, s=w509, f=-1) -> (s? t:f=w503:i32)
                            n216 = Add(x=w504, y=w503) -> (x+y=w505:i32)
                            n217 = case shown="1" w505 {
                              tunnel: w502 -> [_ w512 _]
                              tunnel: w501 -> [_ _ w513]
                              frame 0, Default {
                              }
                              frame 1 {
                                n218 = property on="Channel2" class="IntGraph (strict)"("Cursor.Cursor Position"=w512) -> ()  [unwired: 2 in, 2 out]
                              }
                              frame -1 {
                                n219 = property on="Reflection Image" class="IntGraph (strict)"("Cursor.Cursor Position"=w513) -> ()  [unwired: 2 in, 2 out]
                              }
                            }
                          }
                          frame True {
                            n220 = case shown="True" w514 {
                              tunnel: w517 -> [_ w519]
                              frame False {
                              }
                              frame True {
                                n221 = property on="Reflection Image" class="IntGraph (strict)"("Cursor.Cursor Position"=w519) -> ()  [unwired: 2 in, 2 out]
                              }
                            }
                            n222 = case shown="True" w515 {
                              tunnel: w516 -> [_ w518]
                              frame False {
                              }
                              frame True {
                                n223 = property on="Channel2" class="IntGraph (strict)"("Cursor.Cursor Position"=w518) -> ()  [unwired: 2 in, 2 out]
                              }
                            }
                          }
                        }
                        n224 = Wait (ms)(milliseconds to wait=u32 200) -> ()  [unwired: 1 out]
                        n225 = local read "Switch to Spectral"() -> (w474:bool)
                        n226 = local read "Exit"() -> (w475:bool)
                      }
                      frame "Scan" {
                        # "Mirrors"
                        # "Slow"
                        # "Fast"
                        # "Data"
                        # "Inputs"
                        # "O/I"
                        # "SR*"
                        # "Mirrors"
                        # "Static"
                        n227 = stacked-sequence {
                          seq-local: [_ w605 _] -> [_ _ w1196]
                          tunnel: w562 -> [_ _ w1197]
                          tunnel: w561 -> [_ _ w1198]
                          tunnel: w560 -> [w566 _ _]
                          tunnel: w559 -> [w565 w606 _]
                          tunnel: w558 -> [w564 w622 _]
                          tunnel: w557 -> [_ w620 _]
                          tunnel: w556 -> [_ w621 _]
                          tunnel: w555 -> [_ w623 _]
                          tunnel: w554 -> [_ w618 w1199]
                          tunnel: w553 -> [_ _ _]
                          tunnel: w552 -> [_ w617 _]
                          tunnel: w551 -> [_ w624 _]
                          tunnel: w550 -> [_ w625 _]
                          tunnel: w549 -> [_ w619 _]
                          tunnel: w548 -> [_ _ _]
                          tunnel: [_ w616 _] -> w547
                          tunnel: [_ w615 _] -> w546
                          tunnel: [_ w614 _] -> w545
                          tunnel: [_ w613 _] -> w544
                          tunnel: [_ w612 _] -> w543
                          tunnel: [_ w611 _] -> w542
                          tunnel: [_ w610 _] -> w541
                          tunnel: [_ w609 _] -> w540
                          tunnel: [_ w608 _] -> w539
                          tunnel: [_ w607 _] -> w538
                          tunnel: w537 -> [_ w604 _]
                          tunnel: w536 -> [_ w603 _]
                          tunnel: [_ w602 _] -> w535
                          tunnel: [_ w601 _] -> w534
                          frame #0 {
                            w578 = 0.5 ("offset")
                            # "Move Mirrors To Starting Point of Scan Image"
                            n228 = Array Size(array=w566) -> (size(s)=w577:i32)
                            n229 = Bundle By Name(cluster=cluster{"Fs":dbl, "#s":dbl} {"Fs"=1000.0, "#s"=1000.0} ("sampling info"), "Fs"=w577, "#s"=w577) -> (w582:cluster{"Fs":dbl, "#s":dbl})
                            n230 = call <vilib>:"Basic Function Generator.vi"("offset"=w578, "sampling info"=w582, "signal type"=T6."Sawtooth Wave", "phase"=180.0, "amplitude"=w578, "frequency"=1.0) -> ("signal out"=w580:waveform(dbl))  [unwired: 3 in, 2 out]
                            n231 = Unbundle By Name(w580) -> ("Y"=w597:dbl[])
                            n232 = call-poly <vilib>:"DAQmx Create Virtual Channel.vi"("maximum value"=10.0 ("Maximum Value 2"), "minimum value"=-10.0 ("Minimum Value 2"), "physical channels"="Starting Point") -> ("task out"=w572:refnum<k21>, "error out"=w571:errorcluster)  [unwired: 11 in]
                            n233 = Index Array(array=w565, index (col)=0 ("disabled index (col)")) -> (element=w596:dbl[])  [unwired: 1 in]
                            n234 = call-poly <vilib>:"DAQmx Read.vi"("task/channels in"=w572, "timeout"=10.0, "error in"=w571) -> ("data"=w569:dbl[])  [unwired: 10 in, 2 out]
                            n235 = Index Array(array=w596, index=0) -> (element=w592:dbl)
                            n236 = Index Array(array=w596, index=1) -> (element=w589:dbl)
                            n237 = Index Array(array=w569, index=1) -> (element=w598:dbl)
                            n238 = Index Array(array=w569, index=0) -> (element=w599:dbl)
                            n239 = Subtract(x=w589, y=w598) -> (x-y=w588:dbl)
                            n240 = Subtract(x=w592, y=w599) -> (x-y=w591:dbl)
                            n241 = Multiply(x=w591, y=w597) -> (x*y=w590:dbl[])
                            n242 = Multiply(x=w588, y=w597) -> (x*y=w587:dbl[])
                            n243 = Add(x=w598, y=w587) -> (x+y=w585:dbl[])
                            n244 = Add(x=w599, y=w590) -> (x+y=w586:dbl[])
                            n245 = Build Array(w586, w585) -> (w600:dbl[][])
                            n246 = call-poly <vilib>:"DAQmx Write.vi"("task/channels in"=w564, "auto start"=TRUE, "data"=w600) -> ("task out"=w567:refnum<k21>)  [unwired: 10 in, 2 out]
                            n247 = call <vilib>:"DAQmx Stop Task.vi"("task/channels in"=w567) -> ()  [unwired: 13 in, 2 out]
                          }
                          frame #1 {
                            n248 = while {
                              tunnel: w625 -> [w665]
                              tunnel: w624 -> [w664]
                              tunnel: w623 -> [w663]
                              tunnel: w622 -> [w662]
                              tunnel: w621 -> [w661]
                              tunnel: w620 -> [w660]
                              tunnel: w619 -> [w649]
                              tunnel: w618 -> [w635]
                              tunnel: w617 -> [w657]
                              tunnel: [w646] -> w613
                              tunnel: [w645] -> w612
                              tunnel: [w644] -> w611
                              tunnel: [w642] -> w610
                              tunnel: [w643] -> w609
                              tunnel: [w636] -> w614
                              tunnel: [w640] -> w615
                              tunnel: [w641] -> w616
                              tunnel: [w638] -> w608
                              tunnel: [w639] -> w607
                              tunnel: w606 -> [w637]
                              tunnel: [w636] -> w605
                              tunnel: w604 -> [w629]
                              tunnel: w603 -> [w628]
                              tunnel: [w627] -> w602
                              tunnel: [w626] -> w601
                              stop <- w648 stop-if-true
                              # "Calculate multiplication factor\nConstantly reading lockin, maybe change"
                              # "Exit"
                              # "Switch"
                              # "Reset"
                              # "Stop Scan"
                              # "DAQ Status"
                              # "Mirror Out"
                              # "Img Data"
                              # "Static"
                              # "O/I"
                              # "Images"
                              # "Mirrors"
                              n249 = local read "Preamp Sensitivity"() -> (w632:T3)
                              n250 = local read "Multiply Data?"() -> (w631:bool)
                              n251 = local read "Lockin resource"() -> (w634:refnum<visa-resource-name>)
                              n252 = local read "Configuration"() -> (w633:T4)
                              n253 = call "Calcfactor.vi"("Preamp Sensitivity"=w632, "Configuration 2"=w633, "Multiply Data?"=w631, "Lockin resource"=w634) -> ("Multiplication Factor"=w630:dbl)
                              n254 = property class="DAQmx Timing"(reference=w664, error in=w665) -> (reference out=w671:refnum<k21>, error out=w669:errorcluster, "Sample Clock:Rate"=→"Input rate":dbl)
                              n255 = property class="DAQmx Timing"(reference=w662, error in=w663) -> (reference out=w672:refnum<k21>, error out=w673:errorcluster, "Sample Clock:Rate"=→"Output rate":dbl)
                              n256 = call "Get Terminal Name with Device Prefix.vi"("error in (no error)"=w669, "Local Terminal Name"="ai/StartTrigger" ("terminal"), "task/channels in"=w671) -> ("error out"=w678:errorcluster, "Terminal Name with Device Prefix"=w674:tag, "task out"=w666:refnum<k21>)  [unwired: 6 in]
                              n257 = call-poly <vilib>:"DAQmx Trigger.vi"("task/channels in"=w672, "source"=w674, "error in"=w673) -> ("task out"=w658:refnum<k21>, "error out"=w659:errorcluster)  [unwired: 11 in]
                              n258 = call-poly <vilib>:"DAQmx Write.vi"("task/channels in"=w658, "data"=w637, "timeout"=10.0, "error in"=w659) -> ("task out"=w675:refnum<k21>, "error out"=w676:errorcluster)  [unwired: 9 in, 1 out]
                              n259 = call <vilib>:"DAQmx Start Task.vi"("task/channels in"=w675, "error in"=w676) -> ("task out"=w652:refnum<k21>, "error out"=w677:errorcluster)  [unwired: 12 in]
                              n260 = Merge Errors(w678, w677) -> (w679:errorcluster)
                              n261 = call <vilib>:"DAQmx Start Task.vi"("task/channels in"=w666, "error in"=w679) -> ("task out"=w653:refnum<k21>, "error out"=w656:errorcluster)  [unwired: 12 in]
                              n262 = call <vilib>:"DAQmx Start Task.vi"("task/channels in"=w660, "error in"=w661) -> ("task out"=w654:refnum<k21>, "error out"=w655:errorcluster)  [unwired: 12 in]
                              n263 = while {
                                tunnel: w635 -> [w681]
                                tunnel: w657 -> [w787]
                                tunnel: w652 -> [w797]
                                tunnel: w656 -> [w799]
                                tunnel: w653 -> [w798]
                                tunnel: w655 -> [w782]
                                tunnel: w654 -> [w781]
                                tunnel: [w794] -> w651
                                tunnel: [w780] -> w650
                                shift-right: [w771] -> _
                                shift-left: w649 -> [w774]
                                shift-right: [w772] -> _
                                shift-left: w649 -> [w775]
                                tunnel: ["Reset"] -> w636
                                tunnel: [w769] -> w640
                                tunnel: ["Switch to Spectral"] -> w638
                                shift-right: [w716] -> _
                                shift-left: w630 -> [w715]
                                tunnel: w629 -> [w702]
                                tunnel: w628 -> [w701]
                                tunnel: [w700] -> w627
                                tunnel: [w699] -> w626
                                i -> [w779]
                                stop <- w773 stop-if-true
                                # "Multiply data"
                                # "Update preamp seperately"
                                # "Lines"
                                # "Img Data"
                                # "Delay"
                                # "RIQ"
                                # "Lines Read"
                                # "Points"
                                # "i"
                                n264 = local read "Increment type"() -> (w698:enum16{"Wavelength", "Output1"})
                                n265 = local write "Multiplication Factor"(w715) -> ()
                                n266 = local read "Subfolder(no outside slashes)"() -> (w708:string)
                                n267 = local read "Prepend date folder?"() -> (w707:bool)
                                n268 = local read "Scan base"() -> (w706:path)
                                n269 = Unbundle By Name(w681) -> ("Scan Rate (Hz)"=w790:dbl, "Scan Lines"=w731:u32, "Scan Points"=w732:u32, "Lines read"=w778:u32, "Scanner delay (ms)"=w789:dbl)
                                n270 = Quotient & Remainder(x=w787, y=w790) -> (floor(x/y)=w777:dbl)  [unwired: 1 out]
                                n271 = call "generate filepath.vi"("Filename"="Channel 1 filename", "Subfolder(no outside slashes)"=w708, "Prepend date folder?"=w707, "Scan base"=w706) -> ("path"=w696:path)
                                n272 = call "generate filepath.vi"("Filename"="Channel 2 Filename", "Subfolder(no outside slashes)"=w708, "Prepend date folder?"=w707, "Scan base"=w706) -> ("path"=w695:path)
                                n273 = case shown="True" "Concat" {
                                tunnel: w695 -> [w808 w822]
                                tunnel: w696 -> [w807 w821]
                                tunnel: [w807 w812] -> w693
                                tunnel: [w808 w811] -> w694
                                tunnel: w698 -> [_ w810]
                                frame False {
                                }
                                frame True {
                                n274 = case shown="\"Wavelength\", Default" w810 {
                                tunnel: [w824 w826] -> w823
                                frame "Wavelength", Default {
                                n275 = local read "Wavelength:"() -> (w824:dbl)
                                }
                                frame "Output1" {
                                n276 = local read "Output 1"() -> (w825:dbl)
                                n277 = Compound Arithmetic op=MULTIPLY(w825, 1000) -> (w826:dbl)
                                }
                                }
                                n278 = Strip Path(path=w821) -> (stripped path=w809:path, name=w820:string)
                                n279 = Strip Path(path=w822) -> (stripped path=w818:path, name=w819:string)
                                n280 = Number To Decimal String(number=w823) -> (decimal integer string=w813:string)  [unwired: 1 in]
                                n281 = Concatenate Strings(w820, "_", w813) -> (w816:string)
                                n282 = Concatenate Strings(w819, "_", w813) -> (w817:string)
                                n283 = Build Path(base path=w809, name or relative path=w816) -> (appended path=w812:path)
                                n284 = Build Path(base path=w818, name or relative path=w817) -> (appended path=w811:path)
                                }
                                }
                                n285 = Compound Arithmetic op=MULTIPLY(w777, w778) -> (w786:dbl)
                                n286 = Compound Arithmetic op=MULTIPLY(w787, w789, 0.001 ("value")) -> (w776:dbl)
                                n287 = local write "Channel 2"(w694) -> ()
                                n288 = call-poly <vilib>:"DAQmx Read.vi"("task/channels in"=w798, "number of samples per channel"=w786, "error in"=w799) -> ("data"=w719:dbl[][], "error out"=w796:errorcluster)  [unwired: 10 in, 1 out]
                                n289 = Multiply(x=w715, y=w719) -> (x*y=w718:dbl[][])
                                n290 = Compound Arithmetic op=MULTIPLY(w779, w778) -> (w791:u32)
                                n291 = local write "Channel 1"(w693) -> ()
                                n292 = Divide(x=w791, y=w731) -> (x/y=w792:dbl)
                                n293 = Quotient & Remainder(x=w791, y=w731) -> (floor(x/y)=w793:u32)  [unwired: 1 out]
                                n294 = Equal?(x=w793, y=w792) -> (x = y?=w785:bool)
                                n295 = And(x="Increment", y=w785) -> (x .and. y?=w705:bool)
                                n296 = stacked-sequence {
                                seq-local: [w891 _] -> [_ w1011]
                                seq-local: [w880 _] -> [_ w1010]
                                seq-local: [w879 _] -> [_ w1009]
                                tunnel: w779 -> [w884 _]
                                tunnel: w732 -> [w888 _]
                                tunnel: w778 -> [w883 _]
                                tunnel: w731 -> [w885 w1012]
                                tunnel: w777 -> [w887 _]
                                tunnel: w776 -> [w886 _]
                                tunnel: w718 -> [w890 _]
                                tunnel: w775 -> [w892 _]
                                tunnel: w774 -> [w889 _]
                                tunnel: [_ w1010] -> w772
                                tunnel: [_ w1009] -> w771
                                tunnel: [_ w1008] -> w717
                                tunnel: w681 -> [_ w1007]
                                tunnel: "Preamp Sensitivity" -> [_ w1005]
                                tunnel: [_ w1004] -> w716
                                tunnel: w715 -> [_ w1003]
                                tunnel: w693 -> [_ w1002]
                                tunnel: w694 -> [_ w1001]
                                frame #0 {
                                # "Points"
                                # "RIQ"
                                # "Delay"
                                # "Lines"
                                # "Lines Read"
                                # "i"
                                # "Points"
                                # "RIQ"
                                # "Delay"
                                # "Lines"
                                # "Lines Read"
                                # "i"
                                n297 = while {
                                tunnel: w883 -> [w939]
                                tunnel: w884 -> [w938]
                                tunnel: w885 -> [w940]
                                tunnel: w888 -> [w945]
                                tunnel: w887 -> [w946]
                                tunnel: w886 -> [w951]
                                tunnel: w890 -> [w955]
                                shift-right: [w936] -> w880
                                shift-left: w892 -> [w937]
                                tunnel: [w935] -> w882
                                tunnel: [w934] -> w891
                                tunnel: "Averaging amount Ch1 (4 min)" -> [w933]
                                tunnel: "Average Ch1?" -> [w932]
                                i -> [w941]
                                stop <- w960 stop-if-true
                                n298 = Multiply(x=w938, y=w939) -> (x*y=w942:u32)
                                n299 = Decrement(x=w939) -> (x-1=w959:u32)
                                n300 = Greater Or Equal?(x=w941, y=w959) -> (x >= y?=w960:bool)
                                n301 = Add(x=w942, y=w941) -> (x+y=w958:u32)
                                n302 = Add(x=0.26666 ("value"), y=w941) -> (x+y=w953:dbl)
                                n303 = Quotient & Remainder(x=w958, y=w940) -> (x-y*floor(x/y)=w934:u32)  [unwired: 1 out]
                                n304 = Compound Arithmetic op=MULTIPLY(w953, w946) -> (w952:dbl)
                                n305 = Add(x=w951, y=w952) -> (x+y=w950:dbl)
                                n306 = Negate(x=w950) -> (-x=w949:dbl)
                                n307 = Index Array(array=w955, index (row)=0) -> (element=w956:dbl[])  [unwired: 1 in]
                                n308 = Round To Nearest(number=w949) -> (nearest integer value=w948:dbl)
                                n309 = Rotate 1D Array(1:w956, 2:w948) -> (0:w947:dbl[])
                                n310 = Initialize Array(0.0 ("element"), w945) -> (w944:dbl[])
                                n311 = case shown="False" w932 {
                                tunnel: w947 -> [w964 w983]
                                tunnel: w946 -> [w963 w982]
                                tunnel: w945 -> [w962 w981]
                                tunnel: w944 -> [w961 w980]
                                tunnel: [w965 w979] -> w935
                                tunnel: w933 -> [_ w978]
                                frame False {
                                n312 = while {
                                tunnel: w964 -> [w974]
                                tunnel: w962 -> [w971]
                                tunnel: w963 -> [w976]
                                shift-right: [w969] -> w965
                                shift-left: w961 -> [w968]
                                i -> [w966]
                                stop <- w972 stop-if-true
                                n313 = Decrement(x=w971) -> (x-1=w970:u32)
                                n314 = Greater Or Equal?(x=w966, y=w970) -> (x >= y?=w972:bool)
                                n315 = Compound Arithmetic op=MULTIPLY(0.6666 ("value"), w976, w966) -> (w975:dbl)
                                n316 = Quotient & Remainder(x=w975, y=w971) -> (floor(x/y)=w973:dbl)  [unwired: 1 out]
                                n317 = Index Array(array=w974, index=w973) -> (element=w967:dbl)
                                n318 = Replace Array Subset(array=w968, new element=w967, index=w966) -> (w969:dbl[])
                                }
                                }
                                frame True {
                                n319 = while {
                                tunnel: w983 -> [w991]
                                tunnel: w981 -> [w996]
                                tunnel: w982 -> [w999]
                                shift-right: [w994] -> w979
                                shift-left: w980 -> [w993]
                                tunnel: w978 -> [w984]
                                i -> [w992]
                                stop <- w997 stop-if-true
                                # "pick subset half averaging amount around each point so it doesn't shift"
                                n320 = Decrement(x=w996) -> (x-1=w995:u32)
                                n321 = Greater Or Equal?(x=w992, y=w995) -> (x >= y?=w997:bool)
                                n322 = Compound Arithmetic op=MULTIPLY(0.6666 ("value"), w999, w992) -> (w998:dbl)
                                n323 = Divide(x=w984, y=2) -> (x/y=w986:dbl)
                                n324 = Quotient & Remainder(x=w998, y=w996) -> (floor(x/y)=w987:dbl)  [unwired: 1 out]
                                n325 = Subtract(x=w987, y=w986) -> (x-y=w985:dbl)
                                n326 = Array Subset(array=w991, index=w985, length=w984) -> (w990:dbl[])
                                n327 = call-poly <vilib>:"Mean.vi"("X"=w990) -> ("mean"=w989:dbl)  [unwired: 1 out]
                                n328 = Replace Array Subset(array=w993, new element=w989, index=w992) -> (w994:dbl[])
                                }
                                }
                                }
                                n329 = Replace Array Subset(array=w937, new element=w935, index (col)=w934) -> (w936:dbl[][])  [unwired: 1 in]
                                }
                                "Reflection Image" <- w880
                                "Linescan" <- w882
                                n330 = while {
                                tunnel: w883 -> [w898]
                                tunnel: w884 -> [w897]
                                tunnel: w885 -> [w899]
                                tunnel: w888 -> [w904]
                                tunnel: w887 -> [w905]
                                tunnel: w886 -> [w910]
                                tunnel: w890 -> [w914]
                                shift-right: [w895] -> w879
                                shift-left: w889 -> [w896]
                                tunnel: [w894] -> w881
                                tunnel: [w893] -> _
                                i -> [w900]
                                stop <- w919 stop-if-true
                                n331 = Multiply(x=w897, y=w898) -> (x*y=w901:u32)
                                n332 = Decrement(x=w898) -> (x-1=w918:u32)
                                n333 = Greater Or Equal?(x=w900, y=w918) -> (x >= y?=w919:bool)
                                n334 = Add(x=w901, y=w900) -> (x+y=w917:u32)
                                n335 = Add(x=0.26666 ("value"), y=w900) -> (x+y=w912:dbl)
                                n336 = Quotient & Remainder(x=w917, y=w899) -> (x-y*floor(x/y)=w893:u32)  [unwired: 1 out]
                                n337 = Compound Arithmetic op=MULTIPLY(w912, w905) -> (w911:dbl)
                                n338 = Add(x=w910, y=w911) -> (x+y=w909:dbl)
                                n339 = Negate(x=w909) -> (-x=w908:dbl)
                                n340 = Index Array(array=w914, index (row)=1) -> (element=w915:dbl[])  [unwired: 1 in]
                                n341 = Round To Nearest(number=w908) -> (nearest integer value=w907:dbl)
                                n342 = Rotate 1D Array(1:w915, 2:w907) -> (0:w906:dbl[])
                                n343 = Initialize Array(0.0 ("element"), w904) -> (w903:dbl[])
                                n344 = while {
                                tunnel: w906 -> [w928]
                                tunnel: w904 -> [w925]
                                tunnel: w905 -> [w930]
                                shift-right: [w923] -> w894
                                shift-left: w903 -> [w922]
                                i -> [w920]
                                stop <- w926 stop-if-true
                                n345 = Decrement(x=w925) -> (x-1=w924:u32)
                                n346 = Greater Or Equal?(x=w920, y=w924) -> (x >= y?=w926:bool)
                                n347 = Compound Arithmetic op=MULTIPLY(0.6666 ("value"), w930, w920) -> (w929:dbl)
                                n348 = Quotient & Remainder(x=w929, y=w925) -> (floor(x/y)=w927:dbl)  [unwired: 1 out]
                                n349 = Index Array(array=w928, index=w927) -> (element=w921:dbl)
                                n350 = Replace Array Subset(array=w922, new element=w921, index=w920) -> (w923:dbl[])
                                }
                                n351 = Replace Array Subset(array=w896, new element=w894, index (col)=w893) -> (w895:dbl[][])  [unwired: 1 in]
                                }
                                "Linescan 2" <- w881
                                "Channel2" <- w879
                                }
                                frame #1 {
                                n352 = Decrement(x=w1012) -> (x-1=w1014:u32)
                                n353 = Equal?(x=w1011, y=w1014) -> (x = y?=w1006:bool)
                                n354 = And(x="Save Image", y=w1006) -> (x .and. y?=w1008:bool)
                                n355 = case shown="True" w1008 {
                                tunnel: w1009 -> [_ w1031]
                                tunnel: w1010 -> [_ w1089]
                                tunnel: w1007 -> [_ w1067]
                                tunnel: w1002 -> [_ w1025]
                                tunnel: w1001 -> [_ w1026]
                                frame False {
                                }
                                frame True {
                                w1090 = T9."create or replace" ("function (open:0)")
                                # "multiplication/bias info"
                                # "Confocal parameters"
                                n356 = Unbundle(w1067) -> ("Y Scan size(um)"=w1066:dbl, "X Scan size(um)"=w1065:dbl, "Scan Rate (Hz)"=w1064:dbl, "Scan Angle (°)"=w1063:dbl, "Conv. (mV/um)"=w1062:dbl)  [unwired: 6 out]
                                n357 = Number To Fractional String(number=w1062, precision (6)=i16 3) -> (F-format string=w1078:string)  [unwired: 2 in]
                                n358 = Number To Fractional String(number=w1066, precision (6)=i16 4) -> (F-format string=w1086:string)  [unwired: 2 in]
                                n359 = Number To Fractional String(number=w1065, precision (6)=i16 4) -> (F-format string=w1083:string)  [unwired: 2 in]
                                n360 = Number To Fractional String(number=w1063, precision (6)=i16 3) -> (F-format string=w1079:string)  [unwired: 2 in]
                                n361 = Number To Fractional String(number=w1064, precision (6)=i16 3) -> (F-format string=w1081:string)  [unwired: 2 in]
                                n362 = Concatenate Strings("Y Scan size:" ("string"), w1086) -> (w1076:string)
                                n363 = Concatenate Strings("   Scan Rate:" ("string"), w1081) -> (w1074:string)
                                n364 = Concatenate Strings("   X Scan size: " ("string"), w1083) -> (w1075:string)
                                n365 = Concatenate Strings("    Scan Angle:" ("string"), w1079) -> (w1073:string)
                                n366 = Concatenate Strings("    mV to micron:" ("string"), w1078) -> (w1072:string)
                                n367 = Concatenate Strings(";Confocal Parameters: " ("string"), w1076, w1075, w1074, w1073, w1072) -> (w1023:string)
                                n368 = local read "Preamp Bias (mv)"() -> (w1055:i32)
                                n369 = local read "Preamp Bias on?"() -> (w1056:bool)
                                n370 = local read "Preamp Sensitivity"() -> (w1052:T3)
                                n371 = local read "Output 2"() -> (w1054:dbl)
                                n372 = local read "Output 1"() -> (w1053:dbl)
                                n373 = local read "Configuration"() -> (w1051:T4)
                                n374 = local read "Multiply Data?"() -> (w1050:bool)
                                n375 = Boolean To (0,1)(Boolean=w1056) -> (0, 1=w1034:i16)
                                n376 = Format Into String(w1052) -> (resulting string=w1044:string)  [unwired: 3 in, 1 out]
                                n377 = Boolean To (0,1)(Boolean=w1050) -> (0, 1=w1048:i16)
                                n378 = Format Into String(w1051) -> (resulting string=w1046:string)  [unwired: 3 in, 1 out]
                                n379 = Number To Fractional String(number=w1053) -> (F-format string=w1037:string)  [unwired: 3 in]
                                n380 = Number To Fractional String(number=w1054) -> (F-format string=w1039:string)  [unwired: 3 in]
                                n381 = Number To Decimal String(number=w1055) -> (decimal integer string=w1041:string)  [unwired: 1 in]
                                n382 = Number To Decimal String(number=w1034) -> (decimal integer string=w1043:string)  [unwired: 1 in]
                                n383 = Number To Decimal String(number=w1048) -> (decimal integer string=w1049:string)  [unwired: 1 in]
                                n384 = property on="Increment" class="Bool (strict)"() -> ("Value"=w1088:bool)  [unwired: 2 in, 2 out]
                                n385 = local read "Wavelength:"() -> (w1024:dbl)
                                n386 = Number To Fractional String(number=w1024) -> (F-format string=w1021:string)  [unwired: 3 in]
                                n387 = Concatenate Strings(w1023, "Wavelength:" ("string"), w1021, "    Multiply Data?:" ("string"), w1049, "  Configuration:" ("string"), w1046, "Preamp Sensitivity:" ("string"), w1044, "  Output 1 :" ("string"), w1037, "   Output 2:" ("string"), w1039, "   Preamp Bias:" ("string"), w1041, "   Preamp Bias on: " ("string"), w1043, "                           ;\r\n" ("string")) -> (w1033:string)
                                n388 = call "Read Lockin.vi"("VISA resource name"="Lockin resource", "String"=w1033) -> ("String 2"=w1058:string)
                                n389 = case shown="True" "Save Channel 2?" {
                                tunnel: w1090 -> [_ w1122]
                                tunnel: w1058 -> [_ w1115]
                                tunnel: w1026 -> [_ w1114]
                                tunnel: w1031 -> [_ w1111]
                                tunnel: [FALSE ("error?") w1108] -> w1028
                                frame False {
                                }
                                frame True {
                                w1110 = FALSE ("prepend array or string size? (T)")
                                n390 = call <vilib>:"Open_Create_Replace File.vi"("function (open:0)"=w1122, "file path"=w1114) -> ("error out"=w1117:errorcluster, "refnum"=w1119:refnum<file>)  [unwired: 6 in, 2 out]
                                n391 = Write to Binary File(file (use dialog)=w1119, data=w1115, error in=w1117, 5:w1110) -> (refnum out=w1118:refnum<file>, error out=w1116:errorcluster)  [unwired: 2 in, 1 out]
                                n392 = Array To Spreadsheet String(array=w1111, 3:"%.3e" ("format string")) -> (spreadsheet string=w1112:string)  [unwired: 1 in]
                                n393 = Write to Binary File(file (use dialog)=w1118, data=w1112, error in=w1116, 5:w1110) -> (refnum out=w1120:refnum<file>, error out=w1121:errorcluster)  [unwired: 2 in, 1 out]
                                n394 = Close File(refnum=w1120, error in=w1121) -> (error out=w1109:errorcluster)  [unwired: 1 out]
                                n395 = call <vilib>:"Simple Error Handler.vi"("error in (no error)"=w1109) -> ("error?"=w1108:bool)  [unwired: 4 in, 4 out]
                                }
                                }
                                n396 = case shown="True" "Save Channel 1?" {
                                tunnel: w1090 -> [_ w1106]
                                tunnel: w1089 -> [_ w1101]
                                tunnel: w1058 -> [_ w1095]
                                tunnel: w1025 -> [_ w1094]
                                tunnel: [FALSE ("error?") w1092] -> w1029
                                frame False {
                                }
                                frame True {
                                w1096 = FALSE ("prepend array or string size? (T)")
                                n397 = call <vilib>:"Open_Create_Replace File.vi"("function (open:0)"=w1106, "file path"=w1094) -> ("error out"=w1098:errorcluster, "refnum"=w1100:refnum<file>)  [unwired: 6 in, 2 out]
                                n398 = Write to Binary File(file (use dialog)=w1100, data=w1095, error in=w1098, 5:w1096) -> (refnum out=w1099:refnum<file>, error out=w1097:errorcluster)  [unwired: 2 in, 1 out]
                                n399 = Array To Spreadsheet String(array=w1101, 3:"%.3e" ("format string")) -> (spreadsheet string=w1102:string)  [unwired: 1 in]
                                n400 = Write to Binary File(file (use dialog)=w1099, data=w1102, error in=w1097, 5:w1096) -> (refnum out=w1103:refnum<file>, error out=w1104:errorcluster)  [unwired: 2 in, 1 out]
                                n401 = Close File(refnum=w1103, error in=w1104) -> (error out=w1093:errorcluster)  [unwired: 1 out]
                                n402 = call <vilib>:"Simple Error Handler.vi"("error in (no error)"=w1093) -> ("error?"=w1092:bool)  [unwired: 4 in, 4 out]
                                }
                                }
                                n403 = Or(x=w1029, y=w1028) -> (x .or. y?=w1027:bool)
                                n404 = Or(x=w1027, y=w1088) -> (x .or. y?=w1087:bool)
                                n405 = local write "Save Image"(w1087) -> ()
                                "Channel 2" <- w1026
                                "Channel 1" <- w1025
                                }
                                }
                                n406 = case shown="True" w1006 {
                                tunnel: w1005 -> [_ w1019]
                                tunnel: [w1015 w1016] -> w1004
                                tunnel: w1003 -> [w1015 _]
                                frame False {
                                }
                                frame True {
                                n407 = local read "Lockin resource"() -> (w1017:refnum<visa-resource-name>)
                                n408 = call "Calcfactor.vi"("Preamp Sensitivity"=w1019, "Configuration 2"="Configuration", "Multiply Data?"="Multiply Data?", "Lockin resource"=w1017) -> ("Multiplication Factor"=w1016:dbl)
                                }
                                }
                                }
                                }
                                n409 = call <vilib>:"DAQmx Is Task Done.vi"("task/channels in"=w797, "error in"=w796) -> ("error out"=w795:errorcluster)  [unwired: 11 in, 2 out]
                                n410 = Unbundle By Name(w795) -> ("status"=w767:bool)
                                n411 = call <vilib>:"DAQmx Is Read or Write Late.vi"("error in"=w795) -> ("error out"=w794:errorcluster)  [unwired: 13 in, 1 out]
                                n412 = while {
                                tunnel: "Output 1" -> [w837]
                                tunnel: "Output 2" -> [w835]
                                shift-right: [w837] -> w723
                                shift-left: _ -> [w836]
                                tunnel: [w836] -> w727
                                shift-right: [w835] -> w683
                                shift-left: _ -> [w834]
                                tunnel: [w834] -> w682
                                stop <- TRUE stop-if-true
                                }
                                n413 = case shown="True" w705 {
                                tunnel: w723 -> [w1135 w1145]
                                tunnel: [w1135 w1136] -> w764
                                tunnel: [FALSE w1143] -> w704
                                tunnel: w702 -> [w1133 w1142]
                                tunnel: w701 -> [w1132 w1141]
                                tunnel: [w1133 w1138] -> w700
                                tunnel: [w1132 w1137] -> w699
                                frame False {
                                }
                                frame True {
                                n414 = case shown="\"Wavelength\", Default" "Increment type" {
                                tunnel: w1145 -> [w1146 w1186]
                                tunnel: [w1146 w1185] -> w1136
                                tunnel: [FALSE TRUE] -> w1143
                                tunnel: w1142 -> [w1159 w1181]
                                tunnel: w1141 -> [w1158 w1180]
                                tunnel: "StopPoint" -> [w1152 w1183]
                                tunnel: "stepsize" -> [w1151 w1182]
                                tunnel: [w1150 w1181] -> w1138
                                tunnel: [w1149 w1180] -> w1137
                                frame "Wavelength", Default {
                                w1164 = u16 0 items=["?nm", "?nm/min", "?grating", "?turret", "?gratings"] ("Cmd")
                                w1162 = u16 1 items=["nm", "goto", "nm/min", "VIS grating", "IR grating"] ("Cmd")
                                n415 = control-ref of="Busy?"() -> (w1166:refnum<vi>)
                                n416 = local read "Use PEM?"() -> (w1147:bool)
                                n417 = local read "Wavelength:"() -> (w1153:dbl)
                                n418 = Greater?(x=w1151, y=0) -> (0:w1157:bool)
                                n419 = Less?(x=w1153, y=w1152) -> (x < y?=w1156:bool)
                                n420 = Exclusive Or(1:w1156, 2:w1157) -> (0:w1154:bool)
                                n421 = case shown="False" w1154 {
                                tunnel: w1151 -> [w1176 _]
                                tunnel: w1153 -> [w1177 w1178]
                                tunnel: [w1175 w1178] -> _
                                tunnel: [w1175 w1178] -> w1148
                                frame False {
                                n422 = Compound Arithmetic op=ADD(w1177, w1176) -> (w1175:dbl)
                                }
                                frame True {
                                n423 = local write "Increment"(FALSE ("Increment")) -> ()
                                }
                                }
                                n424 = call "CmdMono.vi"("Busy"=w1166, "error in (no error)"=w1158, "Wavelength (nm)"=w1148, "Cmd"=w1162, "Mono Port"=w1159) -> ("error out"=w1160:errorcluster, "Response"=w1163:string, "Mono Port Out"=w1161:refnum<visa-resource-name>)  [unwired: 3 in, 1 out]
                                n425 = case shown="True" w1147 {
                                tunnel: w1148 -> [_ w1170]
                                frame False {
                                }
                                frame True {
                                n426 = local read "PEM100Setup"() -> (w1174:T1)
                                n427 = Unbundle(w1174) -> ("Address:"=w1173:T2, "Retardation:"=w1172:dbl, "RTD Units"=w1171:u16, "Wave Units"=w1169:u16)  [unwired: 1 out]
                                n428 = Bundle("Address:"=w1173, "Retardation:"=w1172, "RTD Units"=w1171, "Wavelength:"=w1170, "Wave Units"=w1169) -> (w1168:T10)  [unwired: 1 in]
                                n429 = call "HindsPEM100_Setup.vi"("PEM100Setup"=w1168) -> ()  [unwired: 18 in, 1 out]
                                }
                                }
                                n430 = local write "Done?"(w1163) -> ()
                                n431 = call "ReadMono.vi"("Busy"=w1166, "error in (no error)"=w1160, "Cmd"=w1164, "Mono Port"=w1161) -> ("error out"=w1149:errorcluster, "Response"=w1165:string, "Mono Port Out"=w1150:refnum<visa-resource-name>)  [unwired: 2 in, 1 out]
                                n432 = local write "Wavelength:"(w1148) -> ()
                                n433 = local write "Reply"(w1165) -> ()
                                }
                                frame "Output1" {
                                n434 = Greater?(x=w1182, y=0) -> (0:w1190:bool)
                                n435 = Less?(x=w1186, y=w1183) -> (x < y?=w1189:bool)
                                n436 = Exclusive Or(1:w1189, 2:w1190) -> (0:w1187:bool)
                                n437 = case shown="True" w1187 {
                                tunnel: w1182 -> [w1192 _]
                                tunnel: w1186 -> [w1193 w1195]
                                tunnel: [w1191 w1195] -> w1185
                                frame False {
                                n438 = Compound Arithmetic op=ADD(w1193, w1192) -> (w1191:dbl)
                                }
                                frame True {
                                n439 = local write "Increment"(FALSE ("Increment")) -> ()
                                }
                                }
                                }
                                }
                                }
                                }
                                n440 = local write "Output 1"(w764) -> ()
                                n441 = while {
                                tunnel: "Preamp Bias (mv)" -> [w805]
                                shift-right: [w805] -> w686
                                shift-left: _ -> [w804]
                                tunnel: [w804] -> w687
                                tunnel: "Preamp Bias on?" -> [w803]
                                shift-right: [w803] -> w685
                                shift-left: _ -> [w802]
                                tunnel: [w802] -> w689
                                tunnel: "Preamp Sensitivity" -> [w801]
                                shift-right: [w801] -> w684
                                shift-left: _ -> [w800]
                                tunnel: [w800] -> w688
                                stop <- TRUE stop-if-true
                                }
                                n442 = Not Equal?(x=w683, y=w682) -> (x != y?=w721:bool)
                                n443 = Not Equal?(x=w727, y=w723) -> (x != y?=w722:bool)
                                n444 = Compound Arithmetic op=OR(w722, w721) -> (w720:bool)
                                n445 = And(x=w705, y=w704) -> (x .and. y?=w703:bool)
                                n446 = Not Equal?(x=w686, y=w687) -> (x != y?=w714:bool)
                                n447 = Not Equal?(x=w684, y=w688) -> (x != y?=w711:bool)
                                n448 = Not Equal?(x=w685, y=w689) -> (x != y?=w713:bool)
                                n449 = Select(t=w720, s="Auto Update", f="Update") -> (s? t:f=w724:bool)
                                n450 = Compound Arithmetic op=OR(w714, w713, w711) -> (w712:bool)
                                n451 = Or(x=w703, y=w724) -> (x .or. y?=w783:bool)
                                n452 = case shown="True" w712 {
                                tunnel: w686 -> [_ w831]
                                tunnel: w685 -> [_ w830]
                                tunnel: w684 -> [_ w829]
                                tunnel: w711 -> [_ w828]
                                frame False {
                                }
                                frame True {
                                n453 = call "BiasPreamp.vi"("VISA resource name"="Preamp resource", "CHANGE SENS?"=w828, "Sensitivity"=w829, "Bias on"=w830, "Bias Voltage (mv)"=w831) -> ()
                                }
                                }
                                n454 = case shown="True" w783 {
                                tunnel: w764 -> [_ w1130]
                                tunnel: w782 -> [w1123 w1128]
                                tunnel: w781 -> [_ w1127]
                                tunnel: [w1123 w1126] -> w780
                                tunnel: w683 -> [_ w1125]
                                frame False {
                                }
                                frame True {
                                n455 = Bundle("Output 1"=w1130, "Output 2"=w1125) -> (w1131:cluster{"Output 1":dbl, "Output 2":dbl})  [unwired: 1 in]
                                n456 = Cluster To Array(cluster=w1131) -> (array=w1129:dbl[])
                                n457 = local write "Update"(FALSE ("Increment")) -> ()
                                n458 = call-poly <vilib>:"DAQmx Write.vi"("task/channels in"=w1127, "data"=w1129, "error in"=w1128) -> ("error out"=w1126:errorcluster)  [unwired: 10 in, 2 out]
                                }
                                }
                                n459 = property on="Reflection Image" class="IntGraph (strict)"() -> ("Cursor.Cursor Position"=w744:T8)  [unwired: 2 in, 2 out]
                                n460 = property on="Channel2" class="IntGraph (strict)"() -> ("Cursor.Cursor Position"=w743:T8)  [unwired: 2 in, 2 out]
                                n461 = Equal?(x=w743, y=w744) -> (x = y?=w740:cluster{"Cursor X":bool, "Cursor Y":bool})
                                n462 = while {
                                tunnel: w744 -> [w874]
                                tunnel: w743 -> [w876]
                                shift-right: [w876] -> w755
                                shift-left: _ -> [w875]
                                tunnel: [w875] -> w762
                                shift-right: [w874] -> w753
                                shift-left: _ -> [w873]
                                tunnel: [w873] -> w763
                                tunnel: [w871] -> w739
                                tunnel: w740 -> [w871]
                                stop <- TRUE stop-if-true
                                }
                                n463 = case shown="True" "Recenter?" {
                                tunnel: w732 -> [_ w839]
                                tunnel: w731 -> [_ w840]
                                frame False {
                                }
                                frame True {
                                # "reset cursor position to zero,zero"
                                n464 = Bundle("Scan Points"=w839, "Scan Lines"=w840) -> (w843:cluster{"Scan Points":u32, "Scan Lines":u32})  [unwired: 1 in]
                                n465 = Divide(x=w843, y=2) -> (x/y=w841:cluster{"Scan Points":dbl, "Scan Lines":dbl})
                                n466 = local write "Recenter?"(FALSE ("Recenter?")) -> ()
                                n467 = property on="Reflection Image" class="IntGraph (strict)"("Cursor.Cursor Position"=w841) -> ()  [unwired: 2 in, 2 out]
                                n468 = property on="Channel2" class="IntGraph (strict)"("Cursor.Cursor Position"=w841) -> ()  [unwired: 2 in, 2 out]
                                }
                                }
                                n469 = Unbundle(w739) -> ("Cursor X"=w738:bool, "Cursor Y"=w737:bool)
                                n470 = Equal?(x=w753, y=w763) -> (x = y?=w756:cluster{"Cursor X":bool, "Cursor Y":bool})
                                n471 = Equal?(x=w755, y=w762) -> (x = y?=w761:cluster{"Cursor X":bool, "Cursor Y":bool})
                                n472 = Unbundle(w761) -> ("Cursor X"=w760:bool, "Cursor Y"=w759:bool)
                                n473 = And(x=w738, y=w737) -> (x .and. y?=w735:bool)
                                n474 = Unbundle(w756) -> ("Cursor X"=w757:bool, "Cursor Y"=w758:bool)
                                n475 = And(x=w760, y=w759) -> (x .and. y?=w750:bool)
                                n476 = And(x=w757, y=w758) -> (x .and. y?=w751:bool)
                                n477 = while {
                                tunnel: w755 -> [w870]
                                tunnel: [w870] -> w754
                                tunnel: w753 -> [w869]
                                tunnel: [w869] -> w752
                                tunnel: w751 -> [w867]
                                shift-right: [w867] -> w749
                                shift-left: _ -> [w864]
                                tunnel: w750 -> [w866]
                                shift-right: [w866] -> w747
                                shift-left: _ -> [w865]
                                tunnel: [w865] -> w733
                                tunnel: [w864] -> w734
                                tunnel: [w863] -> w736
                                tunnel: w735 -> [w863]
                                stop <- TRUE stop-if-true
                                }
                                n478 = Exclusive Or(1:w734, 2:w747) -> (0:w746:bool)
                                n479 = Exclusive Or(1:w749, 2:w733) -> (0:w748:bool)
                                n480 = And(x=w733, y=w748) -> (x .and. y?=w741:bool)
                                n481 = And(x=w746, y=w734) -> (x .and. y?=w742:bool)
                                n482 = Compound Arithmetic op=OR(w742, w736, w741) -> (w745:bool)
                                n483 = local read "Start Scan"() -> (w770:bool)
                                n484 = case shown="True" w745 {
                                tunnel: w754 -> [w844 w860]
                                tunnel: w752 -> [w845 w859]
                                tunnel: w741 -> [_ w858]
                                tunnel: w742 -> [_ w857]
                                tunnel: w734 -> [w852 _]
                                tunnel: w733 -> [w854 _]
                                frame False {
                                n485 = Select(t=0, s=w854, f=1) -> (s? t:f=w847:i32)
                                n486 = Select(t=0, s=w852, f=-1) -> (s? t:f=w846:i32)
                                n487 = Add(x=w847, y=w846) -> (x+y=w848:i32)
                                n488 = case shown="-1" w848 {
                                tunnel: w845 -> [_ w855 _]
                                tunnel: w844 -> [_ _ w856]
                                frame 0, Default {
                                }
                                frame 1 {
                                n489 = property on="Channel2" class="IntGraph (strict)"("Cursor.Cursor Position"=w855) -> ()  [unwired: 2 in, 2 out]
                                }
                                frame -1 {
                                n490 = property on="Reflection Image" class="IntGraph (strict)"("Cursor.Cursor Position"=w856) -> ()  [unwired: 2 in, 2 out]
                                }
                                }
                                }
                                frame True {
                                n491 = case shown="True" w857 {
                                tunnel: w860 -> [_ w862]
                                frame False {
                                }
                                frame True {
                                n492 = property on="Reflection Image" class="IntGraph (strict)"("Cursor.Cursor Position"=w862) -> ()  [unwired: 2 in, 2 out]
                                }
                                }
                                n493 = case shown="True" w858 {
                                tunnel: w859 -> [_ w861]
                                frame False {
                                }
                                frame True {
                                n494 = property on="Channel2" class="IntGraph (strict)"("Cursor.Cursor Position"=w861) -> ()  [unwired: 2 in, 2 out]
                                }
                                }
                                }
                                }
                                n495 = local read "Exit"() -> (w766:bool)
                                n496 = Not(x=w770) -> (.not. x?=w769:bool)
                                n497 = Compound Arithmetic op=OR(w769, "Switch to Spectral", w767, w717, w766, "Reset") -> (w773:bool)
                              }
                              n498 = call <vilib>:"DAQmx Stop Task.vi"("task/channels in"=w652, "error in"=w651) -> ("task out"=w644:refnum<k21>, "error out"=w647:errorcluster)  [unwired: 12 in]
                              n499 = call <vilib>:"DAQmx Stop Task.vi"("task/channels in"=w653, "error in"=w647) -> ("task out"=w643:refnum<k21>, "error out"=w642:errorcluster)  [unwired: 12 in]
                              n500 = Unbundle By Name(w642) -> ("status"=w641:bool)
                              n501 = call <vilib>:"DAQmx Stop Task.vi"("task/channels in"=w654, "error in"=w650) -> ("task out"=w646:refnum<k21>, "error out"=w645:errorcluster)  [unwired: 12 in]
                              n502 = local read "Exit"() -> (w639:bool)
                              n503 = Compound Arithmetic op=OR(w640, w638, w639, w636) -> (w648:bool)
                            }
                          }
                          frame #2 {
                            # "Reset Boolean"
                            n504 = case shown="True" w1196 {
                              tunnel: w1199 -> [_ w1204]
                              tunnel: w1198 -> [_ w1203]
                              tunnel: w1197 -> [_ w1202]
                              frame False {
                              }
                              frame True {
                                n505 = flat-sequence {
                                tunnel: w1204 -> [w1211]
                                tunnel: w1203 -> [w1205]
                                tunnel: w1202 -> [w1206]
                                tunnel: [w1206] -> w1201
                                tunnel: [w1205] -> w1200
                                tunnel: w1201 -> [w1249]
                                tunnel: w1200 -> [w1250]
                                frame #0 {
                                # "Calculate Offsets from cursor position"
                                n506 = property on="Channel2" class="IntGraph (strict)"() -> ("Cursor.Cursor Position"=w1210:T8)  [unwired: 2 in, 2 out]
                                n507 = Bundle("Value"=w1205, "Value"=w1206) -> (w1225:cluster{"Value":u32, "Value":u32})  [unwired: 1 in]
                                n508 = Unbundle By Name(w1211) -> ("Scan Angle (°)"=w1233:dbl)
                                n509 = Reciprocal(x=180.0 ("value")) -> (1/x=w1231:dbl)
                                n510 = Divide(x=w1225, y=2) -> (x/y=w1230:cluster{"Value":dbl, "Value":dbl})
                                n511 = flat-sequence {
                                tunnel: [w1238] -> w1237
                                tunnel: w1237 -> [w1244]
                                tunnel: w1207 -> [w1243]
                                frame #0 {
                                n512 = local read "X offset (um)"() -> (w1240:dbl)
                                n513 = local read "Y offset (um)"() -> (w1239:dbl)
                                n514 = Bundle("X offset (um)"=w1240, "Y offset (um)"=w1239) -> (w1238:T11)  [unwired: 1 in]
                                }
                                frame #1 {
                                n515 = Subtract(x=w1244, y=w1243) -> (x-y=w1245:cluster{dbl, dbl})
                                n516 = Unbundle(w1245) -> (w1241:dbl, w1242:dbl)
                                n517 = local write "X offset (um)"(w1241) -> ()
                                n518 = local write "Y offset (um)"(w1242) -> ()
                                }
                                }
                                n519 = Compound Arithmetic op=MULTIPLY(w1233, w1231, 3.141592653589793) -> (w1234:dbl)
                                n520 = Subtract(x=w1210, y=w1230) -> (x-y=w1226:T8)
                                n521 = Sine & Cosine(0:w1234) -> (1:w1229:dbl, 2:w1228:dbl)
                                n522 = Divide(x=w1226, y=w1225) -> (x/y=w1227:T8)
                                n523 = Negate(x=w1229) -> (-x=w1212:dbl)
                                n524 = property on="Y Scan size(um)" class="DigNum (strict)"() -> ("Value"=w1209:dbl)  [unwired: 2 in, 2 out]
                                n525 = Multiply(x=w1212, y=w1227) -> (x*y=w1223:T8)
                                n526 = Multiply(x=w1228, y=w1227) -> (x*y=w1224:T8)
                                n527 = Unbundle(w1224) -> ("Cursor X"=w1222:dbl, "Cursor Y"=w1220:dbl)
                                n528 = Unbundle(w1223) -> ("Cursor X"=w1219:dbl, "Cursor Y"=w1221:dbl)
                                n529 = Negate(x=w1209) -> (-x=w1213:dbl)
                                n530 = property on="X Scan size(um)" class="DigNum (strict)"() -> ("Value"=w1208:dbl)  [unwired: 2 in, 2 out]
                                n531 = Add(x=w1221, y=w1222) -> (x+y=w1215:dbl)
                                n532 = Negate(x=w1219) -> (-x=w1218:dbl)
                                n533 = Add(x=w1218, y=w1220) -> (x+y=w1214:dbl)
                                n534 = Bundle("Value"=w1208, w1213) -> (w1216:cluster{"Value":dbl, dbl})  [unwired: 1 in]
                                n535 = Bundle(w1215, w1214) -> (w1217:cluster{dbl, dbl})  [unwired: 1 in]
                                n536 = Multiply(x=w1217, y=w1216) -> (x*y=w1207:cluster{dbl, dbl})
                                }
                                frame #1 {
                                # "Rezero Cursor after offset calculation"
                                n537 = Bundle("Value"=w1250, "Value"=w1249) -> (w1248:cluster{"Value":u32, "Value":u32})  [unwired: 1 in]
                                n538 = Divide(x=w1248, y=2) -> (x/y=w1246:cluster{"Value":dbl, "Value":dbl})
                                n539 = property on="Channel2" class="IntGraph (strict)"("Cursor.Cursor Position"=w1246) -> ()  [unwired: 2 in, 2 out]
                                n540 = property on="Reflection Image" class="IntGraph (strict)"("Cursor.Cursor Position"=w1246) -> ()  [unwired: 2 in, 2 out]
                                }
                                }
                              }
                            }
                          }
                        }
                      }
                      frame "Move" {
                        w1269 = -1
                        # "watch for switch/exit\ncmd"
                        # "Control code execution with +/- 1\nbased on loop #"
                        n541 = Power Of X(1:w1269, 2:w1270) -> (0:w1268:dbl)
                        n542 = Equal?(x=w1268, y=w1269) -> (x = y?=w1271:bool)
                        n543 = case shown="True" w1271 {
                          selector: w1271 -> [w1273 w1315]
                          tunnel: w1267 -> [w1276 w1323]
                          tunnel: w1266 -> [w1275 w1319]
                          tunnel: w1265 -> [w1274 w1321]
                          tunnel: [w1273 w1315] -> w1262
                          tunnel: w1255 -> [w1272 w1326]
                          tunnel: [w1272 w1317] -> w1254
                          tunnel: w1253 -> [_ w1325]
                          tunnel: w1252 -> [_ w1324]
                          frame False {
                            # "Send false to stay inside while loop and recalculate\nmirror array with updated x&y offsets"
                            # "First time through, find new x&y offsets corresponding to the cursor position"
                            n544 = property on="Channel2" class="IntGraph (strict)"() -> ("Cursor.Cursor Position"=w1280:T8)  [unwired: 2 in, 2 out]
                            n545 = Bundle("Value"=w1274, "Value"=w1275) -> (w1294:cluster{"Value":u32, "Value":u32})  [unwired: 1 in]
                            n546 = Unbundle By Name(w1276) -> ("Scan Angle (°)"=w1302:dbl)
                            n547 = Reciprocal(x=180.0 ("value")) -> (1/x=w1300:dbl)
                            n548 = Divide(x=w1294, y=2) -> (x/y=w1299:cluster{"Value":dbl, "Value":dbl})
                            n549 = Compound Arithmetic op=MULTIPLY(w1302, w1300, 3.141592653589793) -> (w1303:dbl)
                            n550 = Subtract(x=w1280, y=w1299) -> (x-y=w1295:T8)
                            n551 = Sine & Cosine(0:w1303) -> (1:w1298:dbl, 2:w1297:dbl)
                            n552 = Divide(x=w1295, y=w1294) -> (x/y=w1296:T8)
                            n553 = Negate(x=w1298) -> (-x=w1281:dbl)
                            n554 = Multiply(x=w1281, y=w1296) -> (x*y=w1292:T8)
                            n555 = Multiply(x=w1297, y=w1296) -> (x*y=w1293:T8)
                            n556 = Unbundle(w1293) -> ("Cursor X"=w1291:dbl, "Cursor Y"=w1289:dbl)
                            n557 = Unbundle(w1292) -> ("Cursor X"=w1288:dbl, "Cursor Y"=w1290:dbl)
                            n558 = property on="Y Scan size(um)" class="DigNum (strict)"() -> ("Value"=w1279:dbl)  [unwired: 2 in, 2 out]
                            n559 = Add(x=w1290, y=w1291) -> (x+y=w1284:dbl)
                            n560 = Negate(x=w1288) -> (-x=w1287:dbl)
                            n561 = Add(x=w1287, y=w1289) -> (x+y=w1283:dbl)
                            n562 = Negate(x=w1279) -> (-x=w1282:dbl)
                            n563 = Bundle(w1284, w1283) -> (w1286:cluster{dbl, dbl})  [unwired: 1 in]
                            n564 = property on="X Scan size(um)" class="DigNum (strict)"() -> ("Value"=w1278:dbl)  [unwired: 2 in, 2 out]
                            n565 = Bundle("Value"=w1278, w1282) -> (w1285:cluster{"Value":dbl, dbl})  [unwired: 1 in]
                            n566 = Multiply(x=w1286, y=w1285) -> (x*y=w1277:cluster{dbl, dbl})
                            n567 = flat-sequence {
                              tunnel: [w1307] -> w1306
                              tunnel: w1306 -> [w1313]
                              tunnel: w1277 -> [w1312]
                              frame #0 {
                                n568 = local read "X offset (um)"() -> (w1309:dbl)
                                n569 = local read "Y offset (um)"() -> (w1308:dbl)
                                n570 = Bundle("X offset (um)"=w1309, "Y offset (um)"=w1308) -> (w1307:T11)  [unwired: 1 in]
                              }
                              frame #1 {
                                n571 = Subtract(x=w1313, y=w1312) -> (x-y=w1314:cluster{dbl, dbl})
                                n572 = Unbundle(w1314) -> (w1310:dbl, w1311:dbl)
                                n573 = local write "X offset (um)"(w1310) -> ()
                                n574 = local write "Y offset (um)"(w1311) -> ()
                              }
                            }
                          }
                          frame True {
                            # "Send True to exit while loop and reset Move to Boolean"
                            n575 = flat-sequence {
                              tunnel: w1326 -> [w1327]
                              tunnel: w1325 -> [w1341]
                              tunnel: w1324 -> [w1340]
                              tunnel: w1323 -> [w1338]
                              tunnel: [w1329] -> w1322
                              tunnel: w1321 -> [w1329]
                              tunnel: [w1328] -> w1320
                              tunnel: w1319 -> [w1328]
                              tunnel: [w1327] -> w1318
                              tunnel: w1322 -> [w1375]
                              tunnel: w1320 -> [w1374]
                              tunnel: w1318 -> [w1379]
                              tunnel: [w1379] -> w1317
                              frame #0 {
                                w1352 = 0.5 ("offset")
                                # "Second time through"
                                # "Calculate the new center of the mirror array after being shifted\nby the cursor offset (desired move to location). The pair of\nvoltages are found by calculating 1250*Scanlines*0.5 + 1250*0.6\n1250 is the size of the fast array and 0.6 is the middle of the image\nfrom a raster line"
                                # "Move Mirrors To Cursor offset"
                                n576 = Array Size(array=w1341) -> (size(s)=w1332:i32)
                                n577 = Unbundle By Name(w1338) -> ("Scan Lines"=w1334:u32)
                                n578 = local read "Starting Point"() -> (w1339:tag)
                                n579 = Compound Arithmetic op=MULTIPLY(0.5 ("y"), w1334, w1332) -> (w1330:dbl)
                                n580 = Compound Arithmetic op=MULTIPLY(w1332, 0.6 ("y")) -> (w1331:dbl)
                                n581 = Bundle By Name(cluster=cluster{"Fs":dbl, "#s":dbl} {"Fs"=1000.0, "#s"=1000.0} ("sampling info"), "Fs"=w1332, "#s"=w1332) -> (w1356:cluster{"Fs":dbl, "#s":dbl})
                                n582 = Compound Arithmetic op=ADD(w1330, w1331) -> (w1336:dbl)
                                n583 = call-poly <vilib>:"DAQmx Create Virtual Channel.vi"("maximum value"=10.0 ("Maximum Value 2"), "minimum value"=-10.0 ("Minimum Value 2"), "physical channels"=w1339) -> ("task out"=w1347:refnum<k21>, "error out"=w1346:errorcluster)  [unwired: 11 in]
                                n584 = call <vilib>:"Basic Function Generator.vi"("offset"=w1352, "sampling info"=w1356, "signal type"=T6."Sawtooth Wave", "phase"=180.0, "amplitude"=w1352, "frequency"=1.0) -> ("signal out"=w1354:waveform(dbl))  [unwired: 3 in, 2 out]
                                n585 = Round To Nearest(number=w1336) -> (nearest integer value=w1337:dbl)
                                n586 = Unbundle By Name(w1354) -> ("Y"=w1370:dbl[])
                                n587 = Index Array(array=w1340, index (col)=w1337) -> (element=w1369:dbl[])  [unwired: 1 in]
                                n588 = call-poly <vilib>:"DAQmx Read.vi"("task/channels in"=w1347, "timeout"=10.0, "error in"=w1346) -> ("data"=w1344:dbl[])  [unwired: 10 in, 2 out]
                                n589 = Index Array(array=w1369, index=0) -> (element=w1366:dbl)
                                n590 = Index Array(array=w1369, index=1) -> (element=w1363:dbl)
                                n591 = Index Array(array=w1344, index=1) -> (element=w1371:dbl)
                                n592 = Index Array(array=w1344, index=0) -> (element=w1372:dbl)
                                n593 = Subtract(x=w1363, y=w1371) -> (x-y=w1362:dbl)
                                n594 = Subtract(x=w1366, y=w1372) -> (x-y=w1365:dbl)
                                n595 = Multiply(x=w1365, y=w1370) -> (x*y=w1364:dbl[])
                                n596 = Multiply(x=w1362, y=w1370) -> (x*y=w1361:dbl[])
                                n597 = Add(x=w1371, y=w1361) -> (x+y=w1359:dbl[])
                                n598 = Add(x=w1372, y=w1364) -> (x+y=w1360:dbl[])
                                n599 = Build Array(w1360, w1359) -> (w1373:dbl[][])
                                n600 = call-poly <vilib>:"DAQmx Write.vi"("task/channels in"=w1327, "auto start"=TRUE, "data"=w1373) -> ("task out"=w1342:refnum<k21>)  [unwired: 10 in, 2 out]
                                n601 = call <vilib>:"DAQmx Stop Task.vi"("task/channels in"=w1342) -> ()  [unwired: 13 in, 2 out]
                              }
                              frame #1 {
                                # "reset cursor position to zero,zero\nthis is optional, could get rid of based on preference"
                                n602 = Bundle("Value"=w1375, "Value"=w1374) -> (w1378:cluster{"Value":u32, "Value":u32})  [unwired: 1 in]
                                n603 = Divide(x=w1378, y=2) -> (x/y=w1376:cluster{"Value":dbl, "Value":dbl})
                                n604 = property on="Channel2" class="IntGraph (strict)"("Cursor.Cursor Position"=w1376) -> ()  [unwired: 2 in, 2 out]
                                n605 = property on="Reflection Image" class="IntGraph (strict)"("Cursor.Cursor Position"=w1376) -> ()  [unwired: 2 in, 2 out]
                              }
                            }
                            n606 = Not(x=w1315) -> (.not. x?=w1316:bool)
                            n607 = local write "Go to Cursor"(w1316) -> ()
                          }
                        }
                        n608 = Merge Errors(w1259, w1258) -> (w1256:errorcluster)
                        n609 = local read "Switch to Spectral"() -> (w1264:bool)
                        n610 = local read "Exit"() -> (w1263:bool)
                      }
                    }
                  }
                }
                n611 = Compound Arithmetic op=OR(w192, w191, w190, w184, w183) -> (w193:bool)
              }
              n612 = call <vilib>:"DAQmx Clear Task.vi"("task in"=w161, "error in"=w162) -> ("error out"=w167:errorcluster)  [unwired: 13 in]
              n613 = call <vilib>:"DAQmx Clear Task.vi"("task in"=w165, "error in"=w164) -> ()  [unwired: 13 in, 1 out]
              n614 = call <vilib>:"DAQmx Clear Task.vi"("task in"=w163, "error in"=w167) -> ("error out"=w166:errorcluster)  [unwired: 13 in]
              n615 = call <vilib>:"General Error Handler.vi"("error in (no error)"=w166) -> ()  [unwired: 10 in, 5 out]
            }
          }
          n616 = Compound Arithmetic op=OR(w103, w104) -> (w105:bool)
        }
        n617 = case shown="True" w94 {
          tunnel: [enum32{"Imaging", "Spectral"}."Imaging" ("Tab Control") w98] -> w95
          frame False {
          }
          frame True {
            w98 = enum32{"Imaging", "Spectral"}."Spectral" ("Tab Control")
            n618 = local write "Switch to Spectral"(FALSE ("Switch to Spectral")) -> ()
            n619 = property on="Tab Control" class="TabCtl (strict)"("Value"=w98) -> ()  [unwired: 2 in, 2 out]
          }
        }
      }
      frame "Spectral" {
        w1386 = dbl[] []
        w1391 = dbl[] []
        # "Time array"
        # "Scan array"
        # "Static Output Voltages"
        # "Check if tabs need to be switched\nand change if necessary"
        # "Mono"
        # "Input Voltage"
        # "Static Voltages"
        # "Mono"
        n620 = local read "Static Channels"() -> (w1383:cluster{dbl, string, "Output Channels":tag}[])
        n621 = Get Date/Time In Seconds() -> (seconds since 1Jan1904=→"Record Start":timestamp)
        n622 = local write "Power Meter Initalized?"(FALSE ("Power Meter Initalized?")) -> ()
        n623 = local write "Measuring?"(FALSE ("Measuring?")) -> ()
        n624 = Index Array(array=w1383, index=0) -> (element=w1398:cluster{dbl, string, "Output Channels":tag})
        n625 = Index Array(array=w1383, index=1) -> (element=w1399:cluster{dbl, string, "Output Channels":tag})
        n626 = call-poly <vilib>:"DAQmx Create Virtual Channel.vi"("maximum value"=10.0, "minimum value"=-10.0, "physical channels"="Input Channel") -> ("task out"=w1409:refnum<k21>, "error out"=w1408:errorcluster)  [unwired: 11 in]
        n627 = Unbundle(w1398) -> ("Output Channels"=w1380:tag)  [unwired: 2 out]
        n628 = call-poly <vilib>:"DAQmx Create Virtual Channel.vi"("maximum value"=10.0, "minimum value"=-10.0, "physical channels"=w1380) -> ("task out"=w1381:refnum<k21>, "error out"=w1407:errorcluster)  [unwired: 11 in]
        n629 = Unbundle(w1399) -> ("Output Channels"=w1397:tag)  [unwired: 2 out]
        n630 = call-poly <vilib>:"DAQmx Create Virtual Channel.vi"("maximum value"=10.0, "minimum value"=-10.0, "physical channels"=w1397) -> ("task out"=w1382:refnum<k21>, "error out"=w1406:errorcluster)  [unwired: 11 in]
        n631 = Build Array(w1391, w1391) -> (w1390:dbl[][])
        n632 = Build Array(w1386, w1386) -> (w1385:dbl[][])
        n633 = while {
          tunnel: w1394 -> [w1496]
          tunnel: [w1494] -> w1393
          tunnel: [w1454] -> _
          shift-right: [w1489] -> w1410
          shift-left: w1409 -> [w1476]
          shift-right: [w1488] -> w1411
          shift-left: w1408 -> [w1475]
          shift-right: [w1493] -> w1419
          shift-left: w1381 -> [w1487]
          shift-right: [w1492] -> w1418
          shift-left: w1407 -> [w1486]
          shift-right: [w1490] -> w1416
          shift-left: w1382 -> [w1485]
          shift-right: [w1491] -> w1417
          shift-left: w1406 -> [w1484]
          shift-right: [w1483] -> w1392
          shift-left: w1395 -> [w1495]
          shift-right: [w1453] -> _
          shift-left: _ -> [w1466]
          shift-right: [w1480] -> _
          shift-left: "" -> [w1481]
          tunnel: ["Switch to Imaging"] -> w1404
          shift-right: [w1426] -> _
          shift-left: w1390 -> [w1439]
          shift-right: [w1435] -> _
          shift-left: w1385 -> [w1438]
          shift-right: [w1425] -> _
          shift-left: _ -> [w1434]
          stop <- w1479 stop-if-true
          # "Time"
          # "Raw"
          # "Normalized"
          # "new scan"
          # "PM error"
          # "Set up AI"
          # "Close power meter if not being used and initialized"
          # "Only initalize power meter if it is selected and not already initalized"
          n634 = local read "Power"() -> (w1461:bool)
          n635 = Not(x="Power Meter Initalized?") -> (.not. x?=w1463:bool)
          n636 = local read "Input Channel"() -> (w1472:tag)
          n637 = And(x=w1463, y=w1461) -> (x .and. y?=w1462:bool)
          n638 = case shown="True" w1462 {
            tunnel: [w1592 w1596] -> w1468
            tunnel: "Power Meter" -> [w1592 w1595]
            tunnel: [w1591 w1594] -> w1465
            tunnel: w1466 -> [w1591 _]
            frame False {
            }
            frame True {
              # "PM"
              n639 = local write "Power Meter Initalized?"(TRUE ("Power Meter Initalized?")) -> ()
              n640 = call "NoPopup_PM100D_Initialize.vi"("PM Channel"=w1595) -> ("error out"=w1600:errorcluster, "Instrument"=→"IDN String":string, "VISA out"=w1601:refnum<visa-resource-name>)  [unwired: 1 in, 1 out]
              n641 = call "PM100D_SensorFlag.vi"("error in (no error)"=w1600, "VISA in"=w1601) -> ("error out"=w1594:errorcluster, "VISA out"=w1596:refnum<visa-resource-name>, "sn"=→"Sensor SN":string, "name"=→"Sensor Name":string)  [unwired: 2 in, 4 out]
            }
          }
          n642 = local read "Power Meter Initalized?"() -> (→"Power meter initalized?":bool)
          n643 = while {
            tunnel: w1472 -> [w1604]
            shift-right: [w1604] -> w1469
            shift-left: _ -> [w1603]
            tunnel: [w1603] -> w1470
            stop <- TRUE stop-if-true
          }
          n644 = Not Equal?(x=w1470, y=w1469) -> (x != y?=w1471:bool)
          n645 = case shown="True" w1471 {
            tunnel: w1476 -> [w1605 w1613]
            tunnel: w1475 -> [w1606 w1612]
            tunnel: [w1606 w1609] -> w1474
            tunnel: [w1605 w1608] -> w1473
            tunnel: w1469 -> [_ w1607]
            frame False {
            }
            frame True {
              n646 = call <vilib>:"DAQmx Clear Task.vi"("task in"=w1613, "error in"=w1612) -> ()  [unwired: 13 in, 1 out]
              n647 = call-poly <vilib>:"DAQmx Create Virtual Channel.vi"("maximum value"=10.0, "minimum value"=-10.0, "physical channels"=w1607) -> ("task out"=w1608:refnum<k21>, "error out"=w1609:errorcluster)  [unwired: 11 in]
            }
          }
          n648 = stacked-sequence {
            seq-local: [w1615 _ _] -> [_ _ w1893]
            seq-local: [w1614 _ _] -> [_ _ w1892]
            seq-local: [_ w1765 _] -> [_ _ w1889]
            seq-local: [_ w1766 _] -> [_ _ w1890]
            seq-local: [_ w1767 _] -> [_ _ w1891]
            seq-local: [_ w1764 _] -> [_ _ w1894]
            seq-local: [_ w1763 _] -> [_ _ w1895]
            tunnel: w1496 -> [w1652 _ w1878]
            tunnel: w1495 -> [w1651 _ _]
            tunnel: [w1641 _ _] -> w1492
            tunnel: [w1642 _ _] -> w1493
            tunnel: w1468 -> [_ w1773 _]
            tunnel: w1465 -> [_ w1772 _]
            tunnel: w1481 -> [_ w1771 _]
            tunnel: [_ _ w1888] -> w1480
            tunnel: [_ _ w1887] -> w1483
            tunnel: [_ _ w1886] -> w1494
            tunnel: [_ _ w1885] -> w1456
            tunnel: [_ _ w1884] -> w1455
            tunnel: [_ _ w1883] -> w1489
            tunnel: [_ _ w1882] -> w1488
            tunnel: [w1639 _ _] -> w1491
            tunnel: [w1640 _ _] -> w1490
            tunnel: w1473 -> [_ w1752 _]
            tunnel: w1474 -> [_ w1751 _]
            tunnel: w1487 -> [w1638 _ _]
            tunnel: w1486 -> [w1637 _ _]
            tunnel: w1485 -> [w1636 _ _]
            tunnel: w1484 -> [w1635 _ _]
            tunnel: [_ _ w1881] -> w1426
            tunnel: w1439 -> [_ _ w1880]
            tunnel: w1438 -> [_ w1754 _]
            tunnel: [_ w1760 _] -> w1435
            tunnel: [_ _ w1877] -> w1428
            tunnel: w1434 -> [_ _ w1876]
            tunnel: [_ _ w1876] -> w1433
            frame #0 {
              # "wavelength out to next sequence"
              # "Update outputs"
              # "\"Step\" removed for now, don't think it does much more than scan other than it can go down in wavelength"
              # "Update preamp seperate from outputs\nAlso check if sens is changed because of voltage spikes"
              n649 = local read "Preamp Sensitivity"() -> (w1634:T3)
              n650 = local read "Preamp Bias on?"() -> (w1645:bool)
              n651 = local read "Preamp Bias (mv)"() -> (w1643:i32)
              n652 = local read "Output 1"() -> (w1621:dbl)
              n653 = local read "Output 2"() -> (w1620:dbl)
              n654 = while {
                shift-right: [w1689] -> w1617
                shift-left: _ -> [w1688]
                tunnel: w1620 -> [w1689]
                tunnel: [w1688] -> w1616
                tunnel: w1621 -> [w1687]
                shift-right: [w1687] -> w1619
                shift-left: _ -> [w1686]
                tunnel: [w1686] -> w1618
                stop <- TRUE stop-if-true
              }
              n655 = while {
                tunnel: w1643 -> [w1714]
                shift-right: [w1714] -> w1626
                shift-left: _ -> [w1713]
                tunnel: [w1713] -> w1644
                tunnel: w1645 -> [w1712]
                shift-right: [w1712] -> w1625
                shift-left: _ -> [w1711]
                tunnel: [w1711] -> w1646
                tunnel: w1634 -> [w1710]
                shift-right: [w1710] -> w1624
                shift-left: _ -> [w1709]
                tunnel: [w1709] -> w1633
                stop <- TRUE stop-if-true
              }
              n656 = Not Equal?(x=w1626, y=w1644) -> (x != y?=w1629:bool)
              n657 = Not Equal?(x=w1619, y=w1618) -> (x != y?=w1632:bool)
              n658 = Not Equal?(x=w1617, y=w1616) -> (x != y?=w1631:bool)
              n659 = Not Equal?(x=w1624, y=w1633) -> (x != y?=w1623:bool)
              n660 = Not Equal?(x=w1625, y=w1646) -> (x != y?=w1628:bool)
              n661 = Compound Arithmetic op=OR(w1632, w1631) -> (w1630:bool)
              n662 = Compound Arithmetic op=OR(w1629, w1628, w1623) -> (w1627:bool)
              n663 = case shown="True" w1630 {
                tunnel: [w1697 w1708] -> w1641
                tunnel: [w1698 w1707] -> w1642
                tunnel: w1638 -> [w1698 w1700]
                tunnel: w1637 -> [w1697 w1699]
                tunnel: [w1696 w1706] -> w1640
                tunnel: [w1695 w1705] -> w1639
                tunnel: w1619 -> [_ w1704]
                tunnel: w1617 -> [_ w1703]
                tunnel: w1636 -> [w1696 w1702]
                tunnel: w1635 -> [w1695 w1701]
                frame False {
                }
                frame True {
                  n664 = call-poly <vilib>:"DAQmx Write.vi"("task/channels in"=w1700, "data"=w1704, "error in"=w1699) -> ("task out"=w1707:refnum<k21>, "error out"=w1708:errorcluster)  [unwired: 10 in, 1 out]
                  n665 = call-poly <vilib>:"DAQmx Write.vi"("task/channels in"=w1702, "data"=w1703, "error in"=w1701) -> ("task out"=w1706:refnum<k21>, "error out"=w1705:errorcluster)  [unwired: 10 in, 1 out]
                }
              }
              n666 = case shown="True" "Send ?" {
                tunnel: w1652 -> [w1741 w1748]
                tunnel: w1651 -> [w1740 w1747]
                tunnel: [w1740 w1745] -> w1648
                tunnel: [w1741 w1744] -> w1649
                frame False {
                }
                frame True {
                  n667 = control-ref of="Busy?"() -> (w1743:refnum<vi>)
                  n668 = call "ReadMono.vi"("Busy"=w1743, "error in (no error)"=w1747, "Cmd"="Ask?", "Mono Port"=w1748) -> ("error out"=w1745:errorcluster, "Response"=→"Reply":string, "Mono Port Out"=w1744:refnum<visa-resource-name>)  [unwired: 2 in, 1 out]
                }
              }
              n669 = case shown="True" w1627 {
                tunnel: w1626 -> [_ w1693]
                tunnel: w1625 -> [_ w1692]
                tunnel: w1624 -> [_ w1691]
                tunnel: w1623 -> [_ w1690]
                frame False {
                }
                frame True {
                  n670 = local read "Preamp resource"() -> (w1694:refnum<visa-resource-name>)
                  n671 = call "BiasPreamp.vi"("VISA resource name"=w1694, "CHANGE SENS?"=w1690, "Sensitivity"=w1691, "Bias on"=w1692, "Bias Voltage (mv)"=w1693) -> ()
                }
              }
              n672 = case shown="True" "Send CMD" {
                tunnel: w1649 -> [w1724 w1735]
                tunnel: w1648 -> [w1723 w1736]
                tunnel: [w1724 w1732] -> w1615
                tunnel: [w1723 w1731] -> w1614
                frame False {
                }
                frame True {
                  w1737 = u16 0 items=["?nm", "?nm/min", "?grating", "?turret", "?gratings"] ("Cmd")
                  # "If the grating changes reset the scan parameters"
                  n673 = control-ref of="Busy?"() -> (w1728:refnum<vi>)
                  n674 = call "CmdMono.vi"("Busy"=w1728, "Scan Speed (nm/min)"="Speed (nm/min)", "error in (no error)"=w1736, "Wavelength (nm)"="Wavelength:", "Cmd"="CMD", "Mono Port"=w1735) -> ("error out"=w1733:errorcluster, "Response"=→"Done?":string, "Mono Port Out"=w1734:refnum<visa-resource-name>)  [unwired: 2 in, 1 out]
                  n675 = case shown="3" "CMD" {
                    frame 0, Default {
                    }
                    frame 3 {
                      n676 = local write "Reset Params"(TRUE ("Reset Params")) -> ()
                    }
                    frame 4 {
                      n677 = local write "Reset Params"(TRUE ("Reset Params")) -> ()
                    }
                  }
                  n678 = call "ReadMono.vi"("Busy"=w1728, "error in (no error)"=w1733, "Cmd"=w1737, "Mono Port"=w1734) -> ("error out"=w1731:errorcluster, "Response"=w1727:string, "Mono Port Out"=w1732:refnum<visa-resource-name>)  [unwired: 2 in, 1 out]
                  n679 = local write "Reply"(w1727) -> ()
                }
              }
              n680 = disable-structure shown="Disabled" {
                disable-tunnel: _ -> [w1662 _]
                disable-tunnel: _ -> [w1661 _]
                disable-tunnel: _ -> [w1660 _]
                disable-tunnel: [w1659 _] -> _
                disable-tunnel: [w1658 _] -> _
                disable-tunnel: [w1657 _] -> _
                disable-tunnel: FALSE -> [w1656 _]
                frame Disabled {
                  # "wavelength"
                  n681 = case shown="True" w1656 {
                    tunnel: w1662 -> [w1663 w1680]
                    tunnel: w1661 -> [w1665 w1679]
                    tunnel: w1660 -> [w1664 w1678]
                    tunnel: [w1663 w1673] -> w1657
                    tunnel: [w1665 w1671] -> w1659
                    tunnel: [w1664 w1670] -> w1658
                    frame False {
                    }
                    frame True {
                      w1667 = u16 1 items=["nm", "goto", "nm/min", "VIS grating", "IR grating"] ("Cmd")
                      w1675 = u16 0 items=["?nm", "?nm/min", "?grating", "?turret", "?gratings"] ("Cmd")
                      # "increment"
                      # "up/down"
                      n682 = control-ref of="Busy?"() -> (w1672:refnum<vi>)
                      n683 = Select(t=1, s=TRUE ("Up"), f=-1) -> (s? t:f=w1684:i32)
                      n684 = Compound Arithmetic op=MULTIPLY(w1684, 10.0 ("Inc. (nm)")) -> (w1681:dbl)
                      n685 = Compound Arithmetic op=ADD(w1681, w1680) -> (w1673:dbl)
                      n686 = call "CmdMono.vi"("Busy"=w1672, "error in (no error)"=w1678, "Wavelength (nm)"=w1673, "Cmd"=w1667, "Mono Port"=w1679) -> ("error out"=w1676:errorcluster, "Response"=w1668:string, "Mono Port Out"=w1677:refnum<visa-resource-name>)  [unwired: 3 in, 1 out]
                      n687 = local write "Done?"(w1668) -> ()
                      n688 = call "ReadMono.vi"("Busy"=w1672, "error in (no error)"=w1676, "Cmd"=w1675, "Mono Port"=w1677) -> ("error out"=w1670:errorcluster, "Response"=w1669:string, "Mono Port Out"=w1671:refnum<visa-resource-name>)  [unwired: 2 in, 1 out]
                      n689 = local write "Reply"(w1669) -> ()
                    }
                  }
                }
                frame Enabled {
                }
              }
              n690 = event shown="[2] \"Current\": Mouse Down?" {
                selector: _ -> [_ _ _ _]
                dyn-events: _ -> [_ _ _ _]
                timeout: 0 -> [_ _ _ _]
                event Timeout {
                  n691 = event-data() -> ()  [unwired: 1 in, 2 out]
                }
                event "Power": Mouse Down? {
                  n692 = event-data() -> ()  [unwired: 1 in, 7 out]
                  n693 = local read "Power"() -> (w1716:bool)
                  n694 = case shown="False" w1716 {
                    selector: w1716 -> [w1718 _]
                    frame False {
                      w1717 = "Power (W)" ("Y Scale.Name Label.Text")
                      n695 = local write "Current"(w1718) -> ()
                      n696 = property on="ScanGraph" class="XYGraph (strict)"("YScale.NameLbl.Text"=w1717) -> ()  [unwired: 2 in, 2 out]
                      n697 = property on="Waveform Chart" class="WFChart (strict)"("YScale.NameLbl.Text"=w1717) -> ()  [unwired: 2 in, 2 out]
                    }
                    frame True {
                    }
                  }
                  n698 = event-data("Discard?"=w1716) -> ()  [unwired: 1 in, 1 out]
                }
                event "Current": Mouse Down? {
                  n699 = event-data() -> ()  [unwired: 1 in, 7 out]
                  n700 = local read "Current"() -> (w1719:bool)
                  n701 = case shown="False" w1719 {
                    selector: w1719 -> [w1721 _]
                    frame False {
                      w1720 = "Current (A)" ("Y Scale.Name Label.Text")
                      n702 = local write "Power"(w1721) -> ()
                      n703 = property on="ScanGraph" class="XYGraph (strict)"("YScale.NameLbl.Text"=w1720) -> ()  [unwired: 2 in, 2 out]
                      n704 = property on="Waveform Chart" class="WFChart (strict)"("YScale.NameLbl.Text"=w1720) -> ()  [unwired: 2 in, 2 out]
                    }
                    frame True {
                    }
                  }
                  n705 = event-data("Discard?"=w1719) -> ()  [unwired: 1 in, 1 out]
                }
                event "Send CMD": Mouse Up {
                  n706 = event-data() -> ()  [unwired: 1 in, 7 out]
                  n707 = local write "Done?"("   ..." ("Done?")) -> ()
                }
              }
              n708 = disable-structure shown="Disabled" {
                frame Disabled {
                  n709 = event shown="[1] \"Send CMD\": Mouse Up" {
                    selector: _ -> [_ _]
                    dyn-events: _ -> [_ _]
                    timeout: 0 -> [_ _]
                    event Timeout {
                      n710 = event-data() -> ()  [unwired: 1 in, 2 out]
                    }
                    event "Send CMD": Mouse Up {
                      n711 = event-data() -> ()  [unwired: 1 in, 1 out]
                      n712 = local write "Done?"("   ..." ("Done?")) -> ()
                    }
                  }
                }
                frame Enabled {
                }
              }
            }
            frame #1 {
              # "AI"
              # "Power meter"
              # "if not reading current power gets passed through"
              n713 = case shown="True" "Calculate current offset" {
                tunnel: w1752 -> [w1775 w1779]
                tunnel: w1751 -> [w1774 w1778]
                tunnel: [w1775 w1781] -> w1750
                tunnel: [w1774 w1780] -> w1749
                frame False {
                }
                frame True {
                  w1795 = 10178 items=["Finite Samples"=10178, "Continuous Samples"=10123, "Hardware Timed Single Point"=12522] ("sample mode")
                  # "Cant change from 50?"
                  n714 = local read "Preamp Sensitivity"() -> (w1787:T3)
                  n715 = local read "Lockin resource"() -> (w1786:refnum<visa-resource-name>)
                  n716 = call-poly <vilib>:"DAQmx Timing.vi"("task/channels in"=w1779, "sample mode"=w1795, "samples per channel"=50, "rate"=1000.0, "error in"=w1778) -> ("task out"=w1796:refnum<k21>, "error out"=w1797:errorcluster)  [unwired: 9 in]
                  n717 = local read "Multiply Data?"() -> (w1788:bool)
                  n718 = local read "Configuration"() -> (w1789:T4)
                  n719 = call <vilib>:"DAQmx Start Task.vi"("task/channels in"=w1796, "error in"=w1797) -> ("task out"=w1791:refnum<k21>, "error out"=w1790:errorcluster)  [unwired: 12 in]
                  n720 = call-poly <vilib>:"DAQmx Read.vi"("task/channels in"=w1791, "error in"=w1790) -> ("task out"=w1793:refnum<k21>, "data"=w1777:dbl[], "error out"=w1792:errorcluster)  [unwired: 11 in]
                  n721 = call "Calcfactor.vi"("Preamp Sensitivity"=w1787, "Configuration 2"=w1789, "Multiply Data?"=w1788, "Lockin resource"=w1786) -> ("Multiplication Factor"=w1784:dbl)
                  n722 = call-poly <vilib>:"Mean.vi"("X"=w1777) -> ("mean"=w1785:dbl)  [unwired: 1 out]
                  n723 = call <vilib>:"DAQmx Stop Task.vi"("task/channels in"=w1793, "error in"=w1792) -> ("task out"=w1781:refnum<k21>, "error out"=w1780:errorcluster)  [unwired: 12 in]
                  n724 = local write "Calculate current offset"(FALSE ("Calculate current offset")) -> ()
                  n725 = Compound Arithmetic op=MULTIPLY(w1784, w1785) -> (w1783:dbl)
                  n726 = local write "Current offset"(w1783) -> ()
                }
              }
              n727 = local read "Power"() -> (w1770:bool)
              n728 = case shown="True" w1770 {
                tunnel: w1773 -> [w1824 w1842]
                tunnel: w1772 -> [w1823 w1841]
                tunnel: w1771 -> [w1822 w1830]
                tunnel: [w1824 w1829] -> w1763
                tunnel: [w1823 w1828] -> w1764
                tunnel: [w1822 w1827] -> w1765
                tunnel: [0.0 ("Readout value") w1826] -> w1769
                frame False {
                }
                frame True {
                  # "before wavelength taken from previous structure. Power reading will change before send CMD"
                  n729 = control-ref of="Zero?"() -> (w1837:refnum<vi>)
                  n730 = call "PMD Settings.vi"("Visa In"=w1842, "Zero?"=w1837, "PMD Settings In"="PM Settings", "Error In"=w1841, "Range"="Range") -> ("AUTO?"=→"AUTO?":bool, "Rng"=→"Rng":string, "Visa Out"=w1839:refnum<visa-resource-name>, "ZeroValue"=→"Zero Value":dbl, "PM Error log"=w1831:string, "error out"=w1840:errorcluster)
                  n731 = local read "Wavelength:"() -> (w1825:dbl)
                  n732 = call "PMD Get Power.vi"("VISA In"=w1839, "Wavelength (nm)"=w1825, "error in"=w1840) -> ("PMD Error"=w1832:string, "VISA out"=w1829:refnum<visa-resource-name>, "Readout value"=w1826:dbl, "error out"=w1828:errorcluster)  [unwired: 1 in, 2 out]
                  n733 = Concatenate Strings(w1830, w1831, w1832) -> (w1827:string)
                }
              }
              n734 = case shown="True" "Current" {
                tunnel: w1749 -> [w1843 w1847]
                tunnel: w1750 -> [w1844 w1848]
                tunnel: [w1845 w1849] -> w1761
                tunnel: w1769 -> [w1845 _]
                tunnel: [w1844 w1859] -> w1767
                tunnel: [w1843 w1858] -> w1766
                frame False {
                }
                frame True {
                  w1863 = 10178 items=["Finite Samples"=10178, "Continuous Samples"=10123, "Hardware Timed Single Point"=12522] ("sample mode")
                  # "Multiply AI by multiplication factor"
                  # "Calculate multipliation factor of preamp"
                  n735 = call-poly <vilib>:"DAQmx Timing.vi"("task/channels in"=w1848, "sample mode"=w1863, "samples per channel"=50, "rate"=1000.0, "error in"=w1847) -> ("task out"=w1861:refnum<k21>, "error out"=w1860:errorcluster)  [unwired: 9 in]
                  n736 = call <vilib>:"DAQmx Start Task.vi"("task/channels in"=w1861, "error in"=w1860) -> ("task out"=w1868:refnum<k21>, "error out"=w1869:errorcluster)  [unwired: 12 in]
                  n737 = local read "Preamp Sensitivity"() -> (w1854:T3)
                  n738 = local read "Lockin resource"() -> (w1855:refnum<visa-resource-name>)
                  n739 = local read "Multiply Data?"() -> (w1853:bool)
                  n740 = local read "Configuration"() -> (w1852:T4)
                  n741 = call-poly <vilib>:"DAQmx Read.vi"("task/channels in"=w1868, "error in"=w1869) -> ("task out"=w1866:refnum<k21>, "data"=w1857:dbl[], "error out"=w1867:errorcluster)  [unwired: 11 in]
                  n742 = call <vilib>:"DAQmx Stop Task.vi"("task/channels in"=w1866, "error in"=w1867) -> ("task out"=w1859:refnum<k21>, "error out"=w1858:errorcluster)  [unwired: 12 in]
                  n743 = call-poly <vilib>:"Mean.vi"("X"=w1857) -> ("mean"=w1865:dbl)  [unwired: 1 out]
                  n744 = call "Calcfactor.vi"("Preamp Sensitivity"=w1854, "Configuration 2"=w1852, "Multiply Data?"=w1853, "Lockin resource"=w1855) -> ("Multiplication Factor"=w1851:dbl)
                  "Multiplication Factor" <- w1851
                  n745 = Compound Arithmetic op=MULTIPLY(w1851, w1865) -> (w1850:dbl)
                  n746 = Wait (ms)(milliseconds to wait=u32 50) -> ()  [unwired: 1 out]
                  n747 = case shown="True" "Use Current offset" {
                    tunnel: w1850 -> [w1870 w1873]
                    tunnel: [w1870 w1871] -> w1849
                    frame False {
                    }
                    frame True {
                      n748 = Subtract(x=w1873, y="Current offset") -> (x-y=w1871:dbl)
                    }
                  }
                }
              }
              "Readout" <- w1761
              n749 = case shown="True" "On" {
                tunnel: w1761 -> [_ w1820]
                frame False {
                }
                frame True {
                  "Waveform Chart" <- w1820
                }
              }
              n750 = while {
                tunnel: "Record" -> [w1805]
                shift-right: [w1805] -> w1756
                shift-left: _ -> [w1804]
                tunnel: [w1804] -> w1758
                stop <- TRUE stop-if-true
              }
              n751 = Not Equal?(x=w1756, y=w1758) -> (x != y?=w1755:bool)
              n752 = case shown="True" w1755 {
                tunnel: w1754 -> [w1798 _]
                tunnel: [w1798 w1800] -> w1757
                frame False {
                }
                frame True {
                  w1801 = dbl[] []
                  n753 = Get Date/Time In Seconds() -> (seconds since 1Jan1904=w1802:timestamp)
                  n754 = local write "Record Start"(w1802) -> ()
                  n755 = property on="ScanGraph" class="XYGraph (strict)"("XScale.NameLbl.Text"="Time (s)" ("X Scale.Name Label.Text")) -> ()  [unwired: 2 in, 2 out]
                  n756 = Build Array(w1801, w1801) -> (w1800:dbl[][])
                }
              }
              n757 = case shown="True" w1756 {
                tunnel: w1761 -> [_ w1812]
                tunnel: w1757 -> [_ w1817]
                tunnel: [w1806 w1811] -> w1760
                tunnel: w1754 -> [w1806 _]
                frame False {
                }
                frame True {
                  n758 = local read "Record Start"() -> (w1807:timestamp)
                  n759 = Get Date/Time In Seconds() -> (seconds since 1Jan1904=w1815:timestamp)
                  n760 = Index Array(array=w1817, index (row) #1=0 ("index"), index (row) #2=1 ("index")) -> (element #1=w1813:dbl[], element #2=w1816:dbl[])  [unwired: 2 in]
                  n761 = Subtract(x=w1815, y=w1807) -> (x-y=w1814:dbl)
                  n762 = Build Array (concatenate)(w1816, w1814) -> (w1809:dbl[])
                  n763 = Build Array (concatenate)(w1813, w1812) -> (w1810:dbl[])
                  n764 = Build Array(w1810, w1809) -> (w1811:dbl[][])
                  n765 = Bundle(w1809, w1810) -> (w1808:cluster{dbl[], dbl[]})  [unwired: 1 in]
                  n766 = local write "ScanGraph"(w1808) -> ()
                }
              }
            }
            frame #2 {
              n767 = case shown="True" "Reset Params" {
                tunnel: w1878 -> [_ w1914]
                frame False {
                }
                frame True {
                  w1913 = u16 2 items=["?nm", "?nm/min", "?grating", "?turret", "?gratings"] ("Cmd")
                  # "Set parameters based \non grating"
                  n768 = control-ref of="Busy?"() -> (w1911:refnum<vi>)
                  n769 = local write "Reset Params"(FALSE ("Reset Params")) -> ()
                  n770 = call "ReadMono.vi"("Busy"=w1911, "Cmd"=w1913, "Mono Port"=w1914) -> ("Response"=w1912:string)  [unwired: 3 in, 3 out]
                  n771 = Decimal String To Number(string=w1912) -> (number=w1910:i32)  [unwired: 2 in, 1 out]
                  n772 = case shown="1, Default" w1910 {
                    frame 2 {
                      n773 = local write "Step Size (nm)"(5.0 ("Step Size (nm)")) -> ()
                      n774 = local write "Start"(1000.0 ("Start")) -> ()
                      n775 = local write "End"(1800.0 ("End")) -> ()
                    }
                    frame 1, Default {
                      n776 = local write "Step Size (nm)"(5.0 ("Step Size (nm)")) -> ()
                      n777 = local write "Start"(400.0 ("Start")) -> ()
                      n778 = local write "End"(1000.0 ("End")) -> ()
                    }
                  }
                }
              }
              n779 = case shown="True" "Scan" {
                selector: "Scan" -> [w1902 w1904]
                tunnel: [w1902 w1906] -> w1874
                frame False {
                }
                frame True {
                  n780 = local read "Saved?"() -> (w1905:bool)
                  n781 = local write "Scan"(FALSE ("Scan")) -> ()
                  n782 = case shown="True" w1905 {
                    tunnel: [w1908 w1909] -> w1906
                    tunnel: w1904 -> [_ w1909]
                    frame False {
                      n783 = Two Button Dialog(message="Not saved, continue?") -> (T button?=w1908:bool)  [unwired: 2 in]
                    }
                    frame True {
                    }
                  }
                }
              }
              n784 = Subtract(x="End", y="Start") -> (x-y=w1901:dbl)
              n785 = Divide(x=w1901, y="Step Size (nm)") -> (x/y=w1900:dbl)
              n786 = Round To Nearest(number=w1900) -> (nearest integer value=w1898:dbl)
              n787 = case shown="True" w1874 {
                tunnel: w1898 -> [_ w1997]
                tunnel: "Start" -> [_ w1995]
                tunnel: "Step Size (nm)" -> [_ w1996]
                tunnel: w1895 -> [w1925 w1987]
                tunnel: w1894 -> [w1924 w1986]
                tunnel: w1893 -> [w1926 w1960]
                tunnel: w1892 -> [w1927 w1961]
                tunnel: w1891 -> [w1928 w1993]
                tunnel: w1890 -> [w1929 w1992]
                tunnel: w1889 -> [w1930 w1990]
                tunnel: [w1926 w1983] -> w1886
                tunnel: [w1927 w1982] -> w1887
                tunnel: [w1925 w1934] -> w1884
                tunnel: [w1924 w1981] -> w1885
                tunnel: [w1928 w1980] -> w1883
                tunnel: [w1929 w1979] -> w1882
                tunnel: [w1930 w1978] -> w1888
                tunnel: [w1923 w1936] -> w1881
                tunnel: w1880 -> [w1923 _]
                tunnel: [FALSE TRUE] -> w1877
                frame False {
                }
                frame True {
                  w1935 = dbl[] []
                  w1968 = 10178 items=["Finite Samples"=10178, "Continuous Samples"=10123, "Hardware Timed Single Point"=12522] ("sample mode")
                  # "sm correction 'scan rate'"
                  # "Determine grating for sm correction"
                  # "Setup inputs/outputs"
                  n788 = Increment(x=w1997) -> (x+1=w1947:dbl)
                  n789 = call-poly <vilib>:"DAQmx Create Virtual Channel.vi"("maximum value"=10.0, "minimum value"=-10.0, "physical channels"="Scan Mirrors in") -> ("task out"=w1942:refnum<k21>, "error out"=w1941:errorcluster)  [unwired: 11 in]
                  n790 = call-poly <vilib>:"DAQmx Create Virtual Channel.vi"("maximum value"=4.0, "minimum value"=-4.0, "physical channels"="Scan mirrors out") -> ("task out"=w1970:refnum<k21>, "error out"=w1969:errorcluster)  [unwired: 11 in]
                  n791 = case shown="True" "Reset Positioned wavelength?" {
                    tunnel: w1942 -> [w2010 w2015]
                    tunnel: w1941 -> [w2009 w2016]
                    tunnel: [w2009 w2014] -> w1939
                    tunnel: [w2010 w2013] -> w1940
                    frame False {
                    }
                    frame True {
                      # "Read VNT(position of nanotube= starting position of scan)"
                      n792 = local read "Wavelength:"() -> (w2028:dbl)
                      n793 = call-poly <vilib>:"DAQmx Read.vi"("task/channels in"=w2015, "timeout"=10.0, "error in"=w2016) -> ("task out"=w2013:refnum<k21>, "data"=w2024:dbl[], "error out"=w2014:errorcluster)  [unwired: 10 in]
                      n794 = local write "Positioned Wavelength"(w2028) -> ()
                      n795 = Index Array(array=w2024, index=0) -> (element=w2022:dbl)
                      n796 = Index Array(array=w2024, index=1) -> (element=w2021:dbl)
                      n797 = Add(x=w2021, y="Sm voltage offset y") -> (x+y=w2026:dbl)
                      n798 = Add(x=w2022, y="Sm Voltage offset x") -> (x+y=w2025:dbl)
                      n799 = Negate(x=w2025) -> (-x=→"VNTx":dbl)
                      n800 = local write "Reset Positioned wavelength?"(FALSE ("Reset Positioned wavelength?")) -> ()
                      n801 = Negate(x=w2026) -> (-x=→"VNTy":dbl)
                    }
                  }
                  n802 = local read "Sm Correction?"() -> (w1933:bool)
                  n803 = local read "Current"() -> (w1994:bool)
                  n804 = Multiply(x=10, y=1000.0 ("rate")) -> (x*y=w1943:dbl)
                  n805 = Multiply(x=w1947, y=1000 ("samples per channel")) -> (x*y=w1946:dbl)
                  n806 = case shown="True" w1933 {
                    tunnel: w1961 -> [w2000 w2008]
                    tunnel: w1960 -> [w1999 w2003]
                    tunnel: [w2000 w2006] -> w1958
                    tunnel: [w1999 w2007] -> w1959
                    tunnel: [0 w2001] -> w1957
                    frame False {
                    }
                    frame True {
                      w2005 = u16 2 items=["?nm", "?nm/min", "?grating", "?turret", "?gratings"] ("Cmd")
                      n807 = control-ref of="Busy?"() -> (w2002:refnum<vi>)
                      n808 = call "ReadMono.vi"("Busy"=w2002, "error in (no error)"=w2008, "Cmd"=w2005, "Mono Port"=w2003) -> ("error out"=w2006:errorcluster, "Response"=w2004:string, "Mono Port Out"=w2007:refnum<visa-resource-name>)  [unwired: 2 in, 1 out]
                      n809 = Decimal String To Number(string=w2004) -> (number=w2001:i32)  [unwired: 2 in, 1 out]
                    }
                  }
                  n810 = case shown="True" w1994 {
                    tunnel: [w2030 w2035] -> w1989
                    tunnel: [w2029 w2034] -> w1988
                    tunnel: w1992 -> [w2029 w2033]
                    tunnel: w1993 -> [w2030 w2032]
                    tunnel: "Step Time (sec)" -> [_ w2031]
                    frame False {
                    }
                    frame True {
                      w2038 = 10178 items=["Finite Samples"=10178, "Continuous Samples"=10123, "Hardware Timed Single Point"=12522] ("sample mode")
                      w2037 = 1000.0 ("rate")
                      n811 = Compound Arithmetic op=MULTIPLY(w2031, w2037) -> (w2036:dbl)
                      n812 = call-poly <vilib>:"DAQmx Timing.vi"("task/channels in"=w2032, "sample mode"=w2038, "samples per channel"=w2036, "rate"=w2037, "error in"=w2033) -> ("task out"=w2035:refnum<k21>, "error out"=w2034:errorcluster)  [unwired: 9 in]
                    }
                  }
                  n813 = call-poly <vilib>:"DAQmx Timing.vi"("task/channels in"=w1970, "sample mode"=w1968, "samples per channel"=w1946, "rate"=w1943, "error in"=w1969) -> ("task out"=w1952:refnum<k21>, "error out"=w1950:errorcluster)  [unwired: 9 in]
                  n814 = local write "Saved?"(FALSE ("Saved?")) -> ()
                  n815 = call <vilib>:"DAQmx Start Task.vi"("task/channels in"=w1952, "error in"=w1950) -> ("task out"=w1951:refnum<k21>, "error out"=w1949:errorcluster)  [unwired: 12 in]
                  n816 = local read "VNTx"() -> (w1937:dbl)
                  n817 = local read "VNTy"() -> (w1938:dbl)
                  n818 = for {
                    N: w1947 -> [_]
                    tunnel: w1996 -> [w2101]
                    tunnel: w1995 -> [w2102]
                    shift-right: [w2094] -> w1982
                    shift-left: w1958 -> [w2096]
                    tunnel: w1959 -> [w2097]
                    tunnel: "Step Time (sec)" -> [w2092]
                    shift-right: [w2047] -> w1984
                    shift-left: w1935 -> [w2099]
                    shift-right: [w2089] -> w1985
                    shift-left: w1935 -> [w2098]
                    shift-right: [w2087] -> w1978
                    shift-left: w1990 -> [w2090]
                    shift-right: [w2041] -> w1979
                    shift-left: w1988 -> [w2069]
                    shift-right: [w2042] -> w1980
                    shift-left: w1989 -> [w2070]
                    shift-right: [w2085] -> w1981
                    shift-left: w1986 -> [w2043]
                    tunnel: w1987 -> [w2044]
                    tunnel: [w2095] -> w1983
                    tunnel: [w2086] -> w1934
                    tunnel: [FALSE ("Tabs Visible?")] -> w1977
                    tunnel: w1938 -> [w2065]
                    tunnel: w1937 -> [w2064]
                    tunnel: [w2048] -> w1956
                    shift-right: [w2082] -> w1954
                    shift-left: w1949 -> [w2081]
                    tunnel: w1951 -> [w2080]
                    shift-right: [w2073] -> w1967
                    shift-left: w1939 -> [w2072]
                    shift-right: [w2071] -> w1966
                    shift-left: w1940 -> [w2083]
                    tunnel: "Sm Correction?" -> [w2063]
                    tunnel: w1957 -> [w2062]
                    i -> [w2100]
                    stop <- "STOP" stop-if-true
                    # "Have mirrors move before taking data"
                    # "Display in nm or eV"
                    # "Read after writing"
                    n819 = Compound Arithmetic op=MULTIPLY(w2101, w2100) -> (w2103:dbl)
                    n820 = Compound Arithmetic op=ADD(w2102, w2103) -> (w2053:dbl)
                    n821 = case shown="True" w2063 {
                      tunnel: w2083 -> [w2115 w2160]
                      tunnel: [w2113 w2116] -> w2048
                      tunnel: [w2112 w2117] -> w2082
                      tunnel: w2081 -> [w2112 w2135]
                      tunnel: w2080 -> [w2113 w2134]
                      tunnel: [w2114 w2157] -> w2074
                      tunnel: w2072 -> [w2114 w2156]
                      tunnel: [w2115 w2155] -> w2067
                      tunnel: w2053 -> [_ w2122]
                      tunnel: w2065 -> [_ w2152]
                      tunnel: w2064 -> [_ w2151]
                      tunnel: w2062 -> [_ w2137]
                      frame False {
                      }
                      frame True {
                        # "At some point measure directly AO/AI offset"
                        # "Wait for scan mirrors to move"
                        # "y is inverted"
                        # "Monitor array being sent to write"
                        # "Write"
                        # "Calc deltaV"
                        # "VNT' = VNT + DeltaV"
                        # "Generate saw waves"
                        # "Correct for AO/AI offset"
                        # "Read current location"
                        n822 = local read "Positioned Wavelength"() -> (w2123:dbl)
                        n823 = case shown="1, Default" w2137 {
                          tunnel: ["Vis Grating Correction" "IR Grating Correction"] -> w2126
                          tunnel: ["Vis Grating" "IR Grating"] -> w2136
                          frame 1, Default {
                          }
                          frame 2 {
                          }
                        }
                        "String" <- w2136
                        n824 = call-poly <vilib>:"DAQmx Read.vi"("task/channels in"=w2160, "error in"=w2156) -> ("task out"=w2155:refnum<k21>, "data"=w2163:dbl[], "error out"=w2157:errorcluster)  [unwired: 11 in]
                        n825 = local read "Sm voltage offset y"() -> (w2119:dbl)
                        n826 = call "CalcdeltaV.vi"("Correction"=w2126, "nm0"=w2123, "nm in"=w2122, "Volts/pixel y"="Volts/pixel y", "Volts/pixel  x"="Volts/pixel  x") -> ("DeltaVy"=w2121:dbl, "Delta Pix y"=→"Delta Pix y":dbl, "delta pix x"=→"delta pix x":dbl, "DeltaVx"=w2150:dbl)
                        n827 = local read "Sm Voltage offset x"() -> (w2120:dbl)
                        n828 = Index Array(array=w2163, index=0) -> (element=w2162:dbl)
                        n829 = Index Array(array=w2163, index=1) -> (element=w2161:dbl)
                        n830 = Add(x=w2150, y=w2151) -> (x+y=w2149:dbl)
                        n831 = Add(x=w2119, y=w2161) -> (x+y=w2129:dbl)
                        n832 = Add(x=w2121, y=w2152) -> (x+y=w2127:dbl)
                        n833 = Add(x=w2120, y=w2162) -> (x+y=w2131:dbl)
                        n834 = Negate(x=w2131) -> (-x=w2130:dbl)
                        n835 = Negate(x=w2129) -> (-x=w2128:dbl)
                        n836 = call "Generate Saw.vi"("V in y"=w2128, "V in x"=w2130, "VNT'y"=w2127, "VNT'x"=w2149) -> ("V out y"=w2139:dbl[], "V out x"=w2138:dbl[])
                        "Waveform Chart X" <- w2138
                        "Waveform Chart  Y" <- w2139
                        n837 = Build Array(w2138, w2139) -> (w2148:dbl[][])
                        n838 = call-poly <vilib>:"DAQmx Write.vi"("task/channels in"=w2134, "data"=w2148, "timeout"=-1.0, "error in"=w2135) -> ("task out"=w2133:refnum<k21>, "number of samples written per channel"=→"number of samples written per channel":u32, "error out"=w2132:errorcluster)  [unwired: 9 in]
                        n839 = Get Date/Time In Seconds() -> (seconds since 1Jan1904=w2118:timestamp)
                        n840 = while {
                          tunnel: w2133 -> [w2167]
                          tunnel: w2132 -> [w2166]
                          tunnel: w2118 -> [w2171]
                          tunnel: [w2167] -> w2116
                          tunnel: [w2166] -> w2117
                          stop <- w2168 stop-if-true
                          n841 = Get Date/Time In Seconds() -> (seconds since 1Jan1904=w2172:timestamp)
                          n842 = Subtract(x=w2172, y=w2171) -> (x-y=w2170:dbl)
                          n843 = Greater Or Equal?(x=w2170, y=0.2 ("milliseconds to wait")) -> (x >= y?=w2168:bool)
                        }
                        n844 = Index Array(array=w2139, index #1=0 ("index"), index #2=999 ("index")) -> (element #1=→"initial y":dbl, element #2=→"Final Y":dbl)
                        n845 = Index Array(array=w2138, index #1=0 ("index"), index #2=999 ("index")) -> (element #1=→"initial x":dbl, element #2=→"Final x":dbl)
                      }
                    }
                    n846 = local write "Wavelength:"(w2053) -> ()
                    n847 = Unbundle("PEM100Setup") -> ("Address:"=w2051:T2, "Retardation:"=w2056:dbl, "RTD Units"=w2055:u16, "Wave Units"=w2054:u16)  [unwired: 1 out]
                    n848 = Bundle("Address:"=w2051, "Retardation:"=w2056, "RTD Units"=w2055, w2053, "Wave Units"=w2054) -> (w2052:T12)  [unwired: 1 in]
                    n849 = local write "PEM100Setup"(w2052) -> ()
                    n850 = flat-sequence {
                      tunnel: w2097 -> [w2195]
                      tunnel: w2096 -> [w2194]
                      tunnel: w2053 -> [w2182]
                      tunnel: [w2187] -> w2095
                      tunnel: [w2186] -> w2094
                      tunnel: [w2183] -> w2093
                      tunnel: [w2182] -> w2091
                      tunnel: [w2181] -> w2068
                      tunnel: w2067 -> [w2181]
                      tunnel: w2052 -> [w2180]
                      tunnel: w2092 -> [w2231]
                      tunnel: w2091 -> [w2233]
                      tunnel: w2090 -> [w2230]
                      tunnel: [w2216] -> w2040
                      tunnel: [w2228] -> w2087
                      tunnel: [w2227] -> w2086
                      tunnel: [w2226] -> w2085
                      tunnel: w2070 -> [w2225]
                      tunnel: w2069 -> [w2224]
                      tunnel: [w2223] -> w2042
                      tunnel: [w2222] -> w2041
                      tunnel: w2068 -> [w2221]
                      tunnel: [w2221] -> w2066
                      tunnel: w2044 -> [w2218]
                      tunnel: w2043 -> [w2219]
                      frame #0 {
                        w2188 = u16 0 items=["?nm", "?nm/min", "?grating", "?turret", "?gratings"] ("Cmd")
                        w2193 = u16 1 items=["nm", "goto", "nm/min", "VIS grating", "IR grating"] ("Cmd")
                        n851 = control-ref of="Busy?"() -> (w2192:refnum<vi>)
                        n852 = call "CmdMono.vi"("Busy"=w2192, "error in (no error)"=w2194, "Wavelength (nm)"=w2182, "Cmd"=w2193, "Mono Port"=w2195) -> ("error out"=w2191:errorcluster, "Response"=w2189:string, "Mono Port Out"=w2190:refnum<visa-resource-name>)  [unwired: 3 in, 1 out]
                        n853 = local write "Done?"(w2189) -> ()
                        n854 = call "ReadMono.vi"("Busy"=w2192, "error in (no error)"=w2191, "Cmd"=w2188, "Mono Port"=w2190) -> ("error out"=w2186:errorcluster, "Response"=w2178:string, "Mono Port Out"=w2187:refnum<visa-resource-name>)  [unwired: 2 in, 1 out]
                        n855 = case shown="True" "Use PEM?" {
                          tunnel: w2180 -> [_ w2204]
                          tunnel: [w2196 w2200] -> w2179
                          tunnel: w2178 -> [w2196 w2199]
                          frame False {
                          }
                          frame True {
                            n856 = while {
                              tunnel: w2204 -> [w2211]
                              tunnel: [w2211] -> w2203
                              tunnel: [w2209] -> w2197
                              tunnel: [w2208] -> w2200
                              tunnel: w2199 -> [w2208]
                              stop <- TRUE stop-if-true
                              n857 = Get Date/Time In Seconds() -> (seconds since 1Jan1904=w2209:timestamp)
                            }
                            n858 = call "HindsPEM100_Setup.vi"("PEM100Setup"=w2203) -> ("error out"=w2202:errorcluster)  [unwired: 18 in]
                            n859 = while {
                              tunnel: w2202 -> [w2207]
                              tunnel: [w2207] -> _
                              tunnel: [w2205] -> w2198
                              stop <- TRUE stop-if-true
                              n860 = Get Date/Time In Seconds() -> (seconds since 1Jan1904=w2205:timestamp)
                            }
                            n861 = Subtract(x=w2198, y=w2197) -> (x-y=→"PEM delay":dbl)
                          }
                        }
                        n862 = Match Pattern(string=w2179, regular expression=" nm") -> (before substring=w2185:string)  [unwired: 1 in, 3 out]
                        n863 = Fract/Exp String To Number(string=w2185) -> (number=w2183:dbl)  [unwired: 3 in, 1 out]
                        n864 = local write "Reply"(w2178) -> ()
                      }
                      frame #1 {
                        n865 = Get Date/Time In Seconds() -> (seconds since 1Jan1904=w2232:timestamp)
                        n866 = local read "Use Current offset"() -> (w2215:bool)
                        n867 = local read "Power"() -> (w2213:bool)
                        n868 = case shown="False" "Power" {
                          tunnel: dbl[] [] -> [_ w2275]
                          tunnel: w2218 -> [w2261 w2274]
                          tunnel: w2219 -> [w2260 w2273]
                          tunnel: w2233 -> [_ w2272]
                          tunnel: w2232 -> [_ w2271]
                          tunnel: w2231 -> [w2241 w2270]
                          tunnel: w2230 -> [_ w2269]
                          tunnel: ["" w2268] -> w2228
                          tunnel: [w2249 w2267] -> w2229
                          tunnel: [w2261 w2266] -> w2227
                          tunnel: [w2260 w2265] -> w2226
                          tunnel: w2225 -> [w2259 w2264]
                          tunnel: w2224 -> [w2258 w2263]
                          tunnel: [w2251 w2264] -> w2223
                          tunnel: [w2250 w2263] -> w2222
                          frame False {
                            n869 = Multiply(x=w2241, y=1000) -> (x*y=w2242:dbl)
                            n870 = local read "Preamp Sensitivity"() -> (w2246:T3)
                            n871 = local read "Lockin resource"() -> (w2245:refnum<visa-resource-name>)
                            n872 = local read "Multiply Data?"() -> (w2244:bool)
                            n873 = local read "Configuration"() -> (w2243:T4)
                            n874 = Wait (ms)(milliseconds to wait=w2242) -> ()  [unwired: 1 out]
                            n875 = call <vilib>:"DAQmx Start Task.vi"("task/channels in"=w2259, "error in"=w2258) -> ("task out"=w2252:refnum<k21>, "error out"=w2253:errorcluster)  [unwired: 12 in]
                            n876 = call "Calcfactor.vi"("Preamp Sensitivity"=w2246, "Configuration 2"=w2243, "Multiply Data?"=w2244, "Lockin resource"=w2245) -> ("Multiplication Factor"=w2247:dbl)
                            n877 = call-poly <vilib>:"DAQmx Read.vi"("task/channels in"=w2252, "error in"=w2253) -> ("task out"=w2255:refnum<k21>, "data"=w2257:dbl[][], "error out"=w2254:errorcluster)  [unwired: 11 in]
                            n878 = Index Array(array=w2257, index (row)=0) -> (element=w2248:dbl[])  [unwired: 1 in]
                            n879 = call <vilib>:"DAQmx Stop Task.vi"("task/channels in"=w2255, "error in"=w2254) -> ("task out"=w2251:refnum<k21>, "error out"=w2250:errorcluster)  [unwired: 12 in]
                            n880 = Compound Arithmetic op=MULTIPLY(w2248, w2247) -> (w2249:dbl[])
                          }
                          frame True {
                            n881 = while {
                              shift-right: [w2283] -> w2267
                              shift-left: w2275 -> [w2284]
                              tunnel: w2274 -> [w2291]
                              tunnel: w2272 -> [w2289]
                              tunnel: w2271 -> [w2288]
                              tunnel: w2270 -> [w2286]
                              shift-right: [w2281] -> w2265
                              shift-left: w2273 -> [w2290]
                              tunnel: [w2280] -> w2266
                              shift-right: [w2277] -> w2268
                              shift-left: w2269 -> [w2279]
                              stop <- w2276 stop-if-true
                              n882 = Get Date/Time In Seconds() -> (seconds since 1Jan1904=w2285:timestamp)
                              n883 = Subtract(x=w2285, y=w2288) -> (x-y=w2287:dbl)
                              n884 = Greater Or Equal?(x=w2287, y=w2286) -> (x >= y?=w2276:bool)
                              n885 = call "PMD Get Power.vi"("VISA In"=w2291, "Wavelength (nm)"=w2289, "error in"=w2290) -> ("PMD Error"=w2278:string, "VISA out"=w2280:refnum<visa-resource-name>, "Readout value"=w2282:dbl, "error out"=w2281:errorcluster)  [unwired: 1 in, 2 out]
                              n886 = Build Array (concatenate)(w2284, w2282) -> (w2283:dbl[])
                              n887 = Concatenate Strings(w2279, w2278) -> (w2277:string)
                            }
                          }
                        }
                        n888 = Not(x=w2213) -> (.not. x?=w2212:bool)
                        n889 = And(x=w2215, y=w2212) -> (x .and. y?=w2214:bool)
                        n890 = call-poly <vilib>:"Mean.vi"("X"=w2229) -> ("mean"=w2217:dbl)  [unwired: 1 out]
                        n891 = case shown="True" w2214 {
                          tunnel: w2217 -> [w2236 w2239]
                          tunnel: [w2236 w2237] -> w2216
                          frame False {
                          }
                          frame True {
                            n892 = local read "Current offset"() -> (w2238:dbl)
                            n893 = Subtract(x=w2239, y=w2238) -> (x-y=w2237:dbl)
                          }
                        }
                        "Measuring?" <- TRUE ("Measuring?")
                      }
                    }
                    n894 = while {
                      tunnel: [w2110] -> _
                      tunnel: w2040 -> [w2109]
                      tunnel: [w2109] -> w2039
                      stop <- TRUE stop-if-true
                      w2110 = FALSE ("Measuring?")
                      n895 = local write "Measuring?"(w2110) -> ()
                    }
                    n896 = call-poly <vilib>:"DAQmx Read.vi"("task/channels in"=w2066, "error in"=w2074) -> ("task out"=w2071:refnum<k21>, "data"=w2077:dbl[], "error out"=w2073:errorcluster)  [unwired: 11 in]
                    n897 = Build Array (concatenate)(w2099, w2093) -> (w2047:dbl[])
                    n898 = Build Array (concatenate)(w2098, w2039) -> (w2089:dbl[])
                    n899 = local write "Readout"(w2039) -> ()
                    n900 = local read "Sm Voltage offset x"() -> (w2050:dbl)
                    n901 = local read "Sm voltage offset y"() -> (w2049:dbl)
                    n902 = Index Array(array=w2077, index=0) -> (element=w2075:dbl)
                    n903 = Index Array(array=w2077, index=1) -> (element=w2076:dbl)
                    n904 = case shown="False" "eV" {
                      tunnel: w2047 -> [w2106 w2108]
                      tunnel: [w2105 w2108] -> w2046
                      frame False {
                        n905 = Divide(x=1240.0, y=w2106) -> (x/y=w2105:dbl[])
                      }
                      frame True {
                      }
                    }
                    n906 = Add(x=w2050, y=w2075) -> (x+y=w2061:dbl)
                    n907 = Add(x=w2049, y=w2076) -> (x+y=w2059:dbl)
                    n908 = Negate(x=w2061) -> (-x=→"x after move":dbl)
                    n909 = Negate(x=w2059) -> (-x=→"y after move":dbl)
                    n910 = local write "PM Error log"(w2087) -> ()
                    n911 = Bundle(w2046, w2089) -> (→"ScanGraph":cluster{dbl[], dbl[]})  [unwired: 1 in]
                  }
                  n912 = local write "Scan"(w1977) -> ()
                  n913 = call <vilib>:"DAQmx Stop Task.vi"("task/channels in"=w1956, "error in"=w1954) -> ("task out"=w1955:refnum<k21>, "error out"=w1953:errorcluster)  [unwired: 12 in]
                  n914 = call <vilib>:"DAQmx Stop Task.vi"("task/channels in"=w1966, "error in"=w1967) -> ("task out"=w1965:refnum<k21>, "error out"=w1964:errorcluster)  [unwired: 12 in]
                  n915 = Build Array(w1985, w1984) -> (w1936:dbl[][])
                  n916 = call <vilib>:"DAQmx Clear Task.vi"("task in"=w1955, "error in"=w1953) -> ()  [unwired: 13 in, 1 out]
                  n917 = call <vilib>:"DAQmx Clear Task.vi"("task in"=w1965, "error in"=w1964) -> ()  [unwired: 13 in, 1 out]
                }
              }
            }
          }
          "PM Error log" <- w1480
          n918 = local read "Power Meter Initalized?"() -> (w1459:bool)
          n919 = local read "Power"() -> (w1460:bool)
          n920 = local read "eV"() -> (w1442:bool)
          n921 = local read "Exit"() -> (w1478:bool)
          n922 = Not(x=w1460) -> (.not. x?=w1458:bool)
          n923 = while {
            tunnel: w1442 -> [w1527]
            shift-right: [w1527] -> w1440
            shift-left: _ -> [w1526]
            tunnel: [w1526] -> w1441
            tunnel: "Normalize?" -> [w1524]
            shift-right: [w1524] -> w1423
            shift-left: _ -> [w1523]
            tunnel: [w1523] -> w1430
            stop <- TRUE stop-if-true
          }
          n924 = call "generate filepath.vi"("Filename"="Filename", "Subfolder(no outside slashes)"="Subfolder(no outside slashes)", "Prepend date folder?"="Prepend date folder?", "Scan base"="Scan base") -> ("path"=w1448:path)
          n925 = And(x=w1459, y=w1458) -> (x .and. y?=w1457:bool)
          n926 = case shown="True" w1457 {
            tunnel: w1455 -> [w1587 w1589]
            tunnel: w1456 -> [w1586 w1590]
            tunnel: [w1587 w1589] -> w1454
            tunnel: [w1586 w1590] -> w1453
            frame False {
            }
            frame True {
              # "PM"
              n927 = local write "Power Meter Initalized?"(FALSE ("Power Meter Initalized?")) -> ()
              n928 = call "PM100D_Close.vi"("error in (no error)"=w1590, "VISA resource name"=w1589) -> ()  [unwired: 2 in]
            }
          }
          n929 = Not Equal?(x=w1441, y=w1440) -> (x != y?=w1429:bool)
          n930 = call <vilib>:"Check if File or Folder Exists.vi"("path"=w1448) -> ("file or folder exists?"=w1449:bool, "dup path"=w1450:path)  [unwired: 8 in, 1 out]
          n931 = Not Equal?(x=w1423, y=w1430) -> (x != y?=w1424:bool)
          n932 = Compound Arithmetic op=OR(w1429, w1428, w1424) -> (w1427:bool)
          n933 = case shown="True" w1428 {
            tunnel: w1426 -> [_ w1508]
            tunnel: [w1499 w1500] -> w1425
            tunnel: w1433 -> [w1499 _]
            frame False {
            }
            frame True {
              n934 = Index Array(array=w1508, index (row) #1=1 ("index (row)"), index (row) #2=0 ("index (row)")) -> (element #1=w1501:dbl[], element #2=w1504:dbl[])  [unwired: 2 in]
              n935 = local read "Vis Power"() -> (w1506:dbl[][])
              n936 = call "Getpower.vi"("Wavlength array"=w1501, "Normalizing power wave"=w1506) -> ("Power array out"=w1503:dbl[])
              n937 = Divide(x=w1504, y=w1503) -> (x/y=w1502:dbl[])
              n938 = Build Array(w1502, w1501) -> (w1500:dbl[][])
            }
          }
          n939 = case shown="False" w1449 {
            tunnel: w1450 -> [w1577 w1585]
            tunnel: [w1577 w1581] -> w1444
            tunnel: "Filename" -> [_ w1580]
            frame False {
            }
            frame True {
              # "add x to filename if exists"
              n940 = Path To String(path=w1585) -> (string=w1584:string)
              n941 = Concatenate Strings(w1580, "x" ("string")) -> (w1578:string)
              n942 = Concatenate Strings(w1584, "x" ("string")) -> (w1582:string)
              n943 = local write "Filename"(w1578) -> ()
              n944 = String To Path(string=w1582) -> (path=w1581:path)
            }
          }
          "path" <- w1444
          n945 = Compound Arithmetic op=OR("Switch to Imaging", w1478) -> (w1479:bool)
          n946 = Wait (ms)(milliseconds to wait=u32 50) -> ()  [unwired: 1 out]
          n947 = case shown="False" w1423 {
            tunnel: w1425 -> [_ w1498]
            tunnel: [w1497 w1498] -> w1432
            tunnel: w1426 -> [w1497 _]
            frame False {
            }
            frame True {
            }
          }
          n948 = case shown="True" w1427 {
            tunnel: w1432 -> [_ w1536]
            tunnel: w1423 -> [_ w1528]
            frame False {
            }
            frame True {
              # "Display in nm or eV"
              n949 = case shown="True" w1528 {
                frame True {
                  n950 = property on="ScanGraph" class="XYGraph (strict)"("YScale.NameLbl.Text"="Normalized Current(A/W)" ("X Scale.Name Label.Text")) -> ()  [unwired: 2 in, 2 out]
                }
                frame False {
                  n951 = property on="ScanGraph" class="XYGraph (strict)"("YScale.NameLbl.Text"="Unnormalized current(A)" ("X Scale.Name Label.Text")) -> ()  [unwired: 2 in, 2 out]
                }
              }
              n952 = local read "eV"() -> (w1532:bool)
              n953 = Index Array(array=w1536, index (row) #1=1 ("index"), index (row) #2=0 ("index (col)")) -> (element #1=w1534:dbl[], element #2=w1530:dbl[])  [unwired: 2 in]
              n954 = case shown="True" w1532 {
                tunnel: w1534 -> [w1541 w1544]
                tunnel: [w1540 w1544] -> w1529
                frame False {
                  n955 = property on="ScanGraph" class="XYGraph (strict)"("XScale.NameLbl.Text"="Photon Energy (eV)" ("X Scale.Name Label.Text")) -> ()  [unwired: 2 in, 2 out]
                  n956 = Divide(x=1240.0, y=w1541) -> (x/y=w1540:dbl[])
                }
                frame True {
                  n957 = property on="ScanGraph" class="XYGraph (strict)"("XScale.NameLbl.Text"="Wavelength (nm)" ("X Scale.Name Label.Text")) -> ()  [unwired: 2 in, 2 out]
                }
              }
              n958 = Bundle(w1529, w1530) -> (w1531:cluster{dbl[], dbl[]})  [unwired: 1 in]
              n959 = local write "ScanGraph"(w1531) -> ()
            }
          }
          n960 = property on="ScanGraph" class="XYGraph (strict)"() -> ("XScale.NameLbl.Text"=w1437:string)  [unwired: 2 in, 2 out]
          n961 = case shown="\"Wavelength (nm)\"" w1437 {
            selector: w1437 -> [w1510 w1516 w1522]
            tunnel: [w1509 w1513 w1519] -> w1436
            tunnel: w1426 -> [_ w1511 w1517]
            tunnel: w1435 -> [w1509 _ _]
            tunnel: w1425 -> [_ w1515 w1521]
            frame "Time (s)" {
              "Data stream" <- w1510
            }
            frame "Photon Energy (eV)", Default {
              n962 = local write "Data stream"(w1516) -> ()
              n963 = Index Array(array=w1515, index (row)=0) -> (element=w1512:dbl[])  [unwired: 1 in]
              n964 = Build Array (concatenate)(w1512, w1511) -> (w1513:dbl[][])
            }
            frame "Wavelength (nm)" {
              n965 = local write "Data stream"(w1522) -> ()
              n966 = Index Array(array=w1521, index (row)=0) -> (element=w1518:dbl[])  [unwired: 1 in]
              n967 = Build Array (concatenate)(w1518, w1517) -> (w1519:dbl[][])
            }
          }
          n968 = case shown="True" "Save" {
            tunnel: w1436 -> [_ w1553]
            tunnel: w1444 -> [_ w1548]
            frame False {
            }
            frame True {
              n969 = stacked-sequence {
                seq-local: [w1556 _] -> [_ w1562]
                tunnel: "" -> [w1558 _]
                tunnel: [_ w1561] -> w1547
                frame #0 {
                  n970 = local read "Lockin resource"() -> (w1557:refnum<visa-resource-name>)
                  n971 = call "Read Lockin.vi"("VISA resource name"=w1557, "String"=w1558) -> ("String 2"=w1556:string)
                }
                frame #1 {
                  n972 = local read "Normalizing power visible"() -> (w1560:path)
                  n973 = local read "Normalizing power IR"() -> (w1559:path)
                  n974 = local read "Use Current offset"() -> (w1566:bool)
                  n975 = property on="ScanGraph" class="XYGraph (strict)"() -> ("XScale.NameLbl.Text"=w1563:string)  [unwired: 2 in, 2 out]
                  n976 = local read "Preamp Bias (mv)"() -> (w1569:i32)
                  n977 = property on="ScanGraph" class="XYGraph (strict)"() -> ("YScale.NameLbl.Text"=w1564:string)  [unwired: 2 in, 2 out]
                  n978 = local read "Output 2"() -> (w1570:dbl)
                  n979 = local read "Preamp Bias on?"() -> (w1568:bool)
                  n980 = local read "Current offset"() -> (w1565:dbl)
                  n981 = local read "Multiply Data?"() -> (w1575:bool)
                  n982 = local read "Preamp Sensitivity"() -> (w1573:T3)
                  n983 = local read "Step Time (sec)"() -> (w1572:dbl)
                  n984 = local read "Output 1"() -> (w1571:dbl)
                  n985 = local read "Wavelength:"() -> (w1567:dbl)
                  n986 = local read "Configuration"() -> (w1574:T4)
                  n987 = Bundle("Multiply Data?"=w1575, "Configuration"=w1574, "Preamp Sensitivity"=w1573, "Step Time (sec)"=w1572, "Output 1"=w1571, "Output 2"=w1570, "Preamp Bias (mv)"=w1569, "Preamp Bias on?"=w1568, "Wavelength:"=w1567, "Use Current offset"=w1566, "Current offset"=w1565, "YScale.NameLbl.Text"=w1564, "XScale.NameLbl.Text"=w1563, "Normalizing power visible"=w1560, "Normalizing power IR"=w1559) -> (w1576:T13)  [unwired: 1 in]
                  n988 = call "Header_CF.vi"("Cluster"=w1576, "String in"=w1562) -> ("String out"=w1561:string)
                }
              }
              n989 = local write "Save"(FALSE ("Save")) -> ()
              n990 = Write to Text File(file (use dialog)=w1548, text=w1547) -> (refnum out=w1546:refnum<file>)  [unwired: 2 in, 2 out]
              n991 = Refnum to Path(1:w1546) -> (0:w1545:path)
              n992 = call-poly <vilib>:"Write To Spreadsheet File.vi"("transpose? (no:F)"=TRUE, "format (%.3f)"="%#.3e", "append to file? (new file:F)"=TRUE, "2D data"=w1553, "file path (dialog if empty)"=w1545) -> ()  [unwired: 3 in, 1 out]
              n993 = local write "Saved?"(TRUE ("Saved?")) -> ()
            }
          }
        }
        n994 = case shown="False" w1404 {
          tunnel: [enum32{"Imaging", "Spectral"}."Spectral" ("Tab Control") w1422] -> w1403
          frame False {
          }
          frame True {
            w1422 = enum32{"Imaging", "Spectral"}."Imaging" ("Tab Control")
            n995 = property on="Tab Control" class="TabCtl (strict)"("Value"=w1422) -> ()  [unwired: 2 in, 2 out]
          }
        }
        n996 = call <vilib>:"DAQmx Clear Task.vi"("task in"=w1416, "error in"=w1417) -> ()  [unwired: 13 in, 1 out]
        n997 = call <vilib>:"DAQmx Clear Task.vi"("task in"=w1419, "error in"=w1418) -> ()  [unwired: 13 in, 1 out]
        n998 = call <vilib>:"DAQmx Clear Task.vi"("task in"=w1410, "error in"=w1411) -> ()  [unwired: 13 in, 1 out]
        "Busy?" <- FALSE ("Busy?")
      }
    }
    n999 = VISA Close(VISA resource name=w50, error in (no error)=w51) -> (error out=w52:errorcluster)
    n1000 = call <vilib>:"Simple Error Handler.vi"("error in (no error)"=w52) -> ()  [unwired: 1 in, 8 out]
  }
  n1001 = local write "Exit"(w4) -> ()
  "Saved?" <- FALSE ("Saved?")
